vi "Laser Spectroscopy.vi"() -> ()   [LabVIEW 2014]
uses:
  Control 3.ctl
  Control 4.ctl
  Source Cluster.ctl
  MoCo Source Code LabView 2013/global_m.vi
  <instrlib>/Tektronix DPO 7104/Tektronix 7000 Series/Public/Configure/Configure Trigger (Edge).vi
  <instrlib>/Tektronix DPO 7104/Tektronix 7000 Series/Public/Data/Read (Single Waveform).vi
  <vilib>/NI/GXML/Generator.vi
  <vilib>/NI/GXML/Write XML to File.vi
  <vilib>/Utility/file.llb/Write To Spreadsheet File (DBL).vi
  <instrlib>/Tektronix 7000 Series/Tektronix 7000 Series.lvlib
  C8855-01api.dll
panel:
  out "Waveform Graph C8855":waveform(dbl)(graph)
  out "Refnum out":refnum<k7> caption="Mono RefNum out"
  out "XY Graph":cluster{"Wavelength":dbl[], "Int WF":dbl[]}(graph)
  in  "Reinitialise to default values":bool
  out "Waveform Graph":waveform(dbl)(graph)
  in  "Tab Control":T1(tab)
  out "state":dbl
  in  "Target Grating":u16(ring)=1 items=["1200", "600", "300"]
  in  "Clear data array":bool
  in  "Abort Scan":bool
  in  "Operator's Name":string="Operator"
  in  "File Format":enum16{"XML", "CSV"}(ring)
  in  "Log Data":bool
  in  "Path":path
  in  "Backward":bool
  in  "Forward":bool
  in  "Scan Mode":enum32{"Interrupted ", "Uninterrupted"}(radio)=enum."Uninterrupted"
  in  "Scan":bool
  in  "Target WL":bool
  in  "End Wavelength":dbl=572.0
  in  "Delay (s)":dbl
  in  "Interval Wavelength":dbl=0.1
  in  "Start Wavelength":dbl=882.0
  in  "Target WL":dbl=882.7202
  in  "Exit Mirror":u16(ring)=2 caption="Target Position Exit Mirror" items=["Front"=2, "Side"=3]
  in  "Entrance Mirror":u16(ring)=2 caption="Target Position\nEntrance Mirror" items=["Front"=2, "Side"=3]
  in  "Target  Exit":dbl
  in  "Target\nFront Entrance":dbl
  out "Current Grating":dbl=1200.0
  out "Grating Index":i32=1
  out "Current Description":string="1" caption="Description"
  in  "Mono ID":string(combo)="Mono4"
  out "Current UniqueID":string="Mono4"
  out "Current WL":dbl=897.9988
  out "Exit":dbl
  out "Unit":string="mm"
  out "Front Entrance":dbl
  out "Unit":string="mm"
  out "Exit Mirror\nPosition":i32(ring)=2 items=["EntranceMirror", "ExitMirror", "Front", "Side"]
  out "Entrance Mirror\nPosition":i32(ring)=2 items=["EntranceMirror", "ExitMirror", "Front", "Side"]
  in  "Force\nInitialization":bool
  out "Unit":string="nm"
  in  "Connect":bool
  out "iHR550 Error Bundle":errorcluster
  out "Emulating":bool
  out "Initialized":bool
  out "Status":string
  out "error out":errorcluster
  out "source out 2":string
  out "code out":i32 format="%0.0f"
  out "Gratings":dbl[](array[numeric])=[1200.0, 300.0]
  out "Current Blaze":string
  out "Medium Loop":T2
  out "DPO7104":T3=enum."Initial Settings"
  in  "stop":bool
  in  "Close Session":bool
  in  "Initialize":bool caption="Push at the start"
  in  "Auto Calibration:":bool
  in  "Save GL302 Settings":bool
  in  "Backlash Compensation":bool
  in  "Calibration":bool
  in  "Set speed":bool
  in  "stop 2":bool
  in  "fs":bool
  in  "bs":bool
  in  "FW":bool
  in  "BW":bool
  in  "Pause":dbl
  in  "Abort Scan GL302":bool
  in  "Step":dbl
  in  "Scan GL302":bool
  in  "End Wavelength":dbl min=-20.0 max=1100.0
  in  "Start Wavelength":dbl min=-20.0 max=1100.0
  in  "Target Wavelength":bool
  in  "Calibration, nm":dbl=587.2
  in  "Destination Wavelength":dbl min=-20.0 max=1100.0 format="%.3f"
  in  "Grating, gr/mm":u16(ring)=2 items=["2400", "1800", "1200", "600", "300", "150"]
  in  "delay before read (ms)":u32=100
  in  "Scan Mode":enum32{"Interrupted ", "Uninterrupted"}(radio)=enum."Uninterrupted"
  out "Present Wavelength":dbl=479.168125 format="%.3f"
  in  "Wavelength, nm":dbl format="%.3f"
  in  "Speed":dbl=5.0 format="%.3f"
  out "R number":i32
  in  "Backlash Compensation":dbl=0.01 format="%.3f"
  out "GL302 Initialization":errorcluster
  out "Communication Port":refnum<visa-resource-name>
  out "Status":string
  in  "shutdown":bool
  in  "stop curving":bool
  in  "Integrate":bool=TRUE
  out "CURV?":bool
  in  "Channel (0: Channel 1)":u16(ring)=1 format="%#_5f" items=["Channel 1", "Channel 2", "Channel 3", "Channel 4", "Math 1", "Math 2", "Math 3", "Math 4", "Reference 1", "Reference 2", "Reference 3", "Reference 4"]
  in  "AUTOSET":bool
  in  "Delay Time":dbl
  in  "Delay":bool
  in  "# of Averages":u32=16
  in  "Acquisition Mode":enum16{"Sample", "Average", "Hi Res"}(ring)=enum."Average"
  in  "Probe Attenuation (10.0)":dbl=1.0 step=0.5
  in  "Vertical Coupling (1: DC)":u16(ring)=1 items=["AC", "DC", "Ground"]
  in  "Trigger Level (0.0)":dbl=0.08
  in  "Input Impedance":u16(ring)=1 items=["1M", "50"]
  in  "Bandwidth (0: FULL)":u16(ring) items=["FULL", "500 MHz", "250 MHz", "150 MHz", "20 MHz"]
  in  "Delay Position":u32
  in  "Vertical Position":dbl step=0.5
  in  "Vertical Offset (0.0 V)":dbl
  in  "Position (0.0 s)":dbl=10.0
  in  "Coupling (0:DC)":u16(ring)=1 items=["DC", "AC", "Hf Reject", "Lf Reject", "Noise Rej", "Atrigger"]
  in  "Trigger Event (0:A Event)":u16(ring) items=["A Event", "B Event"]
  in  "Slope (0:Rise)":u16(ring) items=["Rise", "Fall", "Either"]
  in  "Source (0:Channel1)":u16(ring) items=["Channel1"=0, "Channel2"=1, "Channel3"=2, "Channel4"=3, "Aux"=12, "Line"=13, "Digital Channel0"=14, "Digital Channel1"=15, "Digital Channel2"=16, "Digital Channel3"=17, "Digital Channel4"=18, "Digital Chennel5"=19, "Digital Channel6"=20, "Digital Channel7"=21, "Digital Channel8"=22, "Digital Channel9"=23, "Digital Channel10"=24, "Digital Channel11"=25, "Digital Channel12"=26, "Digital Channel13"=27, "Digital Channel14"=28, "Digital Channel15"=29]
  in  "VISA resource name":refnum<visa-resource-name>="TEKSCOPE-A4EC42"
  out "Number of Acquisitions":u32
  out "Area":dbl
  out "Unit":string
  in  "file path":path
  in  "Save waveform":bool
  out "Saved":bool
  out "Main":errorcluster
  out "Cursors":errorcluster
  out "source out":string
  out "User-driven Event Struct":errorcluster
  out "code out":i32 format="%0.0f"
  in  "Horizontal Modes":enum16{"Constant", "Manual", "Auto"}(ring)=enum."Auto"
  in  "Record Length (10000)":u32=10000 caption="Record Length (10000s)"
  out "Acquisition Length":dbl
  out "Sample Rate":dbl
  out "Time/Div.":dbl
  out "Volt/Div.":dbl
  out "Acquisition Duration":dbl
  in  "Number of Averages":u32
  in  "Average":bool
  in  "Measure":bool
  in  "Monitor":bool
  in  "Close C8855":bool
  out "C8855 Initialised":bool
  in  "Measurement points":u32=30
  in  "C8855 gate time":i32(ring) caption="Gate time" items=["50 us", "100 us", "200 us", "500 us", "1 ms", "2 ms", "5 ms", "10 ms", "20 ms", "50 ms", "100 ms", "200 ms", "500 ms", "1 s", "2 s", "5 s", "10 s"]
  in  "Triggers":enum32{"Software", "External"}(radio)
  out "code out 2":i32 format="%0.0f"
  out "source out 3":string
  out "error out 2":errorcluster
  out "Counts":u32
  out "Measurement Time (sec)":dbl
  out "time step":dbl
  out "status":T3=enum."Initial Settings"
  out "Handle":i32
  out "Result Returned":u8
  out "iterations":i32
  out "Numeric":i32
  in  "wait between function nodes in averaging mode (ms)":u32=10
  in  "Horizontal Scale":u32(knob)=30 scale=0.0..44.0
  in  "Sampling Rate":u32(knob)=17 scale=0.0..29.0
  in  "Vertical Scale":u32(knob)=27 scale=0.0..36.0
  in  "Vertical Range (10.0 V)":dbl=10.0
  in  "L Cursor 2":dbl(slide)=3.9682539682539764e-05 min=-0.020000000000000004 max=0.18 step=0.001 scale=-0.020000000000000004..0.18
  in  "R Cursor 2":dbl(slide)=0.008058730158730161 min=-0.020000000000000004 max=0.18 step=0.001 scale=-0.020000000000000004..0.18
  out "delta t":dbl
  out "R Cursor":dbl
  out "L Cursor":dbl
  in  "T Cursor":dbl(slide) min=-5.0 max=5.0 step=0.2 scale=-5.0..5.0
  in  "B Cursor":dbl(slide) min=-5.0 max=5.0 step=0.2 scale=-5.0..5.0
  out "delta V":dbl
  out "B Cursor":dbl
  out "T Cursor":dbl
  in  "Cursor Type":enum16{"Vertical", "Horizontal", "Screen"}(ring)
  in  "Snap":bool
  in  "Cursor ON/OFF":bool
  in  "Vertical Cursor Style":i32=3 min=0 max=3 step=1
  in  "Horizontal Cursor Style":i32
  out "Cursors Error Status":bool
  # "Press until \"Saved\" light is on"
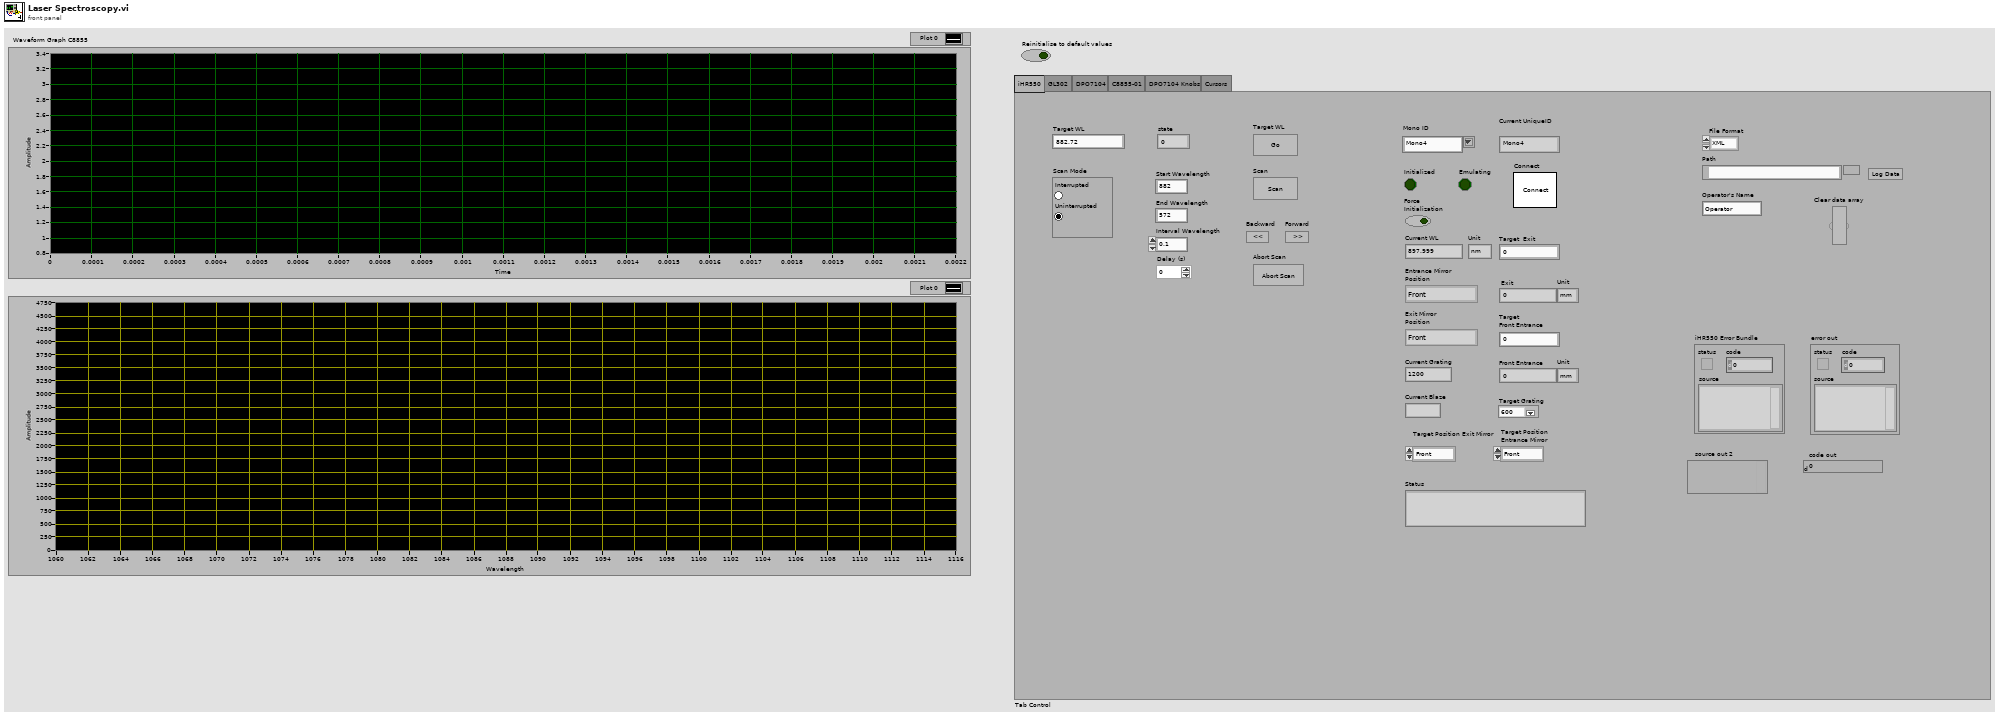
[diagram p1: front panel]
types:
  T1 = enum32{"iHR550", "GL302", "DPO7104", "C8855-01", "DPO7104 Knobs", "Cursors"}
  T2 = typedef "Control 3.ctl" = enum16{"Idle", "iHR550 Initial Settings", "iHR550 Front Entrance ", "iHR550 Front Exit", "iHR550 Gratings", "iHR550 Fixed Wavelength", "iHR550 Interval Movement", "GL302 Settings", "GL302 Goto WL", "GL302 Step Movement", "GL302 scan", "Log Data", "Error Handler", "Close Session"}
  T3 = typedef "Control 4.ctl" = enum16{"Stop ", "Waveform Queries", "Idle", "Initial Settings", "Ver/Hor Queries", "Trigger", "AUTOSET", "Delay", "Acquisition Mode", "Time Settings", "Channel Settings", "Error Handler", "C8855-Reset", "C8855-Measurement Setup", "C8855-Count Start", "C8855-Data Update", "C8855-Close", "C8855-Count Stop", "C8855-Monitor", "C8855-ECreO"}
  T4 = cluster{"Name":string, "Color":i32, "Style":i32, "Point Style":i32, "Name Visible":bool, "Allow Drag":bool, "Cursor Mode":i32, "Plot":i32, "Index":i32, "Position":cluster{"X":dbl, "Y":dbl}, "X Scale":i32, "Y Scale":i32, "Watch Plots":i32[], "Watch All Plots":bool, "Plot Area":i32, "Label Offset":cluster{"X":dbl, "Y":dbl}}
  T5 = cluster{"Operator's Name":string, "Start Wavelength":dbl, "End Wavelength":dbl, "Interval Wavelength":dbl, "Delay":dbl, "Date":string, "Time":string, "Data":cluster{"Wavelength":dbl[], "Int WF":dbl[]}}
  T6 = typedef "Source Cluster.ctl" = cluster{"VISA resource name":refnum<visa-resource-name>, "error in (no error)":errorcluster, "Spec Plot":cluster{"Wavelength":dbl[], "Int WF":dbl[]}, "C8855 Measurement Parameters":cluster{"Gate time":u8, "Number of Gates":u16, "Number of measurements":i32, "Number of blocks":i32, "For AVG":dbl[][]}, "Data Buffer":u32[]}
  T7 = cluster{"Name":string, "Color":i32, "Style":i32, "Point Style":i32, "Name Visible":bool, "Allow Drag":bool, "Cursor Mode":i32, "Plot":i32, "Index":i32, "Position":cluster{"X":dbl, "Y":dbl}, "X Scale":i32, "Y Scale":i32, "Watch Plots":i32[], "Watch All Plots":bool, "Plot Area":i32, "Label Offset":cluster{"X":dbl, "Y":dbl}}[]
  T8 = cluster{"Gate time":u8, "Number of Gates":u16, "Number of measurements":i32, "Number of blocks":i32, "For AVG":dbl[][]}
  T9 = cluster{"Gate time":u8, "Number of gates":u16, "Number of measurements":i32, "Number of blocks":i32, "Array":u32[][]}
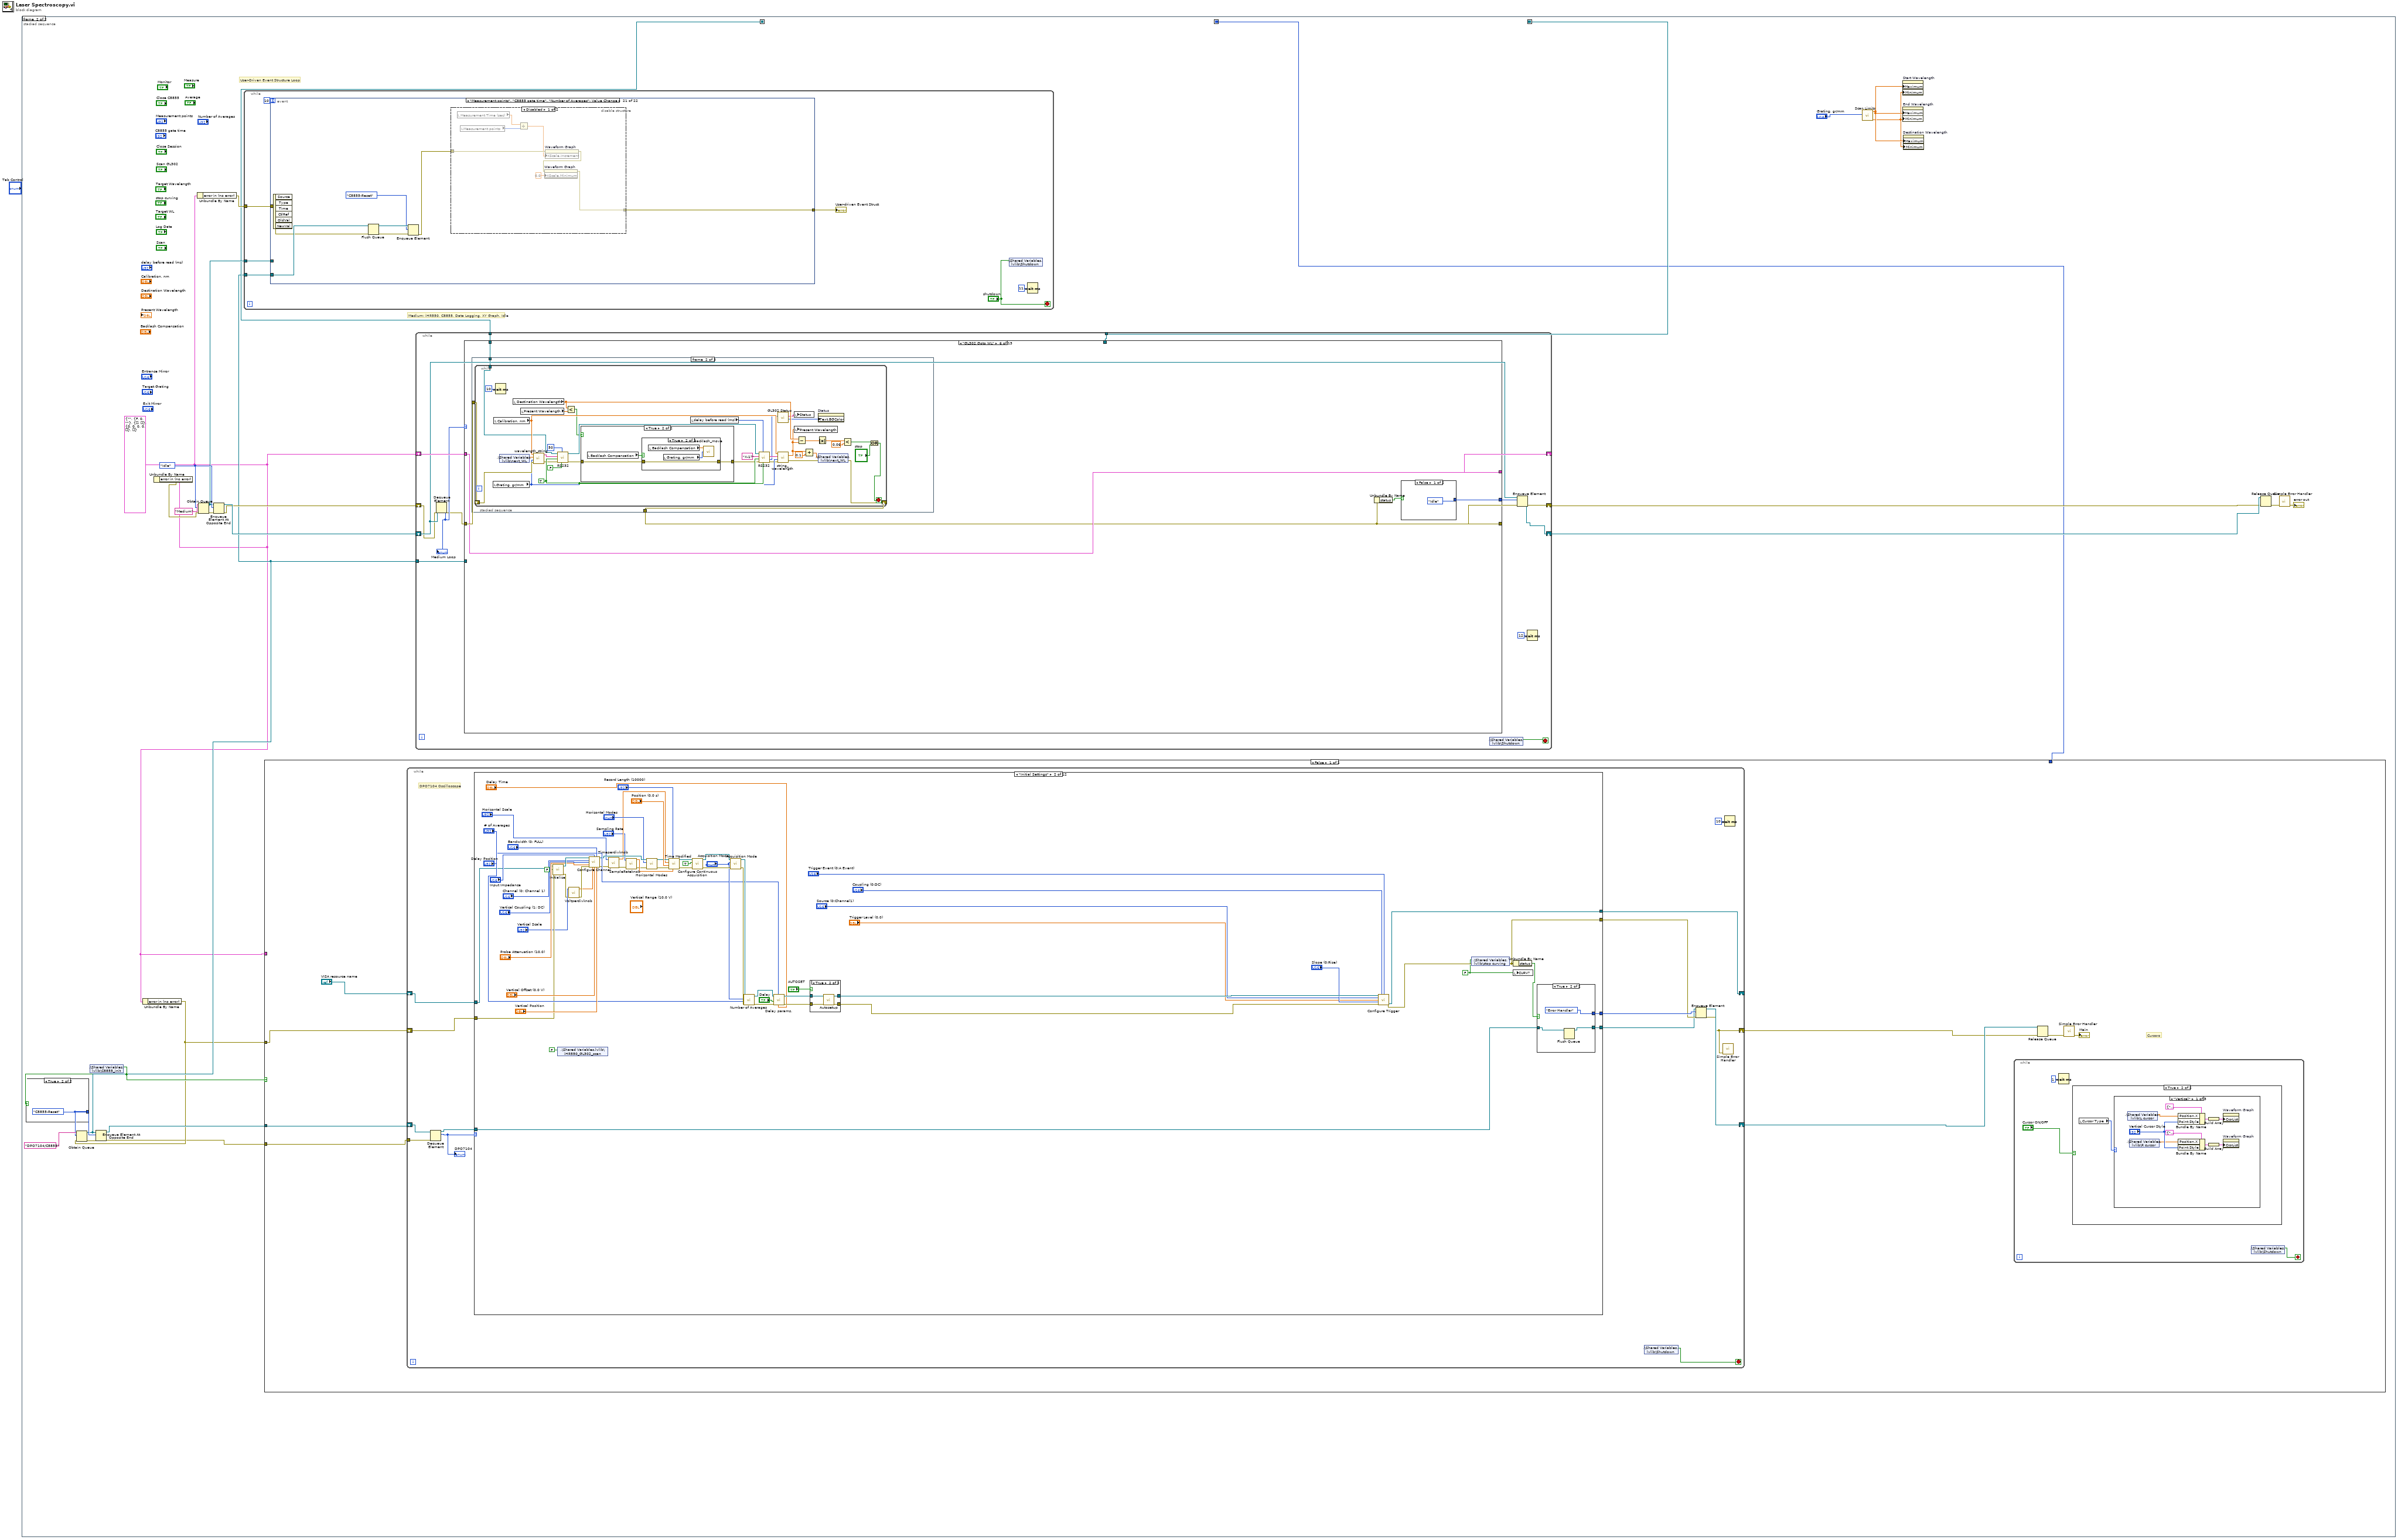
[diagram p0: block diagram]
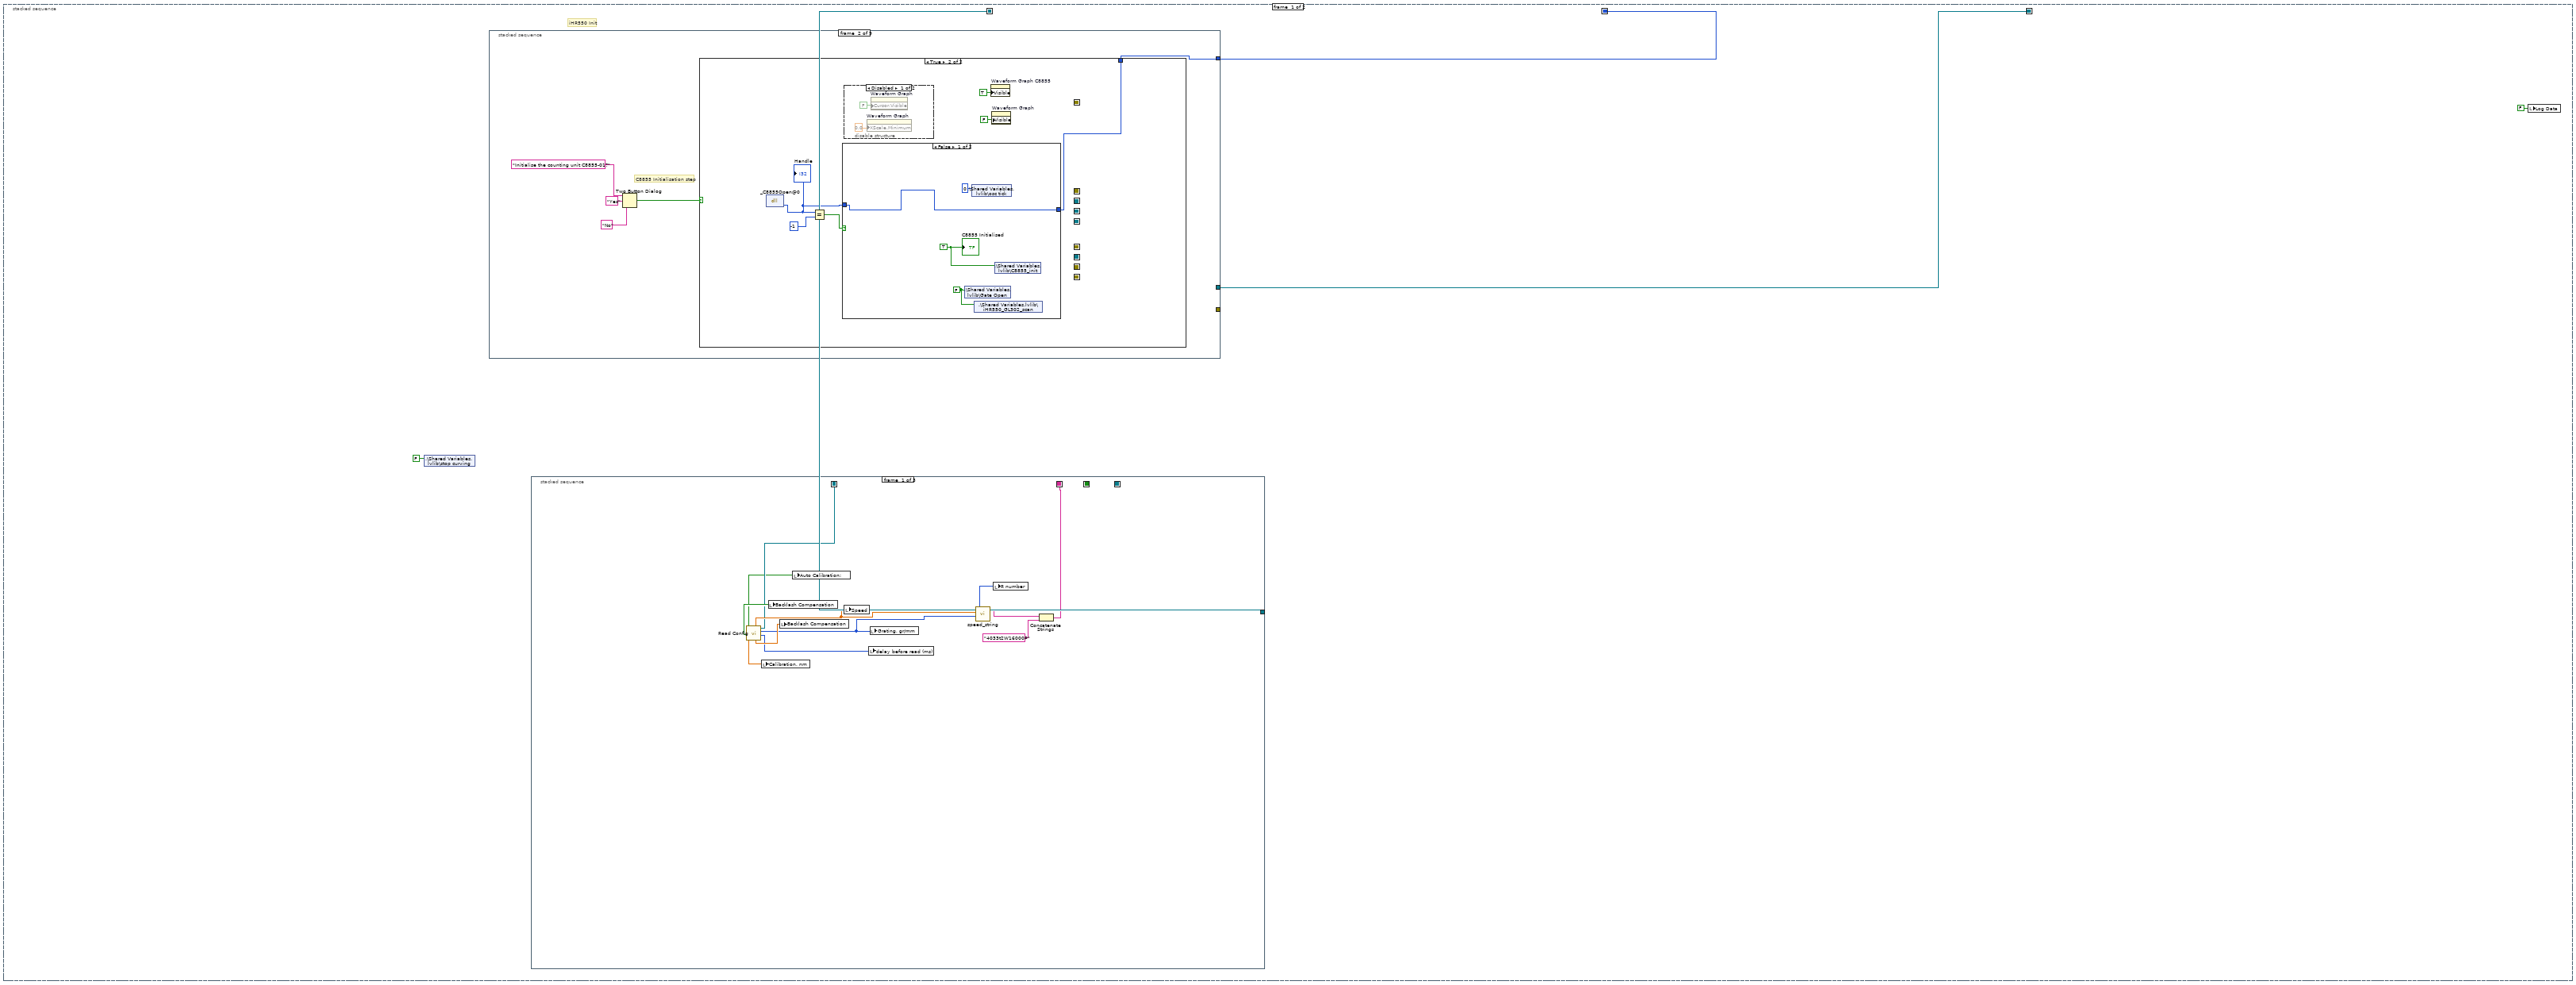
[diagram p2: hidden frame]
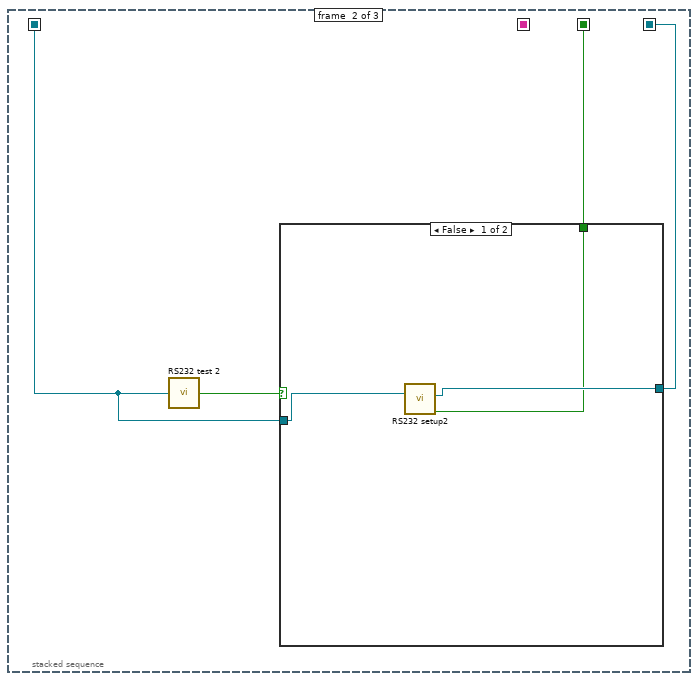
[diagram p3: hidden frame]
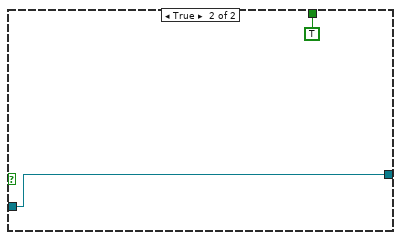
[diagram p4: hidden frame]
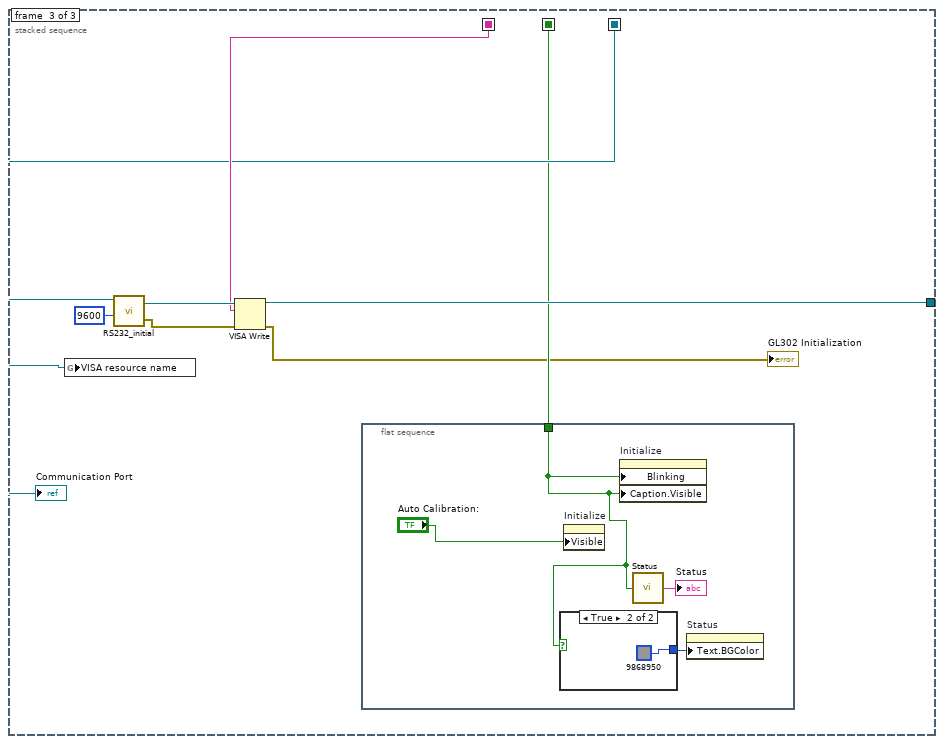
[diagram p5: hidden frame]
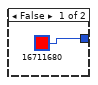
[diagram p6: hidden frame]
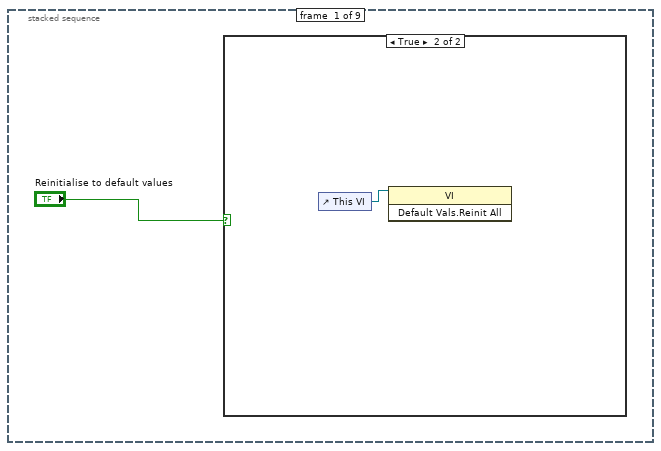
[diagram p7: hidden frame]
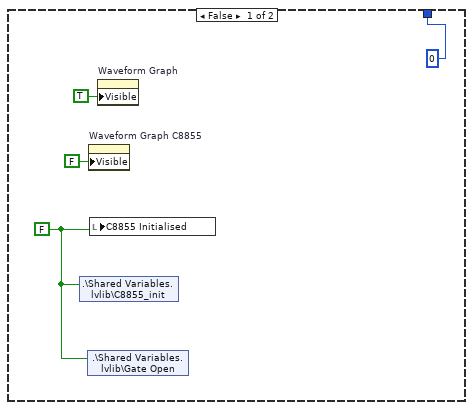
[diagram p9: hidden frame]
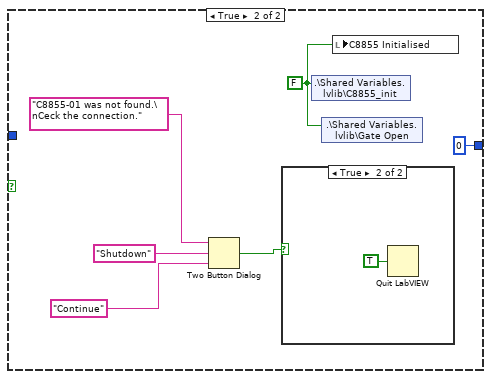
[diagram p11: hidden frame]
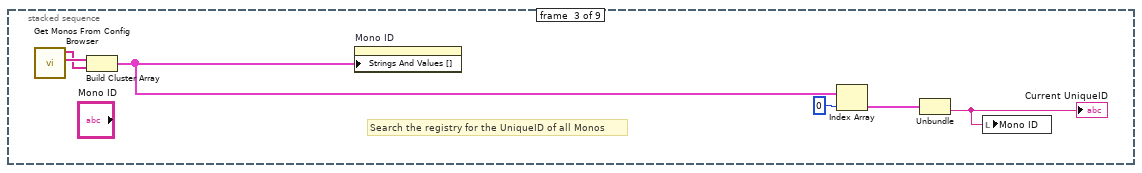
[diagram p13: hidden frame]
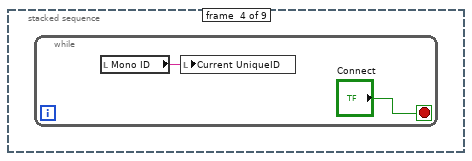
[diagram p14: hidden frame]
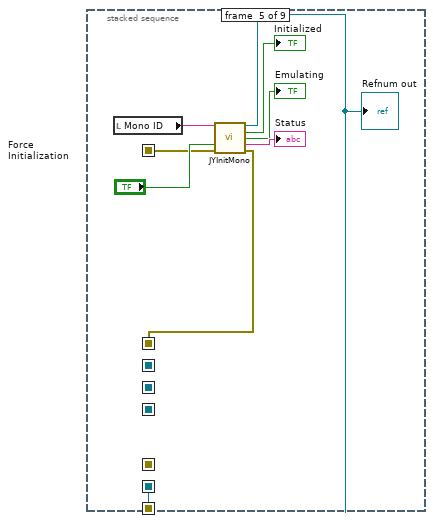
[diagram p15: hidden frame]
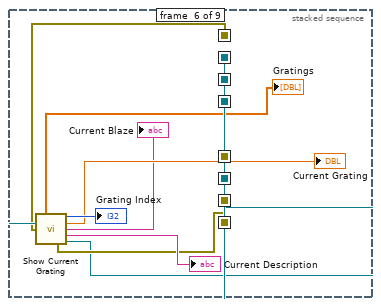
[diagram p16: hidden frame]
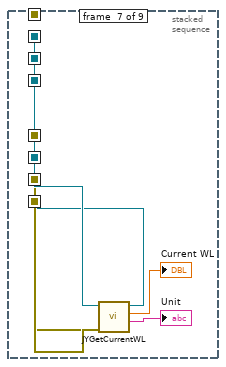
[diagram p17: hidden frame]
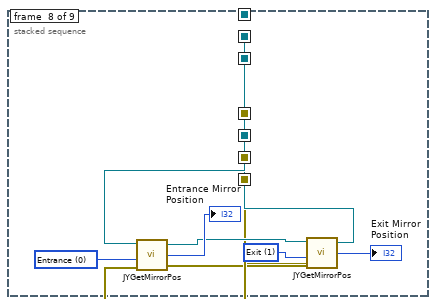
[diagram p18: hidden frame]
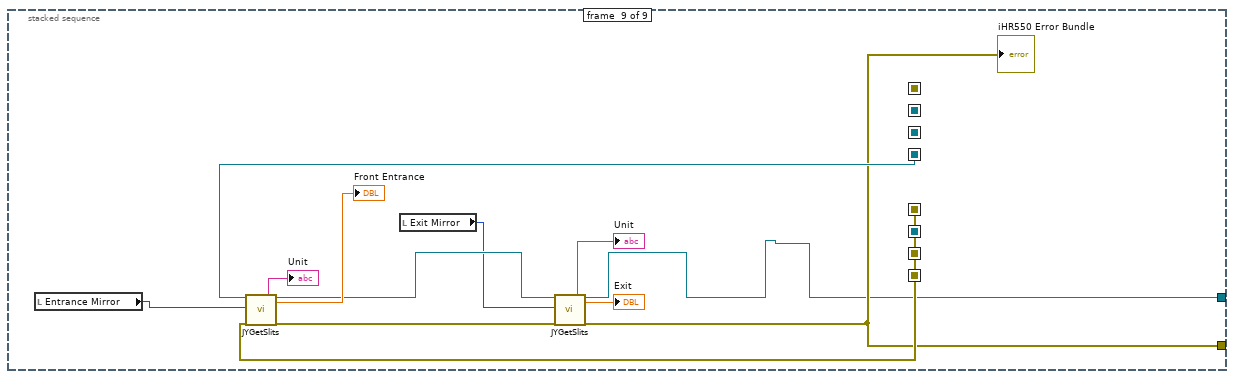
[diagram p19: hidden frame]
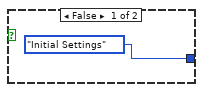
[diagram p20: hidden frame]
diagram:
  n1 = stacked-sequence {
    seq-local: [w4 _] -> [_ w143]
    seq-local: [w2 _] -> [_ w136]
    seq-local: [w1 _] -> [_ w124]
    frame #0 {
      # "iHR550 Init"
      n2 = shared-variable ".\\Shared Variables.lvlib\\stop curving"(FALSE ("Stop Curving")) -> ()  [unwired: 1 in, 1 out]
      n3 = stacked-sequence {
        seq-local: [_ _ _ _ w79 _ _ _ _] -> [_ _ _ _ _ _ _ _ _]
        seq-local: [_ _ _ _ w79 _ _ _ _] -> [_ _ _ _ _ w87 _ _ _]
        seq-local: [_ _ _ _ w82 _ _ _ _] -> [_ _ _ _ _ w92 _ _ _]
        seq-local: [_ _ _ _ _ w91 _ _ _] -> [_ _ _ _ _ _ w97 _ _]
        seq-local: [_ _ _ _ _ w90 _ _ _] -> [_ _ _ _ _ _ w98 _ _]
        seq-local: [_ _ _ _ _ _ w96 _ _] -> [_ _ _ _ _ _ _ w103 _]
        seq-local: [_ _ _ _ _ _ w95 _ _] -> [_ _ _ _ _ _ _ w106 _]
        seq-local: [_ _ _ _ _ _ _ w104 _] -> [_ _ _ _ _ _ _ _ w116]
        seq-local: [_ _ _ _ _ _ _ w101 _] -> [_ _ _ _ _ _ _ _ w115]
        tunnel: [_ _ _ _ _ _ _ _ w114] -> _
        tunnel: [_ _ _ _ _ _ _ _ w113] -> w4
        tunnel: [_ w43 _ _ _ _ _ _ _] -> w1
        frame #0 {
          n4 = case shown="True" "Reinitialise to default values" {
            frame False {
            }
            frame True {
              n5 = control-ref of="This VI"() -> (w42:refnum<vi>)
              n6 = invoke class="VI" method="Default Vals.Reinit All"(reference=w42) -> ()  [unwired: 2 in, 3 out]
            }
          }
        }
        frame #1 {
          # "C8855 Initialisation step"
          n7 = Two Button Dialog(message="Initialise the counting unit C8855-01?", 1:"No" ("F button name (\"Cancel\")"), 2:"Yes" ("T button name (\"OK\")")) -> (T button?=w47:bool)
          n8 = case shown="True" w47 {
            tunnel: [0 ("Handle") w57] -> w43
            frame False {
              w51 = FALSE ("C8855 Initialised")
              n9 = shared-variable ".\\Shared Variables.lvlib\\C8855_init"(w51) -> ()  [unwired: 1 in, 1 out]
              n10 = shared-variable ".\\Shared Variables.lvlib\\Gate Open"(w51) -> ()  [unwired: 1 in, 1 out]
              n11 = property on="Waveform Graph C8855" class="WFGraph (strict)"("Visible"=FALSE) -> ()  [unwired: 2 in, 2 out]
              n12 = local write "C8855 Initialised"(w51) -> ()
              n13 = property on="Waveform Graph" class="WFGraph (strict)"("Visible"=TRUE) -> ()  [unwired: 2 in, 2 out]
            }
            frame True {
              n14 = dll-call lib="C:/Users/physrin/Documents/LSLV/Labview Laser Spectroscopy/C8855-01api.dll" fn="_C8855Open@0"() -> ("Handle"=w56:i32)  [unwired: 3 in, 2 out]
              "Handle" <- w56
              n15 = Equal?(x=w56, y=-1) -> (x = y?=w55:bool)
              n16 = case shown="False" w55 {
                tunnel: w56 -> [w60 _]
                tunnel: [w60 0 ("Handle")] -> w57
                frame False {
                  w62 = FALSE ("Gate Open")
                  w63 = TRUE ("C8855 Initialised")
                  n17 = shared-variable ".\\Shared Variables.lvlib\\Gate Open"(w62) -> ()  [unwired: 1 in, 1 out]
                  n18 = shared-variable ".\\Shared Variables.lvlib\\osc tick"(u32 0 ("osc tick")) -> ()  [unwired: 1 in, 1 out]
                  n19 = shared-variable ".\\Shared Variables.lvlib\\iHR550_GL302_scan"(w62) -> ()  [unwired: 1 in, 1 out]
                  n20 = shared-variable ".\\Shared Variables.lvlib\\C8855_init"(w63) -> ()  [unwired: 1 in, 1 out]
                  "C8855 Initialised" <- w63
                }
                frame True {
                  w64 = FALSE ("C8855_init")
                  n21 = Two Button Dialog(message="C8855-01 was not found.\nCeck the connection.", 1:"Continue" ("F button name (\"Cancel\")"), 2:"Shutdown" ("T button name (\"OK\")")) -> (T button?=w66:bool)
                  n22 = case shown="True" w66 {
                    frame False {
                    }
                    frame True {
                      n23 = Quit LabVIEW(quit? (T)=TRUE) -> ()
                    }
                  }
                  n24 = shared-variable ".\\Shared Variables.lvlib\\C8855_init"(w64) -> ()  [unwired: 1 in, 1 out]
                  n25 = shared-variable ".\\Shared Variables.lvlib\\Gate Open"(w64) -> ()  [unwired: 1 in, 1 out]
                  n26 = local write "C8855 Initialised"(w64) -> ()
                }
              }
              n27 = disable-structure shown="Disabled" {
                frame Disabled {
                  n28 = property on="Waveform Graph" class="WFGraph (strict)"("XScale.Minimum"=0.0 ("X Scale.Range:Minimum")) -> ()  [unwired: 2 in, 2 out]
                  n29 = property on="Waveform Graph" class="WFGraph (strict)"("Cursor.Visible"=FALSE) -> ()  [unwired: 2 in, 2 out]
                }
                frame Enabled {
                }
              }
              n30 = property on="Waveform Graph C8855" class="WFGraph (strict)"("Visible"=TRUE) -> ()  [unwired: 2 in, 2 out]
              n31 = property on="Waveform Graph" class="WFGraph (strict)"("Visible"=FALSE) -> ()  [unwired: 2 in, 2 out]
            }
          }
        }
        frame #2 {
          # "Search the registry for the UniqueID of all Monos"
          n32 = call "Get Monos From Config Browser.vi"() -> ("UniqueIDs"=w71:string[], "Mono ID"=w72:string[])  [unwired: 3 in, 1 out]
          n33 = Build Cluster Array(w72, w71) -> (w76:cluster{"String":string, "String":string}[])
          n34 = property on="Mono ID" class="CmbBox"("Strings And Values []"=w76) -> ()  [unwired: 2 in, 2 out]
          n35 = Index Array(array=w76, index=0) -> (element=w74:cluster{"String":string, "String":string})
          n36 = Unbundle(w74) -> ("String"=w73:string)  [unwired: 1 out]
          "Current UniqueID" <- w73
          n37 = local write "Mono ID"(w73) -> ()
        }
        frame #3 {
          n38 = while {
            stop <- "Connect" stop-if-true
            n39 = local read "Mono ID"() -> (w78:string)
            n40 = local write "Current UniqueID"(w78) -> ()
          }
        }
        frame #4 {
          n41 = local read "Mono ID"() -> (w80:string)
          n42 = call "JYInitMono.vi"("Unique ID"=w80, "Force Init"="Force\nInitialization") -> ("Refnum out"=w82:refnum<k7>, "Initialized"=→"Initialized":bool, "Emulating"=→"Emulating":bool, "Status"=→"Status":string, "error out"=w79:errorcluster)  [unwired: 9 in]
          "Refnum out" <- w82
        }
        frame #5 {
          n43 = call "Show Current Grating.vi"("Refnum in"=w92, "error in (no error)"=w87) -> ("Gratings"=→"Gratings":dbl[], "Grating Index"=→"Grating Index":i32, "Current Grating"=→"Current Grating":dbl, "Current Blaze"=→"Current Blaze":string, "Current Description"=→"Current Description":string, "error out"=w91:errorcluster, "JYMONOLib.IJYMonoReqd"=w90:refnum<k7>)  [unwired: 5 in, 2 out]
        }
        frame #6 {
          n44 = call "JYGetCurrentWL.vi"("error in (no error)"=w97, "JYMONOLib.IJYMonoReqd"=w98) -> ("error out"=w96:errorcluster, "Units"=→"Unit":string, "Current WL"=→"Current WL":dbl, "JYMONOLib.IJYMonoReqd 2"=w95:refnum<k7>)  [unwired: 5 in, 1 out]
        }
        frame #7 {
          w107 = u16 1 items=["Entrance", "Exit"] ("Mirror")
          w108 = u16 0 items=["Entrance", "Exit"] ("Mirror")
          n45 = call "JYGetMirrorPos.vi"("error in (no error)"=w103, "Mirror"=w108, "Refnum In"=w106) -> ("error out"=w102:errorcluster, "Current Mirror Position"=→"Entrance Mirror\nPosition":i32, "Refnum Out"=w105:refnum<k7>)  [unwired: 1 in]
          n46 = call "JYGetMirrorPos.vi"("error in (no error)"=w102, "Mirror"=w107, "Refnum In"=w105) -> ("error out"=w101:errorcluster, "Current Mirror Position"=→"Exit Mirror\nPosition":i32, "Refnum Out"=w104:refnum<k7>)  [unwired: 1 in]
        }
        frame #8 {
          n47 = local read "Entrance Mirror"() -> (w112:u16)
          n48 = call "JYGetSlits.vi"("MonoRefNum IN"=w116, "Slit"=w112, "error in (no error)"=w115) -> ("Units"=→"Unit":string, "MonoRefNum Out"=w117:refnum<k7>, "Slit Width"=→"Front Entrance":dbl, "error out"=w118:errorcluster)  [unwired: 13 in]
          n49 = local read "Exit Mirror"() -> (w111:u16)
          n50 = call "JYGetSlits.vi"("MonoRefNum IN"=w117, "Slit"=w111, "error in (no error)"=w118) -> ("Units"=→"Unit":string, "MonoRefNum Out"=w113:refnum<k7>, "Slit Width"=→"Exit":dbl, "error out"=w114:errorcluster)  [unwired: 13 in]
          "iHR550 Error Bundle" <- w114
        }
      }
      n51 = stacked-sequence {
        seq-local: [w9 _ _] -> [_ w20 _]
        seq-local: [w7 _ _] -> [_ _ w32]
        seq-local: [_ w19 _] -> [_ _ w30]
        seq-local: [_ w18 _] -> [_ _ w28]
        tunnel: [_ _ w29] -> w2
        frame #0 {
          n52 = call "Read Config.vi"() -> ("Delay Before read (ms)"=w14:u32, "Grating, gr/mm"=w12:u16, "VISA resource name"=w9:refnum<visa-resource-name>, "Backlash compensation"=w16:dbl, "Speed"=w13:dbl, "Calibration, nm"=w15:dbl, "Backlash"=w17:bool, "Auto Calibration:"=w6:bool)  [unwired: 4 out]
          n53 = local write "Calibration, nm"(w15) -> ()
          n54 = local write "Backlash Compensation"(w17) -> ()
          n55 = local write "Backlash Compensation"(w16) -> ()
          n56 = local write "Auto Calibration:"(w6) -> ()
          n57 = local write "Speed"(w13) -> ()
          n58 = local write "delay before read (ms)"(w14) -> ()
          n59 = local write "Grating, gr/mm"(w12) -> ()
          n60 = call "speed_string.vi"("Grating, gr/mm"=w12, "Speed"=w13) -> ("nm_String"=w10:string, "R number"=w11:i32)  [unwired: 1 in, 1 out]
          n61 = local write "R number"(w11) -> ()
          n62 = Concatenate Strings(w10, "4033t2W16000P") -> (w7:string)
        }
        frame #1 {
          n63 = call "RS232 test 2.vi"("VISA resource name"=w20) -> ("RS Communication:"=w21:bool)  [unwired: 4 in]
          n64 = case shown="False" w21 {
            tunnel: w20 -> [w24 w26]
            tunnel: [w23 w26] -> w19
            tunnel: [w22 TRUE ("Status:")] -> w18
            frame False {
              n65 = call "RS232 setup2.vi"("PC Port"=w24) -> ("Status:"=w22:bool, "PC Port out"=w23:refnum<visa-resource-name>)  [unwired: 9 in]
            }
            frame True {
            }
          }
        }
        frame #2 {
          n66 = global write "global_m.vi" "VISA resource name"(w30) -> ()
          n67 = call "RS232_initial.vi"("baud rate"=u32 9600, "VISA resource name"=w30) -> ("error out"=w31:errorcluster, "VISA name out"=w33:refnum<visa-resource-name>)  [unwired: 2 in]
          n68 = VISA Write(VISA resource name=w33, write buffer=w32, error in (no error)=w31) -> (VISA resource name out=w29:refnum<visa-resource-name>, error out=→"GL302 Initialization":errorcluster)  [unwired: 1 out]
          n69 = flat-sequence {
            tunnel: w28 -> [w36]
            frame #0 {
              n70 = case shown="True" w36 {
                tunnel: [u32 16711680 u32 9868950] -> w35
                frame False {
                }
                frame True {
                }
              }
              n71 = property on="Initialize" class="Bool (strict)"("Visible"="Auto Calibration:") -> ()  [unwired: 2 in, 2 out]
              n72 = property on="Initialize" class="Bool (strict)"("Blinking"=w36, "Caption.Visible"=w36) -> ()  [unwired: 2 in, 2 out]
              n73 = call "Status.vi"("Status"=w36) -> ("String"=→"Status":string)
              n74 = property on="Status" class="Str"("Text.BGColor"=w35) -> ()  [unwired: 2 in, 2 out]
            }
          }
          "Communication Port" <- w30
        }
      }
      n75 = local write "Log Data"(FALSE ("Log Data")) -> ()
    }
    frame #1 {
      w147 = Control_3."Idle"
      w123 = T6 {"VISA resource name"="", "error in (no error)"={"status"=FALSE, "code"=0, "source"=""}, "Spec Plot"={"Wavelength"=[], "Int WF"=[]}, "C8855 Measurement Parameters"={"Gate time"=0, "Number of Gates"=0, "Number of measurements"=0, "Number of blocks"=0, "For AVG"=[]}, "Data Buffer"=[]}
      # "Medium: iHR550, C8855, Data Logging, XY Graph, Idle"
      # "User-Driven Event Structure Loop"
      n76 = shared-variable ".\\Shared Variables.lvlib\\C8855_init"() -> (w129:bool)  [unwired: 1 in, 1 out]
      n77 = case shown="True" w129 {
        tunnel: [Control_4."Initial Settings" ("Enum") Control_4."C8855-Reset" ("Enum")] -> w131
        frame False {
        }
        frame True {
        }
      }
      n78 = Unbundle By Name(w123) -> ("error in (no error)"=w126:errorcluster)
      n79 = Obtain Queue(name (unnamed)="DPO7104/C8855", element data type=w131, error in (no error)=w126) -> (queue out=w130:refnum<queue>, error out=w127:errorcluster)  [unwired: 2 in, 1 out]
      n80 = Enqueue Element At Opposite End(queue=w130, element=w131, error in (no error)=w127) -> (queue out=w128:refnum<queue>, error out=w125:errorcluster)  [unwired: 1 in, 1 out]
      n81 = Unbundle By Name(w123) -> ("error in (no error)"=w141:errorcluster)
      n82 = Unbundle By Name(w123) -> ("error in (no error)"=w137:errorcluster)
      n83 = Obtain Queue(name (unnamed)="Medium", element data type=w147, error in (no error)=w141) -> (queue out=w144:refnum<queue>, error out=w148:errorcluster)  [unwired: 2 in, 1 out]
      n84 = Enqueue Element At Opposite End(queue=w144, element=w147, error in (no error)=w148) -> (queue out=w146:refnum<queue>, error out=w138:errorcluster)  [unwired: 1 in, 1 out]
      n85 = while {
        tunnel: w130 -> [w2324]
        tunnel: w144 -> [w2323]
        tunnel: w137 -> [w2320]
        stop <- "shutdown" stop-if-true
        n86 = event shown="[20] \"Measurement points\", \"C8855 gate time\", \"Number of Averages\": Value Change" {
          selector: _ -> [_ _ _ _ _ _ _ _ _ _ _ _ _ _ _ _ _ _ _ _ _ _]
          dyn-events: _ -> [_ _ _ _ _ _ _ _ _ _ _ _ _ _ _ _ _ _ _ _ _ _]
          timeout: 10 -> [_ _ _ _ _ _ _ _ _ _ _ _ _ _ _ _ _ _ _ _ _ _]
          tunnel: w2324 -> [_ _ _ w2345 _ _ _ w2371 _ _ _ w2392 w2407 _ w2435 w2443 w2451 w2459 w2467 w2473 w2480 w2496]
          tunnel: w2323 -> [_ w2331 w2337 _ w2351 w2357 w2363 _ w2377 w2383 w2389 w2398 w2414 w2427 _ _ _ _ _ _ _ _]
          tunnel: [w2325 w2327 w2333 w2340 w2347 w2352 w2358 w2366 w2372 w2378 w2384 w2394 w2411 w2422 w2430 w2438 w2446 w2454 w2462 w2468 w2474 w2490] -> w2321
          tunnel: w2320 -> [w2325 w2329 w2335 w2343 w2349 w2354 w2360 w2368 w2374 w2380 w2386 w2391 w2409 w2424 w2433 w2441 w2449 w2457 w2465 w2472 w2477 w2495]
          event Timeout {
            n87 = event-data() -> ()  [unwired: 1 in, 3 out]
          }
          event "Target\nFront Entrance": Value Change {
            n88 = event-data() -> ()  [unwired: 1 in, 2 out]
            n89 = Flush Queue(queue=w2331, error in (no error)=w2329) -> (queue out=w2330:refnum<queue>, error out=w2328:errorcluster)  [unwired: 1 out]
            n90 = Enqueue Element(queue=w2330, element=Control_3."iHR550 Front Entrance ", error in (no error)=w2328) -> (error out=w2327:errorcluster)  [unwired: 1 in, 2 out]
          }
          event "Target  Exit": Value Change {
            n91 = event-data() -> ()  [unwired: 1 in, 6 out]
            n92 = Flush Queue(queue=w2337, error in (no error)=w2335) -> (queue out=w2336:refnum<queue>, error out=w2334:errorcluster)  [unwired: 1 out]
            n93 = Enqueue Element(queue=w2336, element=Control_3."iHR550 Front Exit", error in (no error)=w2334) -> (error out=w2333:errorcluster)  [unwired: 1 in, 2 out]
          }
          event "stop curving": Value Change {
            w2339 = TRUE ("Stop Curving")
            n94 = event-data() -> ()  [unwired: 1 in, 6 out]
            n95 = Flush Queue(queue=w2345, error in (no error)=w2343) -> (queue out=w2344:refnum<queue>, error out=w2342:errorcluster)  [unwired: 1 out]
            n96 = Enqueue Element(queue=w2344, element=Control_4."Stop " ("Enum"), error in (no error)=w2342) -> (error out=w2341:errorcluster)  [unwired: 1 in, 2 out]
            n97 = shared-variable ".\\Shared Variables.lvlib\\stop curving"(w2339, error in=w2341) -> (error out=w2340:errorcluster)
            "CURV?" <- w2339
          }
          event "Target Grating": Value Change {
            n98 = event-data() -> ()  [unwired: 1 in, 6 out]
            n99 = Flush Queue(queue=w2351, error in (no error)=w2349) -> (queue out=w2350:refnum<queue>, error out=w2348:errorcluster)  [unwired: 1 out]
            n100 = Enqueue Element(queue=w2350, element=Control_3."iHR550 Gratings", error in (no error)=w2348) -> (error out=w2347:errorcluster)  [unwired: 1 in, 2 out]
          }
          event "Set speed", "Calibration", "Save GL302 Settings", "Initialize": Value Change {
            n101 = event-data() -> ()  [unwired: 1 in, 6 out]
            n102 = Flush Queue(queue=w2357, error in (no error)=w2354) -> (queue out=w2356:refnum<queue>, error out=w2353:errorcluster)  [unwired: 1 out]
            n103 = Enqueue Element(queue=w2356, element=Control_3."GL302 Settings", error in (no error)=w2353) -> (error out=w2352:errorcluster)  [unwired: 1 in, 2 out]
          }
          event "Close Session": Value Change {
            n104 = event-data() -> ()  [unwired: 1 in, 6 out]
            n105 = Flush Queue(queue=w2363, error in (no error)=w2360) -> (queue out=w2362:refnum<queue>, error out=w2359:errorcluster)  [unwired: 1 out]
            n106 = Enqueue Element(queue=w2362, element=Control_3."Close Session", error in (no error)=w2359) -> (error out=w2358:errorcluster)  [unwired: 1 in, 2 out]
          }
          event "Vertical Coupling (1: DC)", "Probe Attenuation (10.0)", "Input Impedance", "Bandwidth (0: FULL)", "Vertical Position", "Vertical Offset (0.0 V)", "Channel (0: Channel 1)", "Vertical Scale": Value Change {
            w2365 = TRUE ("Stop Curving")
            n107 = event-data() -> ()  [unwired: 1 in, 1 out]
            n108 = Flush Queue(queue=w2371, error in (no error)=w2368) -> (queue out=w2370:refnum<queue>, error out=w2369:errorcluster)  [unwired: 1 out]
            n109 = Enqueue Element(queue=w2370, element=Control_4."Channel Settings" ("Enum"), error in (no error)=w2369) -> (error out=w2367:errorcluster)  [unwired: 1 in, 2 out]
            n110 = shared-variable ".\\Shared Variables.lvlib\\stop curving"(w2365, error in=w2367) -> (error out=w2366:errorcluster)
            n111 = local write "CURV?"(w2365) -> ()
          }
          event "Target WL": Value Change {
            n112 = event-data() -> ()  [unwired: 1 in, 6 out]
            n113 = Flush Queue(queue=w2377, error in (no error)=w2374) -> (queue out=w2376:refnum<queue>, error out=w2373:errorcluster)  [unwired: 1 out]
            n114 = Enqueue Element(queue=w2376, element=Control_3."iHR550 Fixed Wavelength", error in (no error)=w2373) -> (error out=w2372:errorcluster)  [unwired: 1 in, 2 out]
          }
          event "Target Wavelength": Value Change {
            n115 = event-data() -> ()  [unwired: 1 in, 6 out]
            n116 = Flush Queue(queue=w2383, error in (no error)=w2380) -> (queue out=w2382:refnum<queue>, error out=w2379:errorcluster)  [unwired: 1 out]
            n117 = Enqueue Element(queue=w2382, element=Control_3."GL302 Goto WL", error in (no error)=w2379) -> (error out=w2378:errorcluster)  [unwired: 1 in, 2 out]
          }
          event "bs", "stop 2", "fs": Value Change {
            n118 = event-data() -> ()  [unwired: 1 in, 6 out]
            n119 = Flush Queue(queue=w2389, error in (no error)=w2386) -> (queue out=w2388:refnum<queue>, error out=w2385:errorcluster)  [unwired: 1 out]
            n120 = Enqueue Element(queue=w2388, element=Control_3."GL302 Step Movement", error in (no error)=w2385) -> (error out=w2384:errorcluster)  [unwired: 1 in, 2 out]
          }
          event "Scan": Value Change {
            n121 = event-data() -> ()  [unwired: 1 in, 6 out]
            n122 = shared-variable ".\\Shared Variables.lvlib\\C8855_init"() -> (w2393:bool)  [unwired: 1 in, 1 out]
            n123 = case shown="True" w2393 {
              tunnel: w2392 -> [_ w2405]
              tunnel: w2391 -> [w2399 w2402]
              tunnel: [w2399 w2400] -> w2390
              frame False {
              }
              frame True {
                n124 = Flush Queue(queue=w2405, error in (no error)=w2402) -> (queue out=w2404:refnum<queue>, error out=w2401:errorcluster)  [unwired: 1 out]
                n125 = Enqueue Element(queue=w2404, element=Control_4."C8855-Count Start" ("Enum"), error in (no error)=w2401) -> (error out=w2400:errorcluster)  [unwired: 1 in, 2 out]
              }
            }
            n126 = Flush Queue(queue=w2398, error in (no error)=w2390) -> (queue out=w2397:refnum<queue>, error out=w2395:errorcluster)  [unwired: 1 out]
            n127 = Enqueue Element(queue=w2397, element=Control_3."iHR550 Interval Movement", error in (no error)=w2395) -> (error out=w2394:errorcluster)  [unwired: 1 in, 2 out]
          }
          event "Scan GL302": Value Change {
            n128 = event-data() -> ()  [unwired: 1 in, 6 out]
            n129 = shared-variable ".\\Shared Variables.lvlib\\C8855_init"() -> (w2406:bool)  [unwired: 1 in, 1 out]
            n130 = case shown="True" w2406 {
              tunnel: w2409 -> [w2415 w2421]
              tunnel: [w2415 w2419] -> w2408
              tunnel: w2407 -> [_ w2418]
              frame False {
              }
              frame True {
                n131 = Flush Queue(queue=w2418, error in (no error)=w2421) -> (queue out=w2417:refnum<queue>, error out=w2420:errorcluster)  [unwired: 1 out]
                n132 = Enqueue Element(queue=w2417, element=Control_4."C8855-Count Start" ("Enum"), error in (no error)=w2420) -> (error out=w2419:errorcluster)  [unwired: 1 in, 2 out]
              }
            }
            n133 = Flush Queue(queue=w2414, error in (no error)=w2408) -> (queue out=w2413:refnum<queue>, error out=w2412:errorcluster)  [unwired: 1 out]
            n134 = Enqueue Element(queue=w2413, element=Control_3."GL302 scan", error in (no error)=w2412) -> (error out=w2411:errorcluster)  [unwired: 1 in, 2 out]
          }
          event "Log Data": Value Change {
            n135 = event-data() -> ()  [unwired: 1 in, 6 out]
            n136 = Flush Queue(queue=w2427, error in (no error)=w2424) -> (queue out=w2426:refnum<queue>, error out=w2423:errorcluster)  [unwired: 1 out]
            n137 = Enqueue Element(queue=w2426, element=Control_3."Log Data", error in (no error)=w2423) -> (error out=w2422:errorcluster)  [unwired: 1 in, 2 out]
          }
          event "Delay Time", "Delay", "Delay Position": Value Change {
            w2429 = TRUE ("Stop Curving")
            n138 = event-data() -> ()  [unwired: 1 in, 6 out]
            n139 = Flush Queue(queue=w2435, error in (no error)=w2433) -> (queue out=w2434:refnum<queue>, error out=w2432:errorcluster)  [unwired: 1 out]
            n140 = Enqueue Element(queue=w2434, element=Control_4."Delay" ("Enum"), error in (no error)=w2432) -> (error out=w2431:errorcluster)  [unwired: 1 in, 2 out]
            n141 = shared-variable ".\\Shared Variables.lvlib\\stop curving"(w2429, error in=w2431) -> (error out=w2430:errorcluster)
            n142 = local write "CURV?"(w2429) -> ()
          }
          event "AUTOSET": Value Change {
            w2437 = TRUE ("Stop Curving")
            n143 = event-data() -> ()  [unwired: 1 in, 6 out]
            n144 = Flush Queue(queue=w2443, error in (no error)=w2441) -> (queue out=w2442:refnum<queue>, error out=w2440:errorcluster)  [unwired: 1 out]
            n145 = Enqueue Element(queue=w2442, element=Control_4."AUTOSET" ("Enum"), error in (no error)=w2440) -> (error out=w2439:errorcluster)  [unwired: 1 in, 2 out]
            n146 = shared-variable ".\\Shared Variables.lvlib\\stop curving"(w2437, error in=w2439) -> (error out=w2438:errorcluster)
            n147 = local write "CURV?"(w2437) -> ()
          }
          event "Trigger Level (0.0)", "Coupling (0:DC)", "Trigger Event (0:A Event)", "Slope (0:Rise)", "Source (0:Channel1)": Value Change {
            w2445 = TRUE ("Stop Curving")
            n148 = event-data() -> ()  [unwired: 1 in, 6 out]
            n149 = Flush Queue(queue=w2451, error in (no error)=w2449) -> (queue out=w2450:refnum<queue>, error out=w2448:errorcluster)  [unwired: 1 out]
            n150 = Enqueue Element(queue=w2450, element=Control_4."Trigger" ("Enum"), error in (no error)=w2448) -> (error out=w2447:errorcluster)  [unwired: 1 in, 2 out]
            n151 = shared-variable ".\\Shared Variables.lvlib\\stop curving"(w2445, error in=w2447) -> (error out=w2446:errorcluster)
            n152 = local write "CURV?"(w2445) -> ()
          }
          event "Horizontal Scale", "Position (0.0 s)", "Record Length (10000)", "Horizontal Modes", "Sampling Rate": Value Change {
            w2453 = TRUE ("Stop Curving")
            n153 = event-data() -> ()  [unwired: 1 in, 6 out]
            n154 = Flush Queue(queue=w2459, error in (no error)=w2457) -> (queue out=w2458:refnum<queue>, error out=w2456:errorcluster)  [unwired: 1 out]
            n155 = Enqueue Element(queue=w2458, element=Control_4."Time Settings" ("Enum"), error in (no error)=w2456) -> (error out=w2455:errorcluster)  [unwired: 1 in, 2 out]
            n156 = shared-variable ".\\Shared Variables.lvlib\\stop curving"(w2453, error in=w2455) -> (error out=w2454:errorcluster)
            n157 = local write "CURV?"(w2453) -> ()
          }
          event "Acquisition Mode", "# of Averages": Value Change {
            w2461 = TRUE ("Stop Curving")
            n158 = event-data() -> ()  [unwired: 1 in, 6 out]
            n159 = Flush Queue(queue=w2467, error in (no error)=w2465) -> (queue out=w2466:refnum<queue>, error out=w2464:errorcluster)  [unwired: 1 out]
            n160 = Enqueue Element(queue=w2466, element=Control_4."Acquisition Mode" ("Enum"), error in (no error)=w2464) -> (error out=w2463:errorcluster)  [unwired: 1 in, 2 out]
            n161 = shared-variable ".\\Shared Variables.lvlib\\stop curving"(w2461, error in=w2463) -> (error out=w2462:errorcluster)
            n162 = local write "CURV?"(w2461) -> ()
          }
          event "Close C8855": Value Change {
            n163 = event-data() -> ()  [unwired: 1 in, 6 out]
            n164 = Flush Queue(queue=w2473, error in (no error)=w2472) -> (queue out=w2470:refnum<queue>, error out=w2471:errorcluster)  [unwired: 1 out]
            n165 = Enqueue Element(queue=w2470, element=Control_4."C8855-Close" ("Enum"), error in (no error)=w2471) -> (error out=w2468:errorcluster)  [unwired: 1 in, 2 out]
          }
          event "Measurement points", "C8855 gate time", "Number of Averages": Value Change {
            n166 = event-data() -> ()  [unwired: 1 in, 6 out]
            n167 = Flush Queue(queue=w2480, error in (no error)=w2477) -> (queue out=w2479:refnum<queue>, error out=w2476:errorcluster)  [unwired: 1 out]
            n168 = Enqueue Element(queue=w2479, element=Control_4."C8855-Reset" ("Enum"), error in (no error)=w2476) -> (error out=w2475:errorcluster)  [unwired: 1 in, 2 out]
            n169 = disable-structure shown="Disabled" {
              disable-tunnel: w2475 -> [w2487 w2488]
              disable-tunnel: [w2485 w2488] -> w2474
              frame Disabled {
                n170 = local read "Measurement Time (sec)"() -> (w2484:dbl)
                n171 = local read "Measurement points"() -> (w2483:u32)
                n172 = Divide(x=w2484, y=w2483) -> (x/y=w2482:dbl)
                n173 = property on="Waveform Graph" class="WFGraph (strict)"(error in=w2487, "XScale.Increment"=w2482) -> (error out=w2486:errorcluster)  [unwired: 1 in, 1 out]
                n174 = property on="Waveform Graph" class="WFGraph (strict)"(error in=w2486, "XScale.Minimum"=0.0 ("X Scale.Range:Minimum")) -> (error out=w2485:errorcluster)  [unwired: 1 in, 1 out]
              }
              frame Enabled {
              }
            }
          }
          event "Monitor": Value Change {
            n175 = event-data() -> ()  [unwired: 1 in, 6 out]
            n176 = Flush Queue(queue=w2496, error in (no error)=w2495) -> (queue out=w2493:refnum<queue>, error out=w2494:errorcluster)  [unwired: 1 out]
            n177 = Enqueue Element(queue=w2493, element=Control_4."C8855-Monitor" ("Enum"), error in (no error)=w2494) -> (error out=w2491:errorcluster)  [unwired: 1 in, 2 out]
            n178 = local read "Monitor"() -> (w2489:bool)
            n179 = case shown="False" w2489 {
              tunnel: w2491 -> [w2499 w2502]
              tunnel: [w2498 w2501] -> w2490
              frame False {
                n180 = property on="Monitor" class="Bool (strict)"(error in=w2499, "BoolText.Text"="Monitor" ("Boolean Text.Text")) -> (error out=w2498:errorcluster)  [unwired: 1 in, 1 out]
              }
              frame True {
                n181 = property on="Monitor" class="Bool (strict)"(error in=w2502, "BoolText.Text"="Stop Monitoring" ("Boolean Text.Text")) -> (error out=w2501:errorcluster)  [unwired: 1 in, 1 out]
              }
            }
          }
        }
        "User-driven Event Struct" <- w2321
        n182 = shared-variable ".\\Shared Variables.lvlib\\Shutdown"("shutdown") -> ()  [unwired: 1 in, 1 out]
        n183 = Wait (ms)(milliseconds to wait=u32 11) -> ()  [unwired: 1 out]
      }
      n184 = case shown="False" w129 {
        tunnel: w128 -> [w154 w591]
        tunnel: w126 -> [w153 w588]
        tunnel: w125 -> [w152 w590]
        tunnel: w124 -> [_ _]
        tunnel: w123 -> [_ w589]
        frame False {
          # "Cursors"
          n185 = while {
            tunnel: w152 -> [w202]
            shift-right: [w211] -> w159
            shift-left: w154 -> [w212]
            shift-right: [w208] -> _
            shift-left: "VISA resource name" -> [w207]
            shift-right: [w203] -> w155
            shift-left: w153 -> [w213]
            stop <- w200 stop-if-true
            # "DPO7104 Oscilloscope"
            n186 = Dequeue Element(queue=w212, error in (no error)=w202) -> (queue out=w205:refnum<queue>, element=w201:T3)  [unwired: 1 in, 2 out]
            "DPO7104" <- w201
            n187 = case shown="\"Initial Settings\"" w201 {
              tunnel: w207 -> [w219 w253 w318 w332 w365 w372 w399 w425 w449 w461 w566 w582]
              tunnel: w213 -> [w218 w252 w302 w330 w364 w371 w395 w424 w448 w460 w568 w581]
              tunnel: [w219 w251 w317 w345 w362 w383 w398 w423 w446 w456 w566 w582] -> w208
              tunnel: [w218 w249 w316 w341 w357 w378 w394 w416 w437 w458 w562 w578] -> w209
              tunnel: [w216 w247 w306 w339 w355 w376 w392 w414 w435 w457 w565 Control_4."Idle" ("Enum")] -> w210
              tunnel: w205 -> [w215 w232 w303 w336 w352 w373 w389 w411 w432 w455 w563 w576]
              tunnel: [w214 w231 w304 w337 w353 w374 w390 w412 w433 w455 w564 w577] -> w204
              frame "Idle", Default {
                n188 = Unbundle By Name(w218) -> ("status"=w217:bool)
                n189 = case shown="False" w217 {
                  tunnel: [Control_4."Idle" ("Enum") Control_4."Error Handler" ("Enum")] -> w216
                  tunnel: w215 -> [w222 w225]
                  tunnel: [w221 w224] -> w214
                  frame False {
                    n190 = Flush Queue(queue=w222) -> (queue out=w221:refnum<queue>)  [unwired: 1 in, 2 out]
                  }
                  frame True {
                    n191 = Flush Queue(queue=w225) -> (queue out=w224:refnum<queue>)  [unwired: 1 in, 2 out]
                  }
                }
              }
              frame "Initial Settings" {
                w246 = FALSE ("stop curving")
                n192 = call <instrlib>:"Initialize.vi"("error in (no error)"=w252, "Reset? ( Yes)"=FALSE, "VISA resource name"=w253) -> ("error out"=w229:errorcluster, "VISA resource name out"=w283:refnum<visa-resource-name>)  [unwired: 7 in]
                n193 = shared-variable ".\\Shared Variables.lvlib\\iHR550_GL302_scan"(FALSE ("iHR550_GL302_scan")) -> ()  [unwired: 1 in, 1 out]
                n194 = call "Voltperdivknob.vi"("error in (no error)"=w229, "Dial"="Vertical Scale") -> ("error out"=w228:errorcluster, "Volt/Div."=w227:dbl)  [unwired: 8 in]
                n195 = call <instrlib>:"Configure Channel.vi"("VISA resource name"=w283, "Input Impedance (0: 1M ohm)"="Input Impedance", "Bandwidth (0: FULL)"="Bandwidth (0: FULL)", "Channel (0: Channel 1)"="Channel (0: Channel 1)", "Vertical Coupling (1: DC)"="Vertical Coupling (1: DC)", "Probe Attenuation (1.0)"="Probe Attenuation (10.0)", "error in (no error)"=w228, "Vertical Range (10.0 V)"=w227, "Vertical Offset (0.0 V)"="Vertical Offset (0.0 V)", "Vertical Position"="Vertical Position") -> ("VISA resource name out"=w244:refnum<visa-resource-name>, "error out"=w238:errorcluster)  [unwired: 4 in]
                n196 = call "Timeperdivknob.vi"("Dial"="Horizontal Scale", "error in (no error)"=w238) -> ("Time/Div."=w239:dbl, "error out"=w235:errorcluster)  [unwired: 5 in]
                n197 = call "SampleRateknob.vi"("Dial"="Sampling Rate", "error in (no error)"=w235) -> ("Sampling Rate"=w236:dbl, "error out"=w234:errorcluster)  [unwired: 5 in]
                n198 = call "Horizontal Modes.vi"("error in (no error)"=w234, "Hor modes"="Horizontal Modes", "VISA Refnum in"=w244) -> ("error out"=w242:errorcluster, "VISA Refnum out"=w243:refnum<visa-resource-name>)  [unwired: 7 in]
                n199 = call <instrlib>:"Time Modified.vi"("Sampling Rate"=w236, "Record Length (10000)"="Record Length (10000)", "error in (no error)"=w242, "Position (0.0 s)"="Position (0.0 s)", "Horizontal Scale"=w239, "VISA resource name"=w243) -> ("error out"=w245:errorcluster, "VISA resource name out"=w282:refnum<visa-resource-name>)  [unwired: 4 in]
                n200 = call <instrlib>:"Configure Continuous Acquisition.vi"("error in (no error)"=w245, "Enable Continuous Acquisition Mode (True)"=TRUE, "VISA resource name"=w282) -> ("error out"=w286:errorcluster, "VISA resource name out"=w281:refnum<visa-resource-name>)  [unwired: 7 in]
                n201 = call <instrlib>:"Acquisition Mode.vi"("error in (no error)"=w286, "Acq Mode"="Acquisition Mode", "VISA resource name"=w281) -> ("error out"=w266:errorcluster, "VISA resource name out"=w268:refnum<visa-resource-name>)  [unwired: 7 in]
                n202 = call <instrlib>:"Number of Averages.vi"("error in (no error)"=w266, "# of Averages"="# of Averages", "Acq Mode"="Acquisition Mode", "VISA resource name"=w268) -> ("error out"=w265:errorcluster, "VISA resource name out"=w267:refnum<visa-resource-name>)  [unwired: 6 in]
                n203 = call <instrlib>:"Delay params..vi"("Delay Time"="Delay Time", "Delay Position"="Delay Position", "error in (no error)"=w265, "selector"="Delay", "VISA resource name"=w267) -> ("error out"=w285:errorcluster, "VISA resource name out"=w280:refnum<visa-resource-name>)  [unwired: 5 in]
                n204 = case shown="True" "AUTOSET" {
                  tunnel: w285 -> [w294 w298]
                  tunnel: [w294 w297] -> w284
                  tunnel: w280 -> [w293 w296]
                  tunnel: [w293 w295] -> w279
                  frame False {
                  }
                  frame True {
                    n205 = call <instrlib>:"Autosetup.vi"("error in (no error)"=w298, "VISA resource name"=w296) -> ("error out"=w297:errorcluster, "VISA resource name out"=w295:refnum<visa-resource-name>)  [unwired: 8 in]
                  }
                }
                n206 = call-poly <instrlib>:"Configure Trigger.vi"("VISA resource name"=w279, "Coupling (0:DC)"="Coupling (0:DC)", "Trigger Event (0:A Event)"="Trigger Event (0:A Event)", "Source (0:Channel1)"="Source (0:Channel1)", "Trigger Level (0.0V)"="Trigger Level (0.0)", "Slope (0:Rise)"="Slope (0:Rise)", "error in (no error)"=w284) -> ("VISA resource name out"=w251:refnum<visa-resource-name>, "error out"=w250:errorcluster)  [unwired: 7 in]
                n207 = shared-variable ".\\Shared Variables.lvlib\\stop curving"(w246, error in=w250) -> (error out=w249:errorcluster)
                n208 = Unbundle By Name(w249) -> ("status"=w248:bool)
                n209 = local write "CURV?"(w246) -> ()
                n210 = case shown="True" w248 {
                  tunnel: [Control_4."Ver/Hor Queries" ("Enum") Control_4."Error Handler" ("Enum")] -> w247
                  tunnel: w232 -> [w289 w292]
                  tunnel: [w288 w291] -> w231
                  frame False {
                    n211 = Flush Queue(queue=w289) -> (queue out=w288:refnum<queue>)  [unwired: 1 in, 2 out]
                  }
                  frame True {
                    n212 = Flush Queue(queue=w292) -> (queue out=w291:refnum<queue>)  [unwired: 1 in, 2 out]
                  }
                }
              }
              frame "Channel Settings" {
                w305 = FALSE ("stop curving")
                n213 = local read "Probe Attenuation (10.0)"() -> (w311:dbl)
                n214 = local read "Channel (0: Channel 1)"() -> (w312:u16)
                n215 = local read "Vertical Coupling (1: DC)"() -> (w313:u16)
                n216 = local read "Vertical Offset (0.0 V)"() -> (w310:dbl)
                n217 = local read "Input Impedance"() -> (w314:u16)
                n218 = local read "Vertical Position"() -> (w309:dbl)
                n219 = local read "Bandwidth (0: FULL)"() -> (w315:u16)
                n220 = local read "Vertical Scale"() -> (w300:u32)
                n221 = call "Voltperdivknob.vi"("error in (no error)"=w302, "Dial"=w300) -> ("error out"=w301:errorcluster, "Volt/Div."=w299:dbl)  [unwired: 8 in]
                n222 = call <instrlib>:"Configure Channel.vi"("VISA resource name"=w318, "Input Impedance (0: 1M ohm)"=w314, "Bandwidth (0: FULL)"=w315, "Channel (0: Channel 1)"=w312, "Vertical Coupling (1: DC)"=w313, "Probe Attenuation (1.0)"=w311, "error in (no error)"=w301, "Vertical Range (10.0 V)"=w299, "Vertical Offset (0.0 V)"=w310, "Vertical Position"=w309) -> ("VISA resource name out"=w317:refnum<visa-resource-name>, "error out"=w308:errorcluster)  [unwired: 4 in]
                n223 = Unbundle By Name(w308) -> ("status"=w307:bool)
                n224 = local write "CURV?"(w305) -> ()
                n225 = shared-variable ".\\Shared Variables.lvlib\\stop curving"(w305, error in=w308) -> (error out=w316:errorcluster)
                n226 = case shown="True" w307 {
                  tunnel: [Control_4."Ver/Hor Queries" ("Enum") Control_4."Error Handler" ("Enum")] -> w306
                  tunnel: [w320 w324] -> w304
                  tunnel: w303 -> [w321 w323]
                  frame False {
                    n227 = Flush Queue(queue=w321) -> (queue out=w320:refnum<queue>)  [unwired: 1 in, 2 out]
                  }
                  frame True {
                    n228 = Flush Queue(queue=w323) -> (queue out=w324:refnum<queue>)  [unwired: 1 in, 2 out]
                  }
                }
              }
              frame "Time Settings" {
                w338 = FALSE ("stop curving")
                n229 = local read "Horizontal Modes"() -> (w333:enum16{"Constant", "Manual", "Auto"})
                n230 = local read "Horizontal Scale"() -> (w335:u32)
                n231 = local read "Sampling Rate"() -> (w328:u32)
                n232 = local read "Record Length (10000)"() -> (w343:u32)
                n233 = call "Horizontal Modes.vi"("error in (no error)"=w330, "Hor modes"=w333, "VISA Refnum in"=w332) -> ("error out"=w329:errorcluster, "VISA Refnum out"=w331:refnum<visa-resource-name>)  [unwired: 7 in]
                n234 = local read "Position (0.0 s)"() -> (w342:dbl)
                n235 = call "Timeperdivknob.vi"("Dial"=w335, "error in (no error)"=w329) -> ("Time/Div."=w334:dbl, "error out"=w326:errorcluster)  [unwired: 5 in]
                n236 = call "SampleRateknob.vi"("Dial"=w328, "error in (no error)"=w326) -> ("Sampling Rate"=w327:dbl, "error out"=w325:errorcluster)  [unwired: 5 in]
                n237 = call <instrlib>:"Time Modified.vi"("Sampling Rate"=w327, "Record Length (10000)"=w343, "error in (no error)"=w325, "Position (0.0 s)"=w342, "Horizontal Scale"=w334, "VISA resource name"=w331) -> ("error out"=w344:errorcluster, "VISA resource name out"=w345:refnum<visa-resource-name>)  [unwired: 4 in]
                n238 = shared-variable ".\\Shared Variables.lvlib\\stop curving"(w338, error in=w344) -> (error out=w341:errorcluster)
                n239 = local write "CURV?"(w338) -> ()
                n240 = Unbundle By Name(w341) -> ("status"=w340:bool)
                n241 = case shown="True" w340 {
                  tunnel: [Control_4."Ver/Hor Queries" ("Enum") Control_4."Error Handler" ("Enum")] -> w339
                  tunnel: [w348 w351] -> w337
                  tunnel: w336 -> [w347 w350]
                  frame False {
                    n242 = Flush Queue(queue=w347) -> (queue out=w348:refnum<queue>)  [unwired: 1 in, 2 out]
                  }
                  frame True {
                    n243 = Flush Queue(queue=w350) -> (queue out=w351:refnum<queue>)  [unwired: 1 in, 2 out]
                  }
                }
              }
              frame "Acquisition Mode" {
                w354 = FALSE ("stop curving")
                n244 = local read "# of Averages"() -> (w358:u32)
                n245 = local read "Acquisition Mode"() -> (w359:enum16{"Sample", "Average", "Hi Res"})
                n246 = call <instrlib>:"Number of Averages.vi"("error in (no error)"=w364, "# of Averages"=w358, "Acq Mode"=w359, "VISA resource name"=w365) -> ("error out"=w361:errorcluster, "VISA resource name out"=w363:refnum<visa-resource-name>)  [unwired: 6 in]
                n247 = call <instrlib>:"Acquisition Mode.vi"("error in (no error)"=w361, "Acq Mode"=w359, "VISA resource name"=w363) -> ("error out"=w360:errorcluster, "VISA resource name out"=w362:refnum<visa-resource-name>)  [unwired: 7 in]
                n248 = shared-variable ".\\Shared Variables.lvlib\\stop curving"(w354, error in=w360) -> (error out=w357:errorcluster)
                n249 = local write "CURV?"(w354) -> ()
                n250 = Unbundle By Name(w357) -> ("status"=w356:bool)
                n251 = case shown="True" w356 {
                  tunnel: [Control_4."Waveform Queries" ("Enum") Control_4."Error Handler" ("Enum")] -> w355
                  tunnel: [w367 w370] -> w353
                  tunnel: w352 -> [w367 w369]
                  frame False {
                  }
                  frame True {
                    n252 = Flush Queue(queue=w369) -> (queue out=w370:refnum<queue>)  [unwired: 1 in, 2 out]
                  }
                }
              }
              frame "Delay" {
                w375 = FALSE ("stop curving")
                n253 = local read "Delay"() -> (w380:bool)
                n254 = local read "Delay Position"() -> (w381:u32)
                n255 = local read "Delay Time"() -> (w379:dbl)
                n256 = call <instrlib>:"Delay params..vi"("Delay Time"=w379, "Delay Position"=w381, "error in (no error)"=w371, "selector"=w380, "VISA resource name"=w372) -> ("error out"=w382:errorcluster, "VISA resource name out"=w383:refnum<visa-resource-name>)  [unwired: 5 in]
                n257 = shared-variable ".\\Shared Variables.lvlib\\stop curving"(w375, error in=w382) -> (error out=w378:errorcluster)
                n258 = local write "CURV?"(w375) -> ()
                n259 = Unbundle By Name(w378) -> ("status"=w377:bool)
                n260 = case shown="False" w377 {
                  tunnel: [Control_4."Waveform Queries" ("Enum") Control_4."Error Handler" ("Enum")] -> w376
                  tunnel: [w385 w388] -> w374
                  tunnel: w373 -> [w385 w387]
                  frame False {
                  }
                  frame True {
                    n261 = Flush Queue(queue=w387) -> (queue out=w388:refnum<queue>)  [unwired: 1 in, 2 out]
                  }
                }
              }
              frame "AUTOSET" {
                w391 = FALSE ("stop curving")
                n262 = local read "AUTOSET"() -> (w396:bool)
                n263 = case shown="True" w396 {
                  tunnel: w395 -> [w406 w410]
                  tunnel: w399 -> [w405 w409]
                  tunnel: [w405 w408] -> w398
                  tunnel: [w406 w407] -> w397
                  frame False {
                  }
                  frame True {
                    n264 = call <instrlib>:"Autosetup.vi"("error in (no error)"=w410, "VISA resource name"=w409) -> ("error out"=w407:errorcluster, "VISA resource name out"=w408:refnum<visa-resource-name>)  [unwired: 8 in]
                  }
                }
                n265 = shared-variable ".\\Shared Variables.lvlib\\stop curving"(w391, error in=w397) -> (error out=w394:errorcluster)
                n266 = local write "CURV?"(w391) -> ()
                n267 = Unbundle By Name(w394) -> ("status"=w393:bool)
                n268 = case shown="True" w393 {
                  tunnel: [Control_4."Waveform Queries" ("Enum") Control_4."Error Handler" ("Enum")] -> w392
                  tunnel: [w401 w404] -> w390
                  tunnel: w389 -> [w401 w403]
                  frame False {
                  }
                  frame True {
                    n269 = Flush Queue(queue=w403) -> (queue out=w404:refnum<queue>)  [unwired: 1 in, 2 out]
                  }
                }
              }
              frame "Trigger" {
                w413 = FALSE ("stop curving")
                n270 = local read "Source (0:Channel1)"() -> (w419:u16)
                n271 = local read "Trigger Event (0:A Event)"() -> (w421:u16)
                n272 = local read "Trigger Level (0.0)"() -> (w418:dbl)
                n273 = local read "Coupling (0:DC)"() -> (w420:u16)
                n274 = local read "Slope (0:Rise)"() -> (w417:u16)
                n275 = call-poly <instrlib>:"Configure Trigger.vi"("VISA resource name"=w425, "Coupling (0:DC)"=w420, "Trigger Event (0:A Event)"=w421, "Source (0:Channel1)"=w419, "Trigger Level (0.0V)"=w418, "Slope (0:Rise)"=w417, "error in (no error)"=w424) -> ("VISA resource name out"=w423:refnum<visa-resource-name>, "error out"=w422:errorcluster)  [unwired: 7 in]
                n276 = shared-variable ".\\Shared Variables.lvlib\\stop curving"(w413, error in=w422) -> (error out=w416:errorcluster)
                n277 = local write "CURV?"(w413) -> ()
                n278 = Unbundle By Name(w416) -> ("status"=w415:bool)
                n279 = case shown="False" w415 {
                  tunnel: [Control_4."Waveform Queries" ("Enum") Control_4."Error Handler" ("Enum")] -> w414
                  tunnel: [w427 w430] -> w412
                  tunnel: w411 -> [w427 w429]
                  frame False {
                  }
                  frame True {
                    n280 = Flush Queue(queue=w429) -> (queue out=w430:refnum<queue>)  [unwired: 1 in, 2 out]
                  }
                }
              }
              frame "Ver/Hor Queries" {
                w434 = FALSE ("stop curving")
                n281 = local read "Channel (0: Channel 1)"() -> (w438:u16)
                n282 = call <instrlib>:"Horizontal Queries.vi"("error in (no error)"=w448, "VISA resource name"=w449) -> ("error out"=w445:errorcluster, "Time/Div."=→"Time/Div.":dbl, "Acquisition Length"=→"Acquisition Length":dbl, "VISA resource name out"=w447:refnum<visa-resource-name>, "Sample Rate"=→"Sample Rate":dbl, "Acquisition Duration"=→"Acquisition Duration":dbl)  [unwired: 4 in]
                n283 = call <instrlib>:"Vertical Queries.vi"("error in (no error)"=w445, "Channel (0:Channel1)"=w438, "VISA resource name"=w447) -> ("error out"=w439:errorcluster, "VISA resource name out"=w446:refnum<visa-resource-name>, "Volt/Div."=→"Volt/Div.":dbl)  [unwired: 4 in, 2 out]
                n284 = shared-variable ".\\Shared Variables.lvlib\\stop curving"(w434, error in=w439) -> (error out=w437:errorcluster)
                n285 = local write "CURV?"(w434) -> ()
                n286 = Unbundle By Name(w437) -> ("status"=w436:bool)
                n287 = case shown="False" w436 {
                  tunnel: [Control_4."Waveform Queries" ("Enum") Control_4."Error Handler" ("Enum")] -> w435
                  tunnel: [w451 w454] -> w433
                  tunnel: w432 -> [w451 w453]
                  frame False {
                  }
                  frame True {
                    n288 = Flush Queue(queue=w453) -> (queue out=w454:refnum<queue>)  [unwired: 1 in, 2 out]
                  }
                }
                n289 = Wait (ms)(milliseconds to wait=u32 100) -> ()  [unwired: 1 out]
              }
              frame "Waveform Queries" {
                n290 = stacked-sequence {
                  tunnel: w461 -> [w497 _]
                  tunnel: w460 -> [w466 _]
                  tunnel: [w496 _] -> w456
                  tunnel: [w495 _] -> w458
                  frame #0 {
                    # "There should be a save case when in\n\"Uninterrupted\" mode."
                    n291 = while {
                      tunnel: w497 -> [w546]
                      tunnel: [w543] -> w496
                      tunnel: [w513] -> w464
                      shift-right: [w514] -> w465
                      shift-left: w466 -> [w545]
                      stop <- w535 stop-if-true
                      n292 = local read "Channel (0: Channel 1)"() -> (w515:u16)
                      n293 = call-poly <instrlib>:"Read.vi"("error in (no error)"=w545, "Maximum Time (10000 ms)"=u32 10000, "Channel (0: Channel 1)"=w515, "VISA resource name"=w546) -> ("error out"=w542:errorcluster, "Waveform Data"=w513:waveform(dbl), "VISA resource name out"=w544:refnum<visa-resource-name>)  [unwired: 5 in]
                      "Waveform Graph" <- w513
                      n294 = call <instrlib>:"Number of Acquisitions.vi"("error in (no error)"=w542, "VISA resource name"=w544) -> ("error out"=w539:errorcluster, "Number of Acquisitions"=→"Number of Acquisitions":u32, "VISA resource name out"=w541:refnum<visa-resource-name>)  [unwired: 7 in]
                      n295 = case shown="True" "Integrate" {
                        tunnel: w541 -> [w549 w559]
                        tunnel: [w549 w558] -> w540
                        tunnel: w539 -> [w548 w557]
                        tunnel: [w548 w553] -> w537
                        tunnel: w515 -> [_ w550]
                        frame False {
                        }
                        frame True {
                          n296 = call <instrlib>:"Gated Integration.vi"("error in (no error)"=w557, "Measurement Source"=w550, "VISA resource name"=w559) -> ("error out"=w554:errorcluster, "Unit"=→"Unit":string, "Area"=w555:dbl, "VISA resource name out"=w558:refnum<visa-resource-name>)  [unwired: 5 in]
                          "Area" <- w555
                          n297 = shared-variable ".\\Shared Variables.lvlib\\Area"(w555, error in=w554) -> (error out=w552:errorcluster)
                          n298 = Tick Count (ms)() -> (millisecond timer value=w551:u32)
                          n299 = shared-variable ".\\Shared Variables.lvlib\\osc tick"(w551, error in=w552) -> (error out=w553:errorcluster)
                        }
                      }
                      n300 = local read "Cursor ON/OFF"() -> (w520:bool)
                      n301 = local read "Record Length (10000)"() -> (w521:u32)
                      n302 = Wait (ms)(milliseconds to wait=u32 100) -> ()  [unwired: 1 out]
                      n303 = shared-variable ".\\Shared Variables.lvlib\\stop curving"() -> (w518:bool)  [unwired: 1 in, 1 out]
                      n304 = call <instrlib>:"Cursors.vi"("VISA resource name"=w540, "Snap"="Snap", "T Cursor"="T Cursor", "B Cursor"="B Cursor", "DATA:STOP"=w521, "error in (no error)"=w537, "L Cursor"="L Cursor 2", "R Cursor"="R Cursor 2", "Cursor Type"="Cursor Type", "ON/OFF"=w520) -> ("delta t"=→"delta t":dbl, "VISA resource name out"=w543:refnum<visa-resource-name>, "L Cursor"=w525:dbl, "T Cursor"=w524:dbl, "B Cursor"=w523:dbl, "delta V"=→"delta V":dbl, "R Cursor"=w522:dbl, "error out"=w514:errorcluster)  [unwired: 10 in]
                      "R Cursor" <- w522
                      "L Cursor" <- w525
                      "B Cursor" <- w523
                      "T Cursor" <- w524
                      n305 = shared-variable ".\\Shared Variables.lvlib\\L cursor"(w525) -> ()  [unwired: 1 in, 1 out]
                      n306 = shared-variable ".\\Shared Variables.lvlib\\T cursor"(w524) -> ()  [unwired: 1 in, 1 out]
                      n307 = shared-variable ".\\Shared Variables.lvlib\\B cursor"(w523) -> ()  [unwired: 1 in, 1 out]
                      n308 = local write "CURV?"("Save waveform") -> ()
                      n309 = Unbundle By Name(w514) -> ("status"=w536:bool)
                      n310 = Or(x="Save waveform", y=w518) -> (x .or. y?=w517:bool)
                      n311 = shared-variable ".\\Shared Variables.lvlib\\R cursor"(w522) -> ()  [unwired: 1 in, 1 out]
                      n312 = Or(x=w536, y=w517) -> (x .or. y?=w535:bool)
                    }
                    n313 = local read "Vertical Offset (0.0 V)"() -> (w480:dbl)
                    n314 = local read "Vertical Position"() -> (w481:dbl)
                    n315 = local read "Volt/Div."() -> (w479:dbl)
                    n316 = call <instrlib>:"Y Scale.vi"("Volt/Div."=w479, "Offset"=w480, "Position"=w481) -> ("Y Minor Inc"=w485:dbl, "Y Min"=w483:dbl, "Y Inc"=w484:dbl, "Y Max"=w482:dbl)  [unwired: 5 in]
                    n317 = property on="T Cursor" class="Slide (strict)"(error in=w466, "Increment"=w484, "Maximum"=w482, "Minimum"=w483) -> (error out=w478:errorcluster)  [unwired: 1 in, 1 out]
                    n318 = property on="B Cursor" class="Slide (strict)"(error in=w478, "Increment"=w484, "Maximum"=w482, "Minimum"=w483) -> (error out=w477:errorcluster)  [unwired: 1 in, 1 out]
                    n319 = property on="Waveform Graph" class="WFGraph (strict)"(error in=w477, "YScale.Increment"=w484, "YScale.Maximum"=w482, "YScale.Minimum"=w483, "YScale.MinorInc"=w485, "YScale.Visible"=TRUE ("Y Scale.Visible")) -> (error out=w476:errorcluster)  [unwired: 1 in, 1 out]
                    n320 = property on="T Cursor" class="Slide (strict)"(error in=w476, "Scale.Maximum"=w482, "Scale.Minimum"=w483, "Scale.MinorInc"=w485) -> (error out=w475:errorcluster)  [unwired: 1 in, 1 out]
                    n321 = property on="B Cursor" class="Slide (strict)"(error in=w475, "Scale.Maximum"=w482, "Scale.Minimum"=w483, "Scale.MinorInc"=w485) -> (error out=w467:errorcluster)  [unwired: 1 in, 1 out]
                    n322 = local read "Delay"() -> (w490:bool)
                    n323 = case shown="True" w490 {
                      tunnel: [w498 w499] -> w487
                      frame False {
                        n324 = local read "Position (0.0 s)"() -> (w498:dbl)
                      }
                      frame True {
                        n325 = local read "Delay Position"() -> (w500:u32)
                        n326 = To Double Precision Float(number=w500) -> (double precision float=w499:dbl)
                      }
                    }
                    n327 = local read "Save waveform"() -> (w494:bool)
                    n328 = local read "Time/Div."() -> (w488:dbl)
                    n329 = case shown="True" w494 {
                      tunnel: w464 -> [_ w504]
                      tunnel: w465 -> [w501 w503]
                      tunnel: [w501 w502] -> w495
                      frame False {
                      }
                      frame True {
                        n330 = stacked-sequence {
                          tunnel: w504 -> [w510 _]
                          tunnel: w503 -> [w508 _]
                          tunnel: [w507 _] -> w502
                          frame #0 {
                            n331 = shared-variable ".\\Shared Variables.lvlib\\stop curving"(FALSE ("stop curving")) -> ()  [unwired: 1 in, 1 out]
                            n332 = call <instrlib>:"TDMS.vi"("error in (no error)"=w508, "Waveform Data"=w510, "file path"="file path") -> ("error out"=w507:errorcluster, "Status"=→"Saved":bool)  [unwired: 7 in]
                          }
                          frame #1 {
                            n333 = flat-sequence {
                              frame #0 {
                                n334 = Wait (ms)(milliseconds to wait=u32 100) -> ()  [unwired: 1 out]
                              }
                              frame #1 {
                                n335 = local write "Saved"(FALSE ("Saved")) -> ()
                              }
                            }
                          }
                        }
                      }
                    }
                    n336 = call <instrlib>:"WF Graph Scale Calculator.vi"("Delay Position"=w487, "Time/Div."=w488) -> ("X Inc"=w492:dbl, "X Max"=w491:dbl, "X Min"=w493:dbl, "X Minor Inc"=w468:dbl)  [unwired: 6 in]
                    n337 = property on="R Cursor 2" class="Slide (strict)"(error in=w467, "Scale.Maximum"=w491, "Scale.Minimum"=w493, "Scale.MinorInc"=w468) -> (error out=w474:errorcluster)  [unwired: 1 in, 1 out]
                    n338 = property on="Waveform Graph" class="WFGraph (strict)"(error in=w474, "XScale.Increment"=w492, "XScale.Maximum"=w491, "XScale.Minimum"=w493, "XScale.MinorInc"=w468, "XScale.Visible"=TRUE ("X Scale.Visible"), "XScale.Offset"=w493) -> (error out=w473:errorcluster)  [unwired: 1 in, 1 out]
                    n339 = property on="L Cursor 2" class="Slide (strict)"(error in=w473, "Increment"=w468, "Maximum"=w491, "Minimum"=w493) -> (error out=w472:errorcluster)  [unwired: 1 in, 1 out]
                    n340 = property on="L Cursor 2" class="Slide (strict)"(error in=w472, "Scale.Maximum"=w491, "Scale.Minimum"=w493, "Scale.MinorInc"=w468) -> (error out=w471:errorcluster)  [unwired: 1 in, 1 out]
                    n341 = property on="R Cursor 2" class="Slide (strict)"(error in=w471, "Increment"=w468, "Maximum"=w491, "Minimum"=w493) -> (error out=w470:errorcluster)  [unwired: 1 in, 1 out]
                    "Cursors" <- w470
                    n342 = Unbundle By Name(w470) -> ("status"=→"Cursors Error Status":bool)
                  }
                  frame #1 {
                    w560 = FALSE ("Stop Curving")
                    n343 = shared-variable ".\\Shared Variables.lvlib\\stop curving"(w560) -> ()  [unwired: 1 in, 1 out]
                    n344 = local write "CURV?"(w560) -> ()
                  }
                }
                n345 = Unbundle By Name(w458) -> ("status"=w459:bool)
                n346 = case shown="False" w459 {
                  tunnel: [Control_4."Waveform Queries" ("Enum") Control_4."Error Handler" ("Enum")] -> w457
                  frame False {
                  }
                  frame True {
                  }
                }
              }
              frame "Stop " {
                n347 = call <instrlib>:"Close.vi"("error in (no error)"=w568, "VISA resource name"=w566) -> ("error out"=w567:errorcluster)  [unwired: 9 in]
                n348 = call <vilib>:"Simple Error Handler.vi"("error in (no error)"=w567) -> ("error out"=w562:errorcluster)  [unwired: 4 in, 4 out]
                n349 = Unbundle By Name(w562) -> ("status"=w561:bool)
                n350 = case shown="True" w561 {
                  tunnel: [Control_4."Idle" ("Enum") Control_4."Error Handler" ("Enum")] -> w565
                  tunnel: [w571 w574] -> w564
                  tunnel: w563 -> [w570 w573]
                  frame False {
                    n351 = Flush Queue(queue=w570) -> (queue out=w571:refnum<queue>)  [unwired: 1 in, 2 out]
                  }
                  frame True {
                    n352 = Flush Queue(queue=w573) -> (queue out=w574:refnum<queue>)  [unwired: 1 in, 2 out]
                  }
                }
              }
              frame "Error Handler" {
                n353 = call <vilib>:"Simple Error Handler.vi"("error in (no error)"=w581) -> ("code out"=→"code out":i32, "source out"=→"source out":string, "error out"=w578:errorcluster)  [unwired: 4 in, 2 out]
                n354 = Flush Queue(queue=w576) -> (queue out=w577:refnum<queue>)  [unwired: 1 in, 2 out]
              }
            }
            n355 = shared-variable ".\\Shared Variables.lvlib\\Shutdown"() -> (w200:bool)  [unwired: 1 in, 1 out]
            n356 = Enqueue Element(queue=w204, element=w210, error in (no error)=w209) -> (queue out=w211:refnum<queue>, error out=w203:errorcluster)  [unwired: 1 in, 1 out]
            n357 = call <vilib>:"Simple Error Handler.vi"("error in (no error)"=w203) -> ()  [unwired: 4 in, 5 out]
            n358 = Wait (ms)(milliseconds to wait=u32 10) -> ()  [unwired: 1 out]
          }
          n359 = while {
            stop <- w160 stop-if-true
            n360 = Wait (ms)(milliseconds to wait=u32 1) -> ()  [unwired: 1 out]
            n361 = case shown="True" "Cursor ON/OFF" {
              frame False {
              }
              frame True {
                n362 = local read "Cursor Type"() -> (w163:enum16{"Vertical", "Horizontal", "Screen"})
                n363 = case shown="\"Vertical\"" w163 {
                  frame "Vertical" {
                    n364 = shared-variable ".\\Shared Variables.lvlib\\L cursor"() -> (w164:dbl)  [unwired: 1 in, 1 out]
                    n365 = shared-variable ".\\Shared Variables.lvlib\\R cursor"() -> (w165:dbl)  [unwired: 1 in, 1 out]
                    n366 = Bundle By Name(cluster=T4 {"Name"="Cursor 0", "Color"=16776960, "Style"=2, "Point Style"=0, "Name Visible"=FALSE, "Allow Drag"=TRUE, "Cursor Mode"=0, "Plot"=0, "Index"=0, "Position"={"X"=0.0, "Y"=-inf}, "X Scale"=0, "Y Scale"=0, "Watch Plots"=[], "Watch All Plots"=FALSE, "Plot Area"=0, "Label Offset"={"X"=0.0, "Y"=0.0}} ("Cluster"), "Position.X"=w164, "Point Style"="Vertical Cursor Style") -> (w170:T4)
                    n367 = Bundle By Name(cluster=T4 {"Name"="Cursor 0", "Color"=16776960, "Style"=2, "Point Style"=0, "Name Visible"=FALSE, "Allow Drag"=TRUE, "Cursor Mode"=0, "Plot"=0, "Index"=0, "Position"={"X"=0.0, "Y"=-inf}, "X Scale"=0, "Y Scale"=0, "Watch Plots"=[], "Watch All Plots"=FALSE, "Plot Area"=0, "Label Offset"={"X"=0.0, "Y"=0.0}} ("Cluster"), "Position.X"=w165, "Point Style"="Vertical Cursor Style") -> (w168:T4)
                    n368 = Build Array(w170) -> (w169:T7)
                    n369 = Build Array(w168) -> (w167:T7)
                    n370 = property on="Waveform Graph" class="WFGraph (strict)"("CrsrList"=w169) -> ()  [unwired: 2 in, 2 out]
                    n371 = property on="Waveform Graph" class="WFGraph (strict)"("CrsrList"=w167) -> ()  [unwired: 2 in, 2 out]
                  }
                  frame "Horizontal" {
                    n372 = shared-variable ".\\Shared Variables.lvlib\\T cursor"() -> (w174:dbl)  [unwired: 1 in, 1 out]
                    n373 = shared-variable ".\\Shared Variables.lvlib\\B cursor"() -> (w173:dbl)  [unwired: 1 in, 1 out]
                    n374 = Bundle By Name(cluster=T4 {"Name"="Cursor 0", "Color"=16776960, "Style"=2, "Point Style"=0, "Name Visible"=FALSE, "Allow Drag"=TRUE, "Cursor Mode"=0, "Plot"=0, "Index"=0, "Position"={"X"=0.0, "Y"=-inf}, "X Scale"=0, "Y Scale"=0, "Watch Plots"=[], "Watch All Plots"=FALSE, "Plot Area"=0, "Label Offset"={"X"=0.0, "Y"=0.0}} ("Cluster"), "Position.Y"=w174, "Style"="Horizontal Cursor Style") -> (w178:T4)
                    n375 = Bundle By Name(cluster=T4 {"Name"="Cursor 0", "Color"=16776960, "Style"=2, "Point Style"=0, "Name Visible"=FALSE, "Allow Drag"=TRUE, "Cursor Mode"=0, "Plot"=0, "Index"=0, "Position"={"X"=0.0, "Y"=-inf}, "X Scale"=0, "Y Scale"=0, "Watch Plots"=[], "Watch All Plots"=FALSE, "Plot Area"=0, "Label Offset"={"X"=0.0, "Y"=0.0}} ("Cluster"), "Position.Y"=w173, "Style"="Horizontal Cursor Style") -> (w180:T4)
                    n376 = Build Array(w178) -> (w177:T7)
                    n377 = Build Array(w180) -> (w179:T7)
                    n378 = property on="Waveform Graph" class="WFGraph (strict)"("CrsrList"=w177) -> ()  [unwired: 2 in, 2 out]
                    n379 = property on="Waveform Graph" class="WFGraph (strict)"("CrsrList"=w179) -> ()  [unwired: 2 in, 2 out]
                  }
                  frame "Screen" {
                    n380 = local read "Horizontal Cursor Style"() -> (w195:i32)
                    n381 = local read "Vertical Cursor Style"() -> (w194:i32)
                    n382 = shared-variable ".\\Shared Variables.lvlib\\B cursor"() -> (w182:dbl)  [unwired: 1 in, 1 out]
                    n383 = shared-variable ".\\Shared Variables.lvlib\\T cursor"() -> (w183:dbl)  [unwired: 1 in, 1 out]
                    n384 = shared-variable ".\\Shared Variables.lvlib\\L cursor"() -> (w185:dbl)  [unwired: 1 in, 1 out]
                    n385 = shared-variable ".\\Shared Variables.lvlib\\R cursor"() -> (w184:dbl)  [unwired: 1 in, 1 out]
                    n386 = Bundle By Name(cluster=T4 {"Name"="Cursor 0", "Color"=16776960, "Style"=2, "Point Style"=0, "Name Visible"=FALSE, "Allow Drag"=TRUE, "Cursor Mode"=0, "Plot"=0, "Index"=0, "Position"={"X"=0.0, "Y"=-inf}, "X Scale"=0, "Y Scale"=0, "Watch Plots"=[], "Watch All Plots"=FALSE, "Plot Area"=0, "Label Offset"={"X"=0.0, "Y"=0.0}} ("Cluster"), "Position.Y"=w183, "Style"=w195) -> (w189:T4)
                    n387 = Bundle By Name(cluster=T4 {"Name"="Cursor 0", "Color"=16776960, "Style"=2, "Point Style"=0, "Name Visible"=FALSE, "Allow Drag"=TRUE, "Cursor Mode"=0, "Plot"=0, "Index"=0, "Position"={"X"=0.0, "Y"=-inf}, "X Scale"=0, "Y Scale"=0, "Watch Plots"=[], "Watch All Plots"=FALSE, "Plot Area"=0, "Label Offset"={"X"=0.0, "Y"=0.0}} ("Cluster"), "Position.Y"=w182, "Style"=w195) -> (w187:T4)
                    n388 = Bundle By Name(cluster=T4 {"Name"="Cursor 0", "Color"=16776960, "Style"=2, "Point Style"=0, "Name Visible"=FALSE, "Allow Drag"=TRUE, "Cursor Mode"=0, "Plot"=0, "Index"=0, "Position"={"X"=0.0, "Y"=-inf}, "X Scale"=0, "Y Scale"=0, "Watch Plots"=[], "Watch All Plots"=FALSE, "Plot Area"=0, "Label Offset"={"X"=0.0, "Y"=0.0}} ("Cluster"), "Position.X"=w185, "Point Style"=w194) -> (w193:T4)
                    n389 = Bundle By Name(cluster=T4 {"Name"="Cursor 0", "Color"=16776960, "Style"=2, "Point Style"=0, "Name Visible"=FALSE, "Allow Drag"=TRUE, "Cursor Mode"=0, "Plot"=0, "Index"=0, "Position"={"X"=0.0, "Y"=-inf}, "X Scale"=0, "Y Scale"=0, "Watch Plots"=[], "Watch All Plots"=FALSE, "Plot Area"=0, "Label Offset"={"X"=0.0, "Y"=0.0}} ("Cluster"), "Position.X"=w184, "Point Style"=w194) -> (w191:T4)
                    n390 = Build Array(w189) -> (w188:T7)
                    n391 = Build Array(w187) -> (w186:T7)
                    n392 = Build Array(w193) -> (w192:T7)
                    n393 = Build Array(w191) -> (w190:T7)
                    n394 = property on="Waveform Graph" class="WFGraph (strict)"("CrsrList"=w188) -> ()  [unwired: 2 in, 2 out]
                    n395 = property on="Waveform Graph" class="WFGraph (strict)"("CrsrList"=w186) -> ()  [unwired: 2 in, 2 out]
                    n396 = property on="Waveform Graph" class="WFGraph (strict)"("CrsrList"=w192) -> ()  [unwired: 2 in, 2 out]
                    n397 = property on="Waveform Graph" class="WFGraph (strict)"("CrsrList"=w190) -> ()  [unwired: 2 in, 2 out]
                  }
                }
              }
            }
            n398 = shared-variable ".\\Shared Variables.lvlib\\Shutdown"() -> (w160:bool)  [unwired: 1 in, 1 out]
          }
          n399 = Release Queue(queue=w159, error in (no error)=w155) -> (error out=w158:errorcluster)  [unwired: 1 in, 2 out]
          n400 = call <vilib>:"Simple Error Handler.vi"("error in (no error)"=w158) -> ("error out"=→"Main":errorcluster)  [unwired: 4 in, 4 out]
        }
        frame True {
          n401 = local read "Handle"() -> (w583:i32)
          n402 = while {
            tunnel: w590 -> [w605]
            shift-right: [w600] -> _
            shift-left: w589 -> [w601]
            shift-right: [w599] -> w587
            shift-left: w591 -> [w603]
            shift-right: [w596] -> w586
            shift-left: w588 -> [w598]
            shift-right: [w594] -> _
            shift-left: w583 -> [w593]
            stop <- w595 stop-if-true
            n403 = Dequeue Element(queue=w603, error in (no error)=w605) -> (element=w604:T3)  [unwired: 1 in, 3 out]
            "status" <- w604
            n404 = case shown="\"Error Handler\"" w604 {
              tunnel: [w606 Control_4."Idle" ("Enum") w633 w682 w733 w771 w847 w1047 w1065] -> w602
              tunnel: w598 -> [w608 w632 w642 w695 w730 w772 w850 w1052 w1069]
              tunnel: w601 -> [w610 w627 w641 w692 w718 w752 w851 w1048 w1063]
              tunnel: [w610 w627 w641 w691 w717 w753 w835 w1048 w1063] -> w600
              tunnel: [w608 w629 w637 w654 w734 w756 w845 w1044 w1064] -> w597
              tunnel: [w609 w626 w640 w657 w731 w754 w836 _ w1061] -> w594
              tunnel: w593 -> [w609 w626 w639 w658 w732 w758 w837 w1046 w1062]
              frame "Idle", Default {
                n405 = shared-variable ".\\Shared Variables.lvlib\\Gate Open"() -> (w607:bool)  [unwired: 1 in, 1 out]
                n406 = case shown="False" w607 {
                  tunnel: [w611 Control_4."C8855-Count Start" ("Enum")] -> w606
                  frame False {
                    n407 = shared-variable ".\\Shared Variables.lvlib\\iHR550_GL302_scan"() -> (w612:bool)  [unwired: 1 in, 1 out]
                    n408 = case shown="True" w612 {
                      tunnel: [w615 w620] -> w611
                      frame False {
                        n409 = local write "iterations"(0 ("iterations")) -> ()
                        n410 = local read "Measure"() -> (w614:bool)
                        n411 = case shown="True" w614 {
                          tunnel: [Control_4."Idle" ("Enum") Control_4."C8855-Count Start" ("Enum")] -> w615
                          frame False {
                          }
                          frame True {
                          }
                        }
                      }
                      frame True {
                        n412 = shared-variable ".\\Shared Variables.lvlib\\C8855-Avg"() -> (w619:bool)  [unwired: 1 in, 1 out]
                        n413 = local write "iterations"(0 ("iterations")) -> ()
                        n414 = case shown="False" w619 {
                          tunnel: [Control_4."Idle" ("Enum") Control_4."C8855-Count Start" ("Enum")] -> w620
                          frame False {
                            w621 = FALSE ("iHR550_scan")
                            n415 = Tick Count (ms)() -> (millisecond timer value=w623:u32)
                            n416 = shared-variable ".\\Shared Variables.lvlib\\osc tick"(w623) -> ()  [unwired: 1 in, 1 out]
                            n417 = shared-variable ".\\Shared Variables.lvlib\\iHR550_GL302_scan"(w621) -> ()  [unwired: 1 in, 1 out]
                            n418 = local write "Measure"(w621) -> ()
                          }
                          frame True {
                          }
                        }
                      }
                    }
                  }
                  frame True {
                  }
                }
              }
              frame "Error Handler" {
                n419 = call <vilib>:"Simple Error Handler.vi"("error in (no error)"=w632) -> ("code out"=→"code out 2":i32, "source out"=→"source out 3":string, "error out"=w629:errorcluster)  [unwired: 4 in, 2 out]
              }
              frame "C8855-Reset" {
                n420 = dll-call lib="C:/Users/physrin/Documents/LSLV/Labview Laser Spectroscopy/C8855-01api.dll" fn="_C8855Reset@4"(error in=w642, "Handle"=w639) -> (error out=w638:errorcluster, "Error"=w643:i32, "Handle"=w640:i32)  [unwired: 2 in, 1 out]
                n421 = call <vilib>:"Simple Error Handler.vi"("error in (no error)"=w638) -> ("code out"=w635:i32, "source out"=w636:string, "error out"=w637:errorcluster)  [unwired: 4 in, 2 out]
                n422 = Equal?(x=w643, y=-1) -> (x = y?=w634:bool)
                n423 = local write "source out 3"(w636) -> ()
                n424 = local write "code out 2"(w635) -> ()
                n425 = case shown="True" w634 {
                  tunnel: [Control_4."C8855-Measurement Setup" ("Enum") w646] -> w633
                  frame False {
                  }
                  frame True {
                    n426 = Two Button Dialog(message="C8855Reset()\nCheck C8855.", 1:"Continue" ("F button name (\"Cancel\")"), 2:"Shutdown" ("T button name (\"OK\")")) -> (T button?=w647:bool)
                    n427 = case shown="False" w647 {
                      tunnel: [Control_4."C8855-Reset" ("Enum") Control_4."C8855-Close" ("Enum")] -> w646
                      frame False {
                      }
                      frame True {
                        n428 = Quit LabVIEW(quit? (T)=TRUE) -> ()
                      }
                    }
                  }
                }
              }
              frame "C8855-Measurement Setup" {
                # "C8855 gate time array"
                n429 = Build Array(5e-05, 0.0001, 0.0002, 0.0005, 0.001, 0.002, 0.005, 0.01, 0.02, 0.05, 0.1, 0.2, 0.5, 1.0, 2.0, 5.0, 10.0) -> (w664:dbl[])
                n430 = Unbundle By Name(w692) -> ("C8855 Measurement Parameters"=w694:T8)
                n431 = local read "Measurement points"() -> (w662:u32)
                n432 = local read "C8855 gate time"() -> (w663:i32)
                n433 = Index Array(array=w664, index=w663) -> (element=w655:dbl)
                "time step" <- w655
                n434 = call "c8855_calc_measurement_params_sub.vi"("measurement params"=w694, "Gate time"=w663, "Measurement points"=w662) -> ("measurement params out"=w693:T9)  [unwired: 2 in]
                n435 = To Double Precision Float(number=w662) -> (double precision float=w661:dbl)
                n436 = Multiply(x=w655, y=w661) -> (x*y=→"Measurement Time (sec)":dbl)
                n437 = Unbundle By Name(w693) -> ("Gate time"=w659:u8, "Number of gates"=w689:u16)
                n438 = dll-call lib="C:/Users/physrin/Documents/LSLV/Labview Laser Spectroscopy/C8855-01api.dll" fn="_C8855Setup@16"(error in=w695, "Handle"=w658, "Gatetime"=w659, "Transmode"=u8 2 ("TransferMode"), "Number of gate"=w689) -> (error out=w656:errorcluster, "Error"=w685:i32, "Handle"=w657:i32)  [unwired: 5 in, 1 out]
                n439 = To Long Integer(number=w689) -> (32bit integer=w688:i32)
                n440 = Initialize Array(u32 0 ("element"), w688) -> (w686:u32[])
                n441 = Bundle By Name(cluster=w692, "C8855 Measurement Parameters"=w693, "Data Buffer"=w686) -> (w691:T6)
                n442 = Equal?(x=w685, y=-1) -> (x = y?=w683:bool)
                n443 = case shown="False" w683 {
                  tunnel: [Control_4."Idle" ("Enum") w709] -> w682
                  tunnel: w656 -> [w697 w708]
                  tunnel: [w696 w708] -> w654
                  frame False {
                    n444 = local read "Scan GL302"() -> (w698:bool)
                    n445 = local read "Scan"() -> (w699:bool)
                    n446 = Exclusive Or(1:w698, 2:w699) -> (0:w700:bool)
                    n447 = case shown="True" w700 {
                      tunnel: w697 -> [w703 w706]
                      tunnel: [w702 w705] -> w696
                      frame False {
                        n448 = shared-variable ".\\Shared Variables.lvlib\\iHR550_GL302_scan"(FALSE ("iHR550_GL302_scan"), error in=w703) -> (error out=w702:errorcluster)
                      }
                      frame True {
                        n449 = shared-variable ".\\Shared Variables.lvlib\\iHR550_GL302_scan"(TRUE ("iHR550_GL302_scan"), error in=w706) -> (error out=w705:errorcluster)
                      }
                    }
                  }
                  frame True {
                    n450 = Two Button Dialog(message="C8855Setup()\nCheck C8855.", 1:"Continue" ("F button name (\"Cancel\")"), 2:"Shutdown" ("T button name (\"OK\")")) -> (T button?=w710:bool)
                    n451 = case shown="False" w710 {
                      tunnel: [Control_4."C8855-Reset" ("Enum") Control_4."C8855-Close" ("Enum")] -> w709
                      frame False {
                      }
                      frame True {
                        n452 = Quit LabVIEW(quit? (T)=TRUE) -> ()
                      }
                    }
                  }
                }
              }
              frame "C8855-Count Start" {
                n453 = Unbundle By Name(w718) -> ("C8855 Measurement Parameters.Number of Gates"=w721:u16)
                n454 = To Long Integer(number=w721) -> (32bit integer=w720:i32)
                n455 = Initialize Array(u32 0 ("element"), w720) -> (w719:u32[])
                n456 = Bundle By Name(cluster=w718, "Data Buffer"=w719) -> (w717:T6)
                n457 = case shown="\"External\", Default" "Triggers" {
                  tunnel: [u8 0 u8 1] -> w728
                  frame "Software" {
                  }
                  frame "External", Default {
                  }
                }
                n458 = dll-call lib="C:/Users/physrin/Documents/LSLV/Labview Laser Spectroscopy/C8855-01api.dll" fn="_C8855CountStart@8"(error in=w730, "Handle"=w732, "TriggerMode"=w728) -> (error out=w723:errorcluster, "Error"=w727:i32, "Handle"=w731:i32)  [unwired: 3 in, 1 out]
                n459 = Equal?(x=w727, y=0) -> (x = y?=w725:bool)
                n460 = case shown="False" w725 {
                  tunnel: [Control_4."C8855-Data Update" ("Enum") w736] -> w733
                  frame False {
                  }
                  frame True {
                    n461 = Two Button Dialog(message="C8855CountStart()\nCheck C8855.", 1:"Continue" ("F button name (\"Cancel\")"), 2:"Shutdown" ("T button name (\"OK\")")) -> (T button?=w737:bool)
                    n462 = case shown="False" w737 {
                      tunnel: [Control_4."C8855-Reset" ("Enum") Control_4."C8855-Close" ("Enum")] -> w736
                      frame False {
                      }
                      frame True {
                        n463 = Quit LabVIEW(quit? (T)=TRUE) -> ()
                      }
                    }
                  }
                }
                n464 = shared-variable ".\\Shared Variables.lvlib\\Gate Open"(FALSE ("Gate Open"), error in=w723) -> (error out=w734:errorcluster)
              }
              frame "C8855-Monitor" {
                n465 = dll-call lib="C:/Users/physrin/Documents/LSLV/Labview Laser Spectroscopy/C8855-01api.dll" fn="_C8855Reset@4"(error in=w772, "Handle"=w758) -> (error out=w750:errorcluster, "Error"=w770:i32, "Handle"=w749:i32)  [unwired: 2 in, 1 out]
                n466 = dll-call lib="C:/Users/physrin/Documents/LSLV/Labview Laser Spectroscopy/C8855-01api.dll" fn="_C8855Setup@16"(error in=w750, "Handle"=w749, "Gatetime"=u8 12, "Transmode"=u8 2 ("TransferMode"), "Number of gate"=u16 10 ("NumberOfGate")) -> (error out=w763:errorcluster, "Error"=w769:i32, "Handle"=w762:i32)  [unwired: 5 in, 1 out]
                n467 = dll-call lib="C:/Users/physrin/Documents/LSLV/Labview Laser Spectroscopy/C8855-01api.dll" fn="_C8855CountStart@8"(error in=w763, "Handle"=w762, "TriggerMode"=u8 0) -> (error out=w757:errorcluster, "Error"=w760:i32, "Handle"=w755:i32)  [unwired: 3 in, 1 out]
                n468 = Equal?(x=w760, y=0) -> (x = y?=w759:bool)
                n469 = Equal?(x=w769, y=-1) -> (x = y?=w765:bool)
                n470 = Equal?(x=w770, y=-1) -> (x = y?=w766:bool)
                n471 = Compound Arithmetic op=OR(w759, w765, w766) -> (w764:bool)
                n472 = case shown="False" w764 {
                  tunnel: [w773 w821] -> w771
                  tunnel: w757 -> [w779 w820]
                  tunnel: [w775 w820] -> w756
                  tunnel: w755 -> [w778 w819]
                  tunnel: [w777 w819] -> w754
                  tunnel: w752 -> [w776 w818]
                  tunnel: [w774 w818] -> w753
                  frame False {
                    n473 = stacked-sequence {
                      seq-local: [_ w787 _] -> [_ _ _]
                      seq-local: [w782 _ _] -> [_ w785 _]
                      tunnel: w779 -> [_ w789 w806]
                      tunnel: w778 -> [_ w788 w808]
                      tunnel: [_ _ w807] -> w777
                      tunnel: w776 -> [w781 _ _]
                      tunnel: [_ _ w805] -> w775
                      tunnel: [_ w786 _] -> w774
                      tunnel: [_ _ w801] -> w773
                      frame #0 {
                        n474 = Initialize Array(u32 0 ("element"), 10 ("dimension size")) -> (w784:u32[])
                        n475 = Bundle By Name(cluster=w781, "Data Buffer"=w784) -> (w782:T6)
                      }
                      frame #1 {
                        n476 = while {
                          tunnel: w789 -> [w800]
                          tunnel: w785 -> [w799]
                          tunnel: w788 -> [w798]
                          tunnel: [w797] -> w787
                          tunnel: [w792] -> w786
                          stop <- w793 continue-if-true
                          n477 = call "C8855_read_data.vi"("error in (no error)"=w800, "Cluster in"=w799, "Handle"=w798) -> ("error out"=w797:errorcluster, "Data update error 1"=w796:bool, "Cluster out"=w792:T6)  [unwired: 2 in, 2 out]
                          n478 = local read "Monitor"() -> (w794:bool)
                          n479 = Not(x=w796) -> (.not. x?=w795:bool)
                          n480 = Unbundle By Name(w792) -> ("Data Buffer"=w791:u32[])
                          n481 = And(x=w795, y=w794) -> (x .and. y?=w793:bool)
                          n482 = Add Array Elements(numeric array=w791) -> (sum=w790:u32)
                          n483 = local write "Counts"(w790) -> ()
                        }
                      }
                      frame #2 {
                        n484 = dll-call lib="C:/Users/physrin/Documents/LSLV/Labview Laser Spectroscopy/C8855-01api.dll" fn="_C8855CountStop@4"(error in=w806, "Handle"=w808) -> (error out=w805:errorcluster, "Error"=w804:i32, "Handle"=w807:i32)  [unwired: 2 in, 1 out]
                        n485 = Equal?(x=w804, y=0) -> (x = y?=w802:bool)
                        n486 = case shown="False" w802 {
                          tunnel: [Control_4."C8855-Reset" ("Enum") w810] -> w801
                          frame False {
                          }
                          frame True {
                            n487 = Two Button Dialog(message="C8855CountStart()\nCheck C8855.", 1:"Continue" ("F button name (\"Cancel\")"), 2:"Shutdown" ("T button name (\"OK\")")) -> (T button?=w811:bool)
                            n488 = case shown="False" w811 {
                              tunnel: [Control_4."C8855-Reset" ("Enum") Control_4."C8855-Close" ("Enum")] -> w810
                              frame False {
                              }
                              frame True {
                                n489 = Quit LabVIEW(quit? (T)=TRUE) -> ()
                              }
                            }
                          }
                        }
                      }
                    }
                  }
                  frame True {
                    n490 = Two Button Dialog(message="C8855CountStart()\nCheck C8855.", 1:"Continue" ("F button name (\"Cancel\")"), 2:"Shutdown" ("T button name (\"OK\")")) -> (T button?=w822:bool)
                    n491 = case shown="False" w822 {
                      tunnel: [Control_4."C8855-Reset" ("Enum") Control_4."C8855-Close" ("Enum")] -> w821
                      frame False {
                      }
                      frame True {
                        n492 = Quit LabVIEW(quit? (T)=TRUE) -> ()
                      }
                    }
                  }
                }
              }
              frame "C8855-Data Update" {
                n493 = Unbundle By Name(w851) -> ("C8855 Measurement Parameters.For AVG"=w839:dbl[][], "C8855 Measurement Parameters.Number of measurements"=w855:i32, "C8855 Measurement Parameters.Number of blocks"=w854:i32)
                n494 = Equal?(x=w854, y=1) -> (x = y?=w852:bool)
                n495 = local read "Average"() -> (w840:bool)
                n496 = case shown="True" w840 {
                  tunnel: [1 w860] -> w841
                  frame False {
                    n497 = shared-variable ".\\Shared Variables.lvlib\\C8855-Avg"(FALSE ("C8855-Avg")) -> ()  [unwired: 1 in, 1 out]
                  }
                  frame True {
                    n498 = local read "Number of Averages"() -> (w861:u32)
                    n499 = shared-variable ".\\Shared Variables.lvlib\\C8855-Avg"(FALSE ("C8855-Avg")) -> ()  [unwired: 1 in, 1 out]
                    n500 = To Long Integer(number=w861) -> (32bit integer=w860:i32)
                  }
                }
                n501 = case shown="False" w852 {
                  tunnel: w837 -> [w865 w918]
                  tunnel: w850 -> [w872 w917]
                  tunnel: [w873 w916] -> w848
                  tunnel: [w874 w912] -> w846
                  tunnel: w851 -> [w871 w915]
                  tunnel: [w870 w914] -> w835
                  tunnel: w855 -> [w869 w913]
                  tunnel: [w866 w910] -> w838
                  tunnel: w854 -> [w868 _]
                  tunnel: w841 -> [_ w911]
                  tunnel: w839 -> [_ w908]
                  tunnel: [w865 w909] -> w836
                  frame False {
                    n502 = for {
                      N: w869 -> [_]
                      tunnel: [w886] -> w874
                      shift-right: [w885] -> w873
                      shift-left: w872 -> [w884]
                      shift-right: [w882] -> w870
                      shift-left: w871 -> [w883]
                      tunnel: w865 -> [w881]
                      tunnel: w868 -> [w879]
                      shift-right: [w875] -> w866
                      shift-left: u32[] [] -> [w877]
                      n503 = for {
                        N: w879 -> [_]
                        shift-right: [w897] -> w886
                        shift-left: FALSE -> [w893]
                        shift-right: [w896] -> w885
                        shift-left: w884 -> [w895]
                        shift-right: [w891] -> w882
                        shift-left: w883 -> [w894]
                        tunnel: w881 -> [w892]
                        shift-right: [w888] -> w878
                        shift-left: u32[] [] -> [w890]
                        n504 = case shown="False" w893 {
                          selector: w893 -> [_ w907]
                          tunnel: [w898 w907] -> w897
                          tunnel: [w904 w905] -> w896
                          tunnel: w895 -> [w903 w905]
                          tunnel: w894 -> [w902 w906]
                          tunnel: [w901 w906] -> w891
                          tunnel: w892 -> [w900 _]
                          frame False {
                            n505 = call "C8855_read_data.vi"("error in (no error)"=w903, "Cluster in"=w902, "Handle"=w900) -> ("error out"=w904:errorcluster, "Data update error 1"=w898:bool, "Result Returned"=→"Result Returned":u8, "Cluster out"=w901:T6)  [unwired: 2 in, 1 out]
                          }
                          frame True {
                          }
                        }
                        n506 = Unbundle By Name(w891) -> ("Data Buffer"=w889:u32[])
                        n507 = Build Array (concatenate)(w890, w889) -> (w888:u32[])
                      }
                      n508 = Add Array Elements(numeric array=w878) -> (sum=w876:u32)
                      n509 = Build Array (concatenate)(w877, w876) -> (w875:u32[])
                    }
                  }
                  frame True {
                    n510 = for {
                      N: w911 -> [_]
                      tunnel: w918 -> [w931]
                      tunnel: w913 -> [w927]
                      tunnel: [w926] -> w912
                      shift-right: [w929] -> w916
                      shift-left: w917 -> [w930]
                      shift-right: [w921] -> w914
                      shift-left: w915 -> [w928]
                      tunnel: w911 -> [w925]
                      tunnel: [w923] -> w910
                      tunnel: [w922] -> w909
                      shift-right: [w920] -> _
                      shift-left: w908 -> [w924]
                      i -> [w919]
                      n511 = stacked-sequence {
                        seq-local: [w934 _] -> [_ w972]
                        seq-local: [w933 _] -> [_ w967]
                        seq-local: [w932 _] -> [_ w964]
                        tunnel: w931 -> [w941 w962]
                        tunnel: w930 -> [w940 _]
                        tunnel: [_ w965] -> w929
                        tunnel: w928 -> [w939 _]
                        tunnel: w927 -> [w938 _]
                        tunnel: [w937 _] -> w926
                        tunnel: w925 -> [_ w973]
                        tunnel: w924 -> [_ w971]
                        tunnel: [_ w970] -> w920
                        tunnel: [_ w969] -> w923
                        tunnel: [_ w966] -> w922
                        tunnel: [_ w963] -> w921
                        frame #0 {
                          n512 = for {
                            N: w938 -> [_]
                            tunnel: w941 -> [w951]
                            shift-right: [w949] -> w933
                            shift-left: w940 -> [w950]
                            shift-right: [w942] -> w932
                            shift-left: w939 -> [w948]
                            shift-right: [w943] -> w934
                            shift-left: u32[] [] -> [w946]
                            shift-right: [w945] -> w937
                            shift-left: FALSE -> [w944]
                            n513 = case shown="False" w944 {
                              selector: w944 -> [_ w961]
                              tunnel: w951 -> [w958 _]
                              tunnel: w950 -> [w957 w959]
                              tunnel: [w956 w959] -> w949
                              tunnel: w948 -> [w955 w960]
                              tunnel: [w954 w960] -> w942
                              tunnel: [w953 w961] -> w945
                              frame False {
                                n514 = call "C8855_read_data.vi"("error in (no error)"=w957, "Cluster in"=w955, "Handle"=w958) -> ("error out"=w956:errorcluster, "Data update error 1"=w953:bool, "Result Returned"=w952:u8, "Cluster out"=w954:T6)  [unwired: 2 in, 1 out]
                                n515 = local write "Result Returned"(w952) -> ()
                              }
                              frame True {
                              }
                            }
                            n516 = Unbundle By Name(w942) -> ("Data Buffer"=w947:u32[])
                            n517 = Build Array (concatenate)(w946, w947) -> (w943:u32[])
                          }
                        }
                        frame #1 {
                          n518 = local read "Average"() -> (w968:bool)
                          n519 = case shown="True" w968 {
                            selector: w968 -> [_ w985]
                            tunnel: w973 -> [_ w990]
                            tunnel: w972 -> [w978 w989]
                            tunnel: w971 -> [w977 w988]
                            tunnel: [w977 w987] -> w970
                            tunnel: [w978 w986] -> w969
                            tunnel: w962 -> [w975 w984]
                            tunnel: w967 -> [w976 w983]
                            tunnel: [w976 w981] -> w965
                            tunnel: [w975 w982] -> w966
                            tunnel: w964 -> [w974 w980]
                            tunnel: [w974 w979] -> w963
                            frame False {
                            }
                            frame True {
                              n520 = stacked-sequence {
                                seq-local: [w993 _] -> [_ w1032]
                                tunnel: w990 -> [w1001 _]
                                tunnel: w989 -> [w1000 _]
                                tunnel: w988 -> [w999 _]
                                tunnel: [w996 _] -> w987
                                tunnel: [w995 _] -> w986
                                tunnel: w985 -> [w994 _]
                                tunnel: w984 -> [_ w1033]
                                tunnel: w983 -> [w993 _]
                                tunnel: [_ w1028] -> w982
                                tunnel: [_ w1025] -> w981
                                tunnel: w980 -> [_ w1019]
                                tunnel: [_ w1018] -> w979
                                frame #0 {
                                n521 = local read "iterations"() -> (w992:i32)
                                n522 = To Unsigned Long Integer(number=w1001) -> (unsigned 32bit integer=w998:u32)
                                n523 = call "C8855_WFAVG.vi"("iteration # in"=w992, "2D populated array in"=w999, "Input Array"=w1000, "Number of Averages"=w998, "Average ON/OFF"=w994) -> ("iteration # out"=→"iterations":i32, "2D populated array out"=w996:dbl[][], "Averaged Array"=w995:dbl[], "Average ON/OFF"=w997:bool)  [unwired: 3 in]
                                n524 = shared-variable ".\\Shared Variables.lvlib\\C8855-Avg"(w997) -> ()  [unwired: 1 in, 1 out]
                                }
                                frame #1 {
                                n525 = Unbundle By Name(w1019) -> ("C8855 Measurement Parameters"=w1020:T8)
                                n526 = local read "Triggers"() -> (w1024:enum32{"Software", "External"})
                                n527 = local read "Measurement points"() -> (w1022:u32)
                                n528 = local read "C8855 gate time"() -> (w1021:i32)
                                n529 = flat-sequence {
                                tunnel: w1011 -> [w1041]
                                tunnel: [w1041] -> w1010
                                tunnel: ["wait between function nodes in averaging mode (ms)"] -> w1003
                                frame #0 {
                                n530 = Wait (ms)(milliseconds to wait="wait between function nodes in averaging mode (ms)") -> ()  [unwired: 1 out]
                                }
                                }
                                n531 = dll-call lib="C:/Users/physrin/Documents/LSLV/Labview Laser Spectroscopy/C8855-01api.dll" fn="_C8855CountStop@4"(error in=w1032, "Handle"=w1033) -> (error out=w1011:errorcluster, "Handle"=w1031:i32)  [unwired: 2 in, 2 out]
                                n532 = call "c8855_calc_measurement_params_sub.vi"("measurement params"=w1020, "Gate time"=w1021, "Measurement points"=w1022) -> ("measurement params out"=w1014:T9)  [unwired: 2 in]
                                n533 = case shown="\"External\", Default" w1024 {
                                tunnel: [u8 0 u8 1] -> w1027
                                frame "Software" {
                                }
                                frame "External", Default {
                                }
                                }
                                n534 = Unbundle By Name(w1014) -> ("Gate time"=w1013:u8, "Number of gates"=w1012:u16)
                                n535 = flat-sequence {
                                tunnel: w1009 -> [w1039]
                                tunnel: [w1039] -> w1008
                                tunnel: w1003 -> [w1038]
                                tunnel: [w1038] -> w1002
                                frame #0 {
                                n536 = Wait (ms)(milliseconds to wait=w1038) -> ()  [unwired: 1 out]
                                }
                                }
                                n537 = dll-call lib="C:/Users/physrin/Documents/LSLV/Labview Laser Spectroscopy/C8855-01api.dll" fn="_C8855Reset@4"(error in=w1010, "Handle"=w1031) -> (error out=w1009:errorcluster, "Handle"=w1030:i32)  [unwired: 3 in, 1 out]
                                n538 = flat-sequence {
                                tunnel: w1007 -> [w1037]
                                tunnel: [w1037] -> w1006
                                tunnel: w1002 -> [w1036]
                                frame #0 {
                                n539 = Wait (ms)(milliseconds to wait=w1036) -> ()  [unwired: 1 out]
                                }
                                }
                                n540 = dll-call lib="C:/Users/physrin/Documents/LSLV/Labview Laser Spectroscopy/C8855-01api.dll" fn="_C8855Setup@16"(error in=w1008, "Handle"=w1030, "Gatetime"=w1013, "Transmode"=u8 2, "Number of gate"=w1012) -> (error out=w1007:errorcluster, "Handle"=w1029:i32)  [unwired: 5 in, 2 out]
                                n541 = To Long Integer(number=w1012) -> (32bit integer=w1016:i32)
                                n542 = dll-call lib="C:/Users/physrin/Documents/LSLV/Labview Laser Spectroscopy/C8855-01api.dll" fn="_C8855CountStart@8"(error in=w1006, "Handle"=w1029, "TriggerMode"=w1027) -> (error out=w1005:errorcluster, "Handle"=w1028:i32)  [unwired: 3 in, 2 out]
                                n543 = Initialize Array(u32 0 ("element"), w1016) -> (w1015:u32[])
                                n544 = flat-sequence {
                                tunnel: w1005 -> [w1035]
                                tunnel: [w1035] -> w1004
                                tunnel: w1002 -> [w1034]
                                frame #0 {
                                n545 = Wait (ms)(milliseconds to wait=w1034) -> ()  [unwired: 1 out]
                                }
                                }
                                n546 = Bundle By Name(cluster=w1019, "C8855 Measurement Parameters"=w1014, "Data Buffer"=w1015) -> (w1018:T6)
                                n547 = shared-variable ".\\Shared Variables.lvlib\\Gate Open"(FALSE ("Gate Open"), error in=w1004) -> (error out=w1025:errorcluster)
                                }
                              }
                            }
                          }
                        }
                      }
                      "Numeric" <- w919
                    }
                  }
                }
                n548 = local read "Measurement Time (sec)"() -> (w832:dbl)
                n549 = local read "Measurement points"() -> (w831:u32)
                n550 = Divide(x=w832, y=w831) -> (x/y=w830:dbl)
                n551 = case shown="False" w846 {
                  tunnel: [Control_4."C8855-Count Stop" ("Enum") Control_4."C8855-Reset" ("Enum")] -> w847
                  frame False {
                  }
                  frame True {
                    n552 = One Button Dialog(message="C8855ReadData()\nChange to a longer gate time.") -> ()  [unwired: 1 in, 1 out]
                  }
                }
                n553 = Add Array Elements(numeric array=w838) -> (sum=w833:dbl)
                n554 = To Unsigned Long Integer(number=w833) -> (unsigned 32bit integer=→"Counts":u32)
                n555 = To Time Stamp(1:0.0) -> (0:w843:timestamp)
                n556 = To Double Precision Float(number=w833) -> (double precision float=w849:dbl)
                n557 = Bundle By Name("t0"=w843, "dt"=w830, "Y"=w838) -> (w842:waveform(dbl))  [unwired: 1 in]
                n558 = To Double Precision Float(number=w842) -> (double precision float=→"Waveform Graph C8855":waveform(dbl))
                n559 = shared-variable ".\\Shared Variables.lvlib\\Area"(w849, error in=w848) -> (error out=w845:errorcluster)
                n560 = disable-structure shown="Disabled" {
                  frame Disabled {
                    n561 = property on="Waveform Graph" class="WFGraph (strict)"("XScale.Minimum"=0.0 ("X Scale.Range:Minimum")) -> ()  [unwired: 2 in, 2 out]
                  }
                  frame Enabled {
                  }
                }
              }
              frame "C8855-Close" {
                n562 = dll-call lib="C:/Users/physrin/Documents/LSLV/Labview Laser Spectroscopy/C8855-01api.dll" fn="_C8855Close@4"(error in=w1052, "Handle"=w1046) -> (error out=w1045:errorcluster, "Handle"=w1051:i32)  [unwired: 2 in, 2 out]
                n563 = Equal?(x=w1051, y=-1) -> (x = y?=w1049:bool)
                n564 = case shown="False" w1049 {
                  tunnel: [Control_4."Idle" ("Enum") Control_4."Idle" ("Enum")] -> w1047
                  tunnel: w1045 -> [w1054 w1057]
                  tunnel: [w1053 w1057] -> w1044
                  frame False {
                    w1055 = FALSE ("C8855_init")
                    n565 = shared-variable ".\\Shared Variables.lvlib\\C8855_init"(w1055, error in=w1054) -> (error out=w1053:errorcluster)
                    n566 = local write "C8855 Initialised"(w1055) -> ()
                  }
                  frame True {
                    n567 = One Button Dialog(message="C8855Close()\nCheck C8855.", button name ("OK")="OK" ("F button name (\"Cancel\")")) -> ()  [unwired: 1 out]
                  }
                }
              }
              frame "C8855-Count Stop" {
                n568 = dll-call lib="C:/Users/physrin/Documents/LSLV/Labview Laser Spectroscopy/C8855-01api.dll" fn="_C8855CountStop@4"(error in=w1069, "Handle"=w1062) -> (error out=w1064:errorcluster, "Error"=w1068:i32, "Handle"=w1061:i32)  [unwired: 2 in, 1 out]
                n569 = Equal?(x=w1068, y=0) -> (x = y?=w1066:bool)
                n570 = case shown="False" w1066 {
                  tunnel: [Control_4."C8855-Reset" ("Enum") w1071] -> w1065
                  frame False {
                  }
                  frame True {
                    n571 = Two Button Dialog(message="C8855CountStop( )\nCheck C8855.", 1:"Continue" ("F button name (\"Cancel\")"), 2:"Shutdown" ("T button name (\"OK\")")) -> (T button?=w1072:bool)
                    n572 = case shown="False" w1072 {
                      tunnel: [Control_4."C8855-Reset" ("Enum") Control_4."C8855-Close" ("Enum")] -> w1071
                      frame False {
                      }
                      frame True {
                        n573 = Quit LabVIEW(quit? (T)=TRUE) -> ()
                      }
                    }
                  }
                }
              }
            }
            n574 = shared-variable ".\\Shared Variables.lvlib\\Shutdown"() -> (w595:bool)  [unwired: 1 in, 1 out]
            n575 = Enqueue Element(queue=w603, element=w602, error in (no error)=w597) -> (queue out=w599:refnum<queue>, error out=w596:errorcluster)  [unwired: 1 in, 1 out]
            n576 = Wait (ms)(milliseconds to wait=u32 100) -> ()  [unwired: 1 out]
          }
          n577 = Release Queue(queue=w587, error in (no error)=w586) -> (error out=w585:errorcluster)  [unwired: 1 in, 2 out]
          n578 = call <vilib>:"Simple Error Handler.vi"("error in (no error)"=w585) -> ("error out"=→"error out 2":errorcluster)  [unwired: 4 in, 4 out]
        }
      }
      n579 = while {
        tunnel: w143 -> [w1092]
        tunnel: w130 -> [w1090]
        shift-right: [w1089] -> _
        shift-left: w123 -> [w1093]
        shift-right: [w1086] -> w145
        shift-left: w146 -> [w1088]
        shift-right: [w1083] -> w140
        shift-left: w138 -> [w1082]
        tunnel: w136 -> [w1080]
        stop <- w1079 stop-if-true
        n580 = Dequeue Element(queue=w1088, error in (no error)=w1082) -> (element=w1091:T2, error out=w1085:errorcluster)  [unwired: 1 in, 2 out]
        "Medium Loop" <- w1091
        n581 = case shown="\"GL302 Goto WL\"" w1091 {
          tunnel: w1093 -> [w1097 w1104 w1116 w1489 w1537 w1544 w1605 w2092 w2189 w2266 w2283 w2297 w2307]
          tunnel: w1092 -> [_ w1105 w1123 _ _ _ _ _ _ _ w2279 w2293 w2309]
          tunnel: w1090 -> [_ _ w1122 _ _ _ w1603 _ _ _ _ _ _]
          tunnel: [w1097 w1104 w1121 w1488 w1537 w1544 w1600 w2092 w2189 w2266 w2283 w2297 w2307] -> w1089
          tunnel: [w1096 w1102 w1120 w1486 w1532 w1541 w1602 w2093 w2190 w2267 w2281 w2295 w2304] -> w1087
          tunnel: w1085 -> [w1095 w1103 w1119 w1487 w1533 w1545 w1604 w2096 w2193 w2270 w2284 w2298 w2308]
          tunnel: [w1095 w1101 w1118 w1485 w1531 w1543 w1601 w2095 w2192 w2269 w2274 w2288 w2306] -> w1084
          tunnel: w1080 -> [_ _ _ _ _ w1540 w1599 w2085 w2187 w2265 _ _ _]
          frame "Idle" {
            n582 = Unbundle By Name(w1095) -> ("status"=w1094:bool)
            n583 = case shown="False" w1094 {
              tunnel: [Control_3."Idle" Control_3."Error Handler"] -> w1096
              frame False {
              }
              frame True {
              }
            }
          }
          frame "iHR550 Fixed Wavelength", Default {
            n584 = stacked-sequence {
              tunnel: w1105 -> [w1110 _]
              tunnel: w1103 -> [w1109 _]
              tunnel: [w1108 _] -> w1101
              frame #0 {
                n585 = call "JYMoveToWavelength.vi"("error in (no error)"=w1109, "Target WL"="Target WL", "RefNum In"=w1110) -> ("error out"=w1112:errorcluster, "Refnum Out"=w1113:refnum<k7>)  [unwired: 1 in, 1 out]
                n586 = call "JYGetCurrentWL.vi"("error in (no error)"=w1112, "JYMONOLib.IJYMonoReqd"=w1113) -> ("error out"=w1108:errorcluster, "Current WL"=w1111:dbl)  [unwired: 5 in, 3 out]
                n587 = local write "Current WL"(w1111) -> ()
              }
              frame #1 {
                n588 = local write "Target WL"(FALSE ("Target WL")) -> ()
              }
            }
            n589 = Unbundle By Name(w1101) -> ("status"=w1100:bool)
            n590 = case shown="False" w1100 {
              tunnel: [Control_3."Idle" Control_3."Error Handler"] -> w1102
              frame False {
              }
              frame True {
              }
            }
          }
          frame "iHR550 Interval Movement" {
            n591 = stacked-sequence {
              seq-local: [w1130 _ _] -> [_ w1132 _]
              tunnel: w1116 -> [w1129 _ _]
              tunnel: w1123 -> [_ w1137 _]
              tunnel: w1122 -> [_ w1136 _]
              tunnel: [_ w1135 _] -> w1121
              tunnel: w1119 -> [_ w1134 _]
              tunnel: [_ w1133 _] -> w1118
              frame #0 {
                n592 = Bundle By Name(cluster=w1129, "Spec Plot"=cluster{"Wavelength":dbl[], "Int WF":dbl[]} {"Wavelength"=[], "Int WF"=[]}) -> (w1130:T6)
              }
              frame #1 {
                n593 = case shown="\"Uninterrupted\"" "Scan Mode" {
                  tunnel: w1132 -> [w1147 w1289]
                  tunnel: w1137 -> [w1146 w1288]
                  tunnel: w1136 -> [w1145 w1287]
                  tunnel: [w1144 w1286] -> w1135
                  tunnel: w1134 -> [w1143 w1285]
                  tunnel: [w1142 w1284] -> w1133
                  frame "Interrupted " {
                    n594 = stacked-sequence {
                      seq-local: [w1156 _] -> [_ w1165]
                      seq-local: [w1150 _] -> [_ w1167]
                      tunnel: w1147 -> [_ w1166]
                      tunnel: [_ w1164] -> w1142
                      tunnel: w1146 -> [w1155 _]
                      tunnel: [_ w1162] -> w1144
                      tunnel: w1145 -> [_ w1163]
                      tunnel: w1143 -> [w1152 _]
                      frame #0 {
                        n595 = local write "state"(0.0 ("state")) -> ()
                        n596 = local read "Start Wavelength"() -> (w1159:dbl)
                        n597 = call "JYMoveToWavelength.vi"("error in (no error)"=w1152, "Target WL"=w1159, "RefNum In"=w1155) -> ("error out"=w1157:errorcluster, "Refnum Out"=w1158:refnum<k7>)  [unwired: 1 in, 1 out]
                        n598 = call "JYGetCurrentWL.vi"("error in (no error)"=w1157, "JYMONOLib.IJYMonoReqd"=w1158) -> ("error out"=w1154:errorcluster, "Current WL"=w1160:dbl, "JYMONOLib.IJYMonoReqd 2"=w1156:refnum<k7>)  [unwired: 5 in, 2 out]
                        n599 = local write "Current WL"(w1160) -> ()
                        n600 = shared-variable ".\\Shared Variables.lvlib\\mono tick"(u32 1 ("mono tick"), error in=w1154) -> (error out=w1151:errorcluster)
                        n601 = shared-variable ".\\Shared Variables.lvlib\\osc tick"(u32 0 ("osc tick"), error in=w1151) -> (error out=w1150:errorcluster)
                      }
                      frame #1 {
                        n602 = while {
                          tunnel: w1167 -> [w1192]
                          tunnel: w1165 -> [w1188]
                          shift-right: [w1187] -> w1162
                          shift-left: w1166 -> [w1191]
                          tunnel: [w1185] -> w1164
                          tunnel: w1163 -> [w1186]
                          stop <- w1189 continue-if-true
                          n603 = local write "state"(2.0 ("state")) -> ()
                          n604 = Build Array("Forward", "Backward") -> (w1173:bool[])
                          n605 = shared-variable ".\\Shared Variables.lvlib\\C8855_init"() -> (w1169:bool)  [unwired: 1 in, 1 out]
                          n606 = local read "Start Wavelength"() -> (w1184:dbl)
                          n607 = local read "Current WL"() -> (w1183:dbl)
                          n608 = Search 1D Array(1D array=w1173, element=TRUE) -> (index of element=w1171:i32)  [unwired: 1 in]
                          n609 = Increment(x=w1171) -> (x+1=w1170:i32)
                          n610 = local read "End Wavelength"() -> (w1190:dbl)
                          n611 = case shown="2" w1170 {
                            tunnel: w1192 -> [w1194 w1203 w1253]
                            tunnel: w1191 -> [w1195 w1202 w1257]
                            tunnel: w1188 -> [_ w1201 w1254]
                            tunnel: w1183 -> [_ w1200 w1255]
                            tunnel: [w1195 w1199 w1256] -> w1187
                            tunnel: [w1194 w1198 w1252] -> w1185
                            tunnel: w1186 -> [_ w1197 _]
                            tunnel: w1169 -> [_ w1196 _]
                            frame 0, Default {
                              n612 = local write "state"(3.0 ("state")) -> ()
                            }
                            frame 1 {
                              n613 = stacked-sequence {
                                tunnel: w1203 -> [w1206 _]
                                tunnel: w1202 -> [w1216 _]
                                tunnel: w1201 -> [w1217 _]
                                tunnel: w1200 -> [w1215 _]
                                tunnel: [w1214 _] -> w1199
                                tunnel: [w1213 _] -> w1198
                                tunnel: w1197 -> [w1212 _]
                                tunnel: w1196 -> [w1204 _]
                                frame #0 {
                                n614 = shared-variable ".\\Shared Variables.lvlib\\mono tick"(error in=w1206) -> (w1210:u32, error out=w1207:errorcluster)
                                n615 = shared-variable ".\\Shared Variables.lvlib\\osc tick"(error in=w1207) -> (w1209:u32, error out=w1205:errorcluster)
                                n616 = case shown="True" w1204 {
                                tunnel: w1212 -> [w1221 _]
                                tunnel: [w1220 w1222] -> w1211
                                tunnel: w1205 -> [w1218 w1222]
                                frame False {
                                n617 = Enqueue Element(queue=w1221, element=Control_4."Waveform Queries" ("Enum"), error in (no error)=w1218) -> (error out=w1220:errorcluster)  [unwired: 1 in, 2 out]
                                }
                                frame True {
                                }
                                }
                                n618 = Less?(x=w1210, y=w1209) -> (x < y?=w1208:bool)
                                n619 = case shown="True" w1208 {
                                tunnel: w1217 -> [_ w1244]
                                tunnel: w1211 -> [w1224 w1240]
                                tunnel: w1216 -> [w1225 w1236]
                                tunnel: w1215 -> [_ w1233]
                                tunnel: [w1225 w1231] -> w1214
                                tunnel: [w1224 w1229] -> w1213
                                frame False {
                                n620 = local write "state"(6.0 ("state")) -> ()
                                }
                                frame True {
                                n621 = Unbundle By Name(w1236) -> ("Spec Plot.Wavelength"=w1238:dbl[], "Spec Plot.Int WF"=w1239:dbl[])
                                n622 = local read "Interval Wavelength"() -> (w1234:dbl)
                                n623 = shared-variable ".\\Shared Variables.lvlib\\Area"(error in=w1240) -> (w1237:dbl, error out=w1242:errorcluster)
                                n624 = Add(x=w1233, y=w1234) -> (x+y=w1232:dbl)
                                n625 = Build Array (concatenate)(w1238, w1233) -> (w1228:dbl[])
                                n626 = Build Array (concatenate)(w1239, w1237) -> (w1227:dbl[])
                                n627 = Bundle By Name(cluster=w1236, "Spec Plot.Wavelength"=w1228, "Spec Plot.Int WF"=w1227) -> (w1231:T6)
                                n628 = call "JYMoveToWavelength.vi"("error in (no error)"=w1242, "Target WL"=w1232, "RefNum In"=w1244) -> ("error out"=w1241:errorcluster, "Refnum Out"=w1243:refnum<k7>)  [unwired: 1 in, 1 out]
                                n629 = call "JYGetCurrentWL.vi"("error in (no error)"=w1241, "JYMONOLib.IJYMonoReqd"=w1243) -> ("error out"=w1230:errorcluster, "Current WL"=w1235:dbl)  [unwired: 5 in, 3 out]
                                n630 = local write "Current WL"(w1235) -> ()
                                n631 = Bundle(w1228, w1227) -> (w1226:cluster{dbl[], dbl[]})  [unwired: 1 in]
                                n632 = flat-sequence {
                                tunnel: w1230 -> [w1249]
                                tunnel: [w1246] -> w1229
                                frame #0 {
                                n633 = Tick Count (ms)() -> (millisecond timer value=w1248:u32)
                                n634 = shared-variable ".\\Shared Variables.lvlib\\mono tick"(w1248, error in=w1249) -> (error out=w1247:errorcluster)
                                n635 = shared-variable ".\\Shared Variables.lvlib\\Gate Open"(TRUE ("Gate Open"), error in=w1247) -> (error out=w1246:errorcluster)
                                }
                                }
                                n636 = local write "XY Graph"(w1226) -> ()
                                }
                                }
                                }
                                frame #1 {
                                n637 = local write "state"(4.0 ("state")) -> ()
                                }
                              }
                            }
                            frame 2 {
                              n638 = stacked-sequence {
                                tunnel: w1257 -> [w1279 _]
                                tunnel: [w1278 _] -> w1256
                                tunnel: w1255 -> [w1277 _]
                                tunnel: w1254 -> [w1276 _]
                                tunnel: w1253 -> [w1274 _]
                                tunnel: [w1275 _] -> w1252
                                frame #0 {
                                n639 = local read "Interval Wavelength"() -> (w1273:dbl)
                                n640 = Unbundle By Name(w1279) -> ("Spec Plot.Wavelength"=w1261:dbl[], "Spec Plot.Int WF"=w1265:dbl[])
                                n641 = Subtract(x=w1277, y=w1273) -> (x-y=w1272:dbl)
                                n642 = Array Size(array=w1261) -> (size(s)=w1264:i32)
                                n643 = Array Size(array=w1265) -> (size(s)=w1268:i32)
                                n644 = call "JYMoveToWavelength.vi"("error in (no error)"=w1274, "Target WL"=w1272, "RefNum In"=w1276) -> ("error out"=w1269:errorcluster, "Refnum Out"=w1271:refnum<k7>)  [unwired: 1 in, 1 out]
                                n645 = Subtract(x=w1268, y=1) -> (x-y=w1266:i32)
                                n646 = Subtract(x=w1264, y=1) -> (x-y=w1262:i32)
                                n647 = Delete From Array(array=w1265, index=w1266) -> (array with subset deleted=w1259:dbl[])  [unwired: 1 in, 1 out]
                                n648 = Delete From Array(array=w1261, index=w1262) -> (array with subset deleted=w1260:dbl[])  [unwired: 1 in, 1 out]
                                n649 = call "JYGetCurrentWL.vi"("error in (no error)"=w1269, "JYMONOLib.IJYMonoReqd"=w1271) -> ("error out"=w1275:errorcluster, "Current WL"=w1270:dbl)  [unwired: 5 in, 3 out]
                                n650 = local write "Current WL"(w1270) -> ()
                                n651 = Bundle By Name(cluster=w1279, "Spec Plot.Wavelength"=w1260, "Spec Plot.Int WF"=w1259) -> (w1278:T6)
                                n652 = Bundle("Wavelength"=w1260, "Int WF"=w1259) -> (w1258:cluster{"Wavelength":dbl[], "Int WF":dbl[]})  [unwired: 1 in]
                                n653 = local write "XY Graph"(w1258) -> ()
                                }
                                frame #1 {
                                n654 = local write "Backward"(FALSE ("Backward")) -> ()
                                }
                              }
                              n655 = local write "state"(5.0 ("state")) -> ()
                            }
                          }
                          n656 = Less Or Equal?(x=w1184, y=w1183) -> (x <= y?=w1180:bool)
                          n657 = Greater Or Equal?(x=w1190, y=w1183) -> (x >= y?=w1181:bool)
                          n658 = And(x=w1181, y=w1180) -> (x .and. y?=w1182:bool)
                          n659 = local read "Abort Scan"() -> (w1177:bool)
                          n660 = Unbundle By Name(w1185) -> ("status"=w1179:bool)
                          n661 = Not(x=w1177) -> (.not. x?=w1176:bool)
                          n662 = Not(x=w1179) -> (.not. x?=w1178:bool)
                          n663 = Compound Arithmetic op=AND(w1178, w1182, w1176) -> (w1189:bool)
                        }
                        "state" <- 1.0 ("state")
                      }
                    }
                    n664 = Unbundle By Name(w1144) -> ("Spec Plot.Wavelength"=w1141:dbl[], "Spec Plot.Int WF"=w1140:dbl[])
                    n665 = Bundle("Wavelength"=w1141, "Int WF"=w1140) -> (→"XY Graph":cluster{"Wavelength":dbl[], "Int WF":dbl[]})  [unwired: 1 in]
                  }
                  frame "Uninterrupted" {
                    n666 = Less?(x="Start Wavelength", y="End Wavelength") -> (x < y?=w1292:bool)
                    n667 = case shown="False" w1292 {
                      tunnel: w1289 -> [w1298 w1391]
                      tunnel: w1288 -> [w1297 w1390]
                      tunnel: [w1296 w1386] -> w1286
                      tunnel: w1287 -> [w1295 w1389]
                      tunnel: w1285 -> [w1294 w1387]
                      tunnel: [w1293 w1388] -> w1284
                      frame False {
                        n668 = stacked-sequence {
                          seq-local: [w1306 _] -> [_ w1315]
                          seq-local: [w1300 _] -> [_ w1314]
                          tunnel: w1298 -> [_ w1316]
                          tunnel: [_ w1313] -> w1293
                          tunnel: w1297 -> [w1305 _]
                          tunnel: [_ w1312] -> w1296
                          tunnel: w1295 -> [_ w1311]
                          tunnel: w1294 -> [w1302 _]
                          frame #0 {
                            n669 = local read "Start Wavelength"() -> (w1309:dbl)
                            n670 = call "JYMoveToWavelength.vi"("error in (no error)"=w1302, "Target WL"=w1309, "RefNum In"=w1305) -> ("error out"=w1310:errorcluster, "Refnum Out"=w1307:refnum<k7>)  [unwired: 1 in, 1 out]
                            n671 = call "JYGetCurrentWL.vi"("error in (no error)"=w1310, "JYMONOLib.IJYMonoReqd"=w1307) -> ("error out"=w1303:errorcluster, "Current WL"=w1308:dbl, "JYMONOLib.IJYMonoReqd 2"=w1306:refnum<k7>)  [unwired: 5 in, 2 out]
                            n672 = local write "Current WL"(w1308) -> ()
                            n673 = shared-variable ".\\Shared Variables.lvlib\\mono tick"(u32 1 ("mono tick"), error in=w1303) -> (error out=w1301:errorcluster)
                            n674 = shared-variable ".\\Shared Variables.lvlib\\osc tick"(u32 0 ("osc tick"), error in=w1301) -> (error out=w1300:errorcluster)
                          }
                          frame #1 {
                            n675 = while {
                              shift-right: [w1321] -> w1312
                              shift-left: w1316 -> [w1328]
                              tunnel: w1315 -> [w1329]
                              tunnel: w1314 -> [w1331]
                              tunnel: [w1326] -> w1313
                              tunnel: w1311 -> [w1327]
                              stop <- w1322 continue-if-true
                              n676 = shared-variable ".\\Shared Variables.lvlib\\C8855_init"() -> (w1317:bool)  [unwired: 1 in, 1 out]
                              n677 = local read "Current WL"() -> (w1330:dbl)
                              n678 = stacked-sequence {
                                tunnel: w1331 -> [w1336 _]
                                tunnel: w1330 -> [w1346 _]
                                tunnel: w1329 -> [w1345 _]
                                tunnel: [w1344 _] -> w1326
                                tunnel: [w1343 _] -> w1321
                                tunnel: w1328 -> [w1342 _]
                                tunnel: w1327 -> [w1335 _]
                                tunnel: w1317 -> [w1337 w1377]
                                frame #0 {
                                n679 = case shown="False" w1337 {
                                tunnel: w1336 -> [w1349 w1351]
                                tunnel: w1335 -> [w1348 _]
                                tunnel: [w1347 w1351] -> w1334
                                frame False {
                                n680 = Enqueue Element(queue=w1348, element=Control_4."Waveform Queries" ("Enum"), error in (no error)=w1349) -> (error out=w1347:errorcluster)  [unwired: 1 in, 2 out]
                                }
                                frame True {
                                }
                                }
                                n681 = shared-variable ".\\Shared Variables.lvlib\\mono tick"() -> (w1340:u32, error out=w1338:errorcluster)  [unwired: 1 in]
                                n682 = shared-variable ".\\Shared Variables.lvlib\\osc tick"(error in=w1338) -> (w1341:u32)  [unwired: 1 out]
                                n683 = Less?(x=w1340, y=w1341) -> (x < y?=w1339:bool)
                                n684 = case shown="True" w1339 {
                                tunnel: [w1352 w1371] -> w1343
                                tunnel: w1334 -> [w1353 w1368]
                                tunnel: [w1353 w1354] -> w1344
                                tunnel: w1342 -> [w1352 w1356]
                                tunnel: w1346 -> [_ w1358]
                                tunnel: w1345 -> [_ w1364]
                                frame False {
                                }
                                frame True {
                                n685 = Unbundle By Name(w1356) -> ("Spec Plot.Wavelength"=w1366:dbl[], "Spec Plot.Int WF"=w1365:dbl[])
                                n686 = shared-variable ".\\Shared Variables.lvlib\\Area"(error in=w1368) -> (w1369:dbl, error out=w1361:errorcluster)
                                n687 = Build Array (concatenate)(w1366, w1358) -> (w1367:dbl[])
                                n688 = Build Array (concatenate)(w1365, w1369) -> (w1370:dbl[])
                                n689 = Bundle By Name(cluster=w1356, "Spec Plot.Wavelength"=w1367, "Spec Plot.Int WF"=w1370) -> (w1371:T6)
                                n690 = local read "Interval Wavelength"() -> (w1359:dbl)
                                n691 = Subtract(x=w1358, y=w1359) -> (x-y=w1357:dbl)
                                n692 = call "JYMoveToWavelength.vi"("error in (no error)"=w1361, "Target WL"=w1357, "RefNum In"=w1364) -> ("error out"=w1360:errorcluster, "Refnum Out"=w1363:refnum<k7>)  [unwired: 1 in, 1 out]
                                n693 = flat-sequence {
                                tunnel: w1355 -> [w1376]
                                tunnel: [w1373] -> w1354
                                frame #0 {
                                n694 = Tick Count (ms)() -> (millisecond timer value=w1375:u32)
                                n695 = shared-variable ".\\Shared Variables.lvlib\\mono tick"(w1375, error in=w1376) -> (error out=w1374:errorcluster)
                                n696 = shared-variable ".\\Shared Variables.lvlib\\Gate Open"(TRUE ("Gate Open"), error in=w1374) -> (error out=w1373:errorcluster)
                                }
                                }
                                n697 = call "JYGetCurrentWL.vi"("error in (no error)"=w1360, "JYMONOLib.IJYMonoReqd"=w1363) -> ("error out"=w1355:errorcluster, "Current WL"=w1362:dbl)  [unwired: 5 in, 3 out]
                                n698 = local write "Current WL"(w1362) -> ()
                                }
                                }
                                }
                                frame #1 {
                                n699 = case shown="False" w1377 {
                                frame False {
                                n700 = local read "Delay (s)"() -> (w1380:dbl)
                                n701 = Multiply(x=w1380, y=1000.0) -> (x*y=w1378:dbl)
                                n702 = To Unsigned Long Integer(number=w1378) -> (unsigned 32bit integer=w1381:u32)
                                n703 = Wait (ms)(milliseconds to wait=w1381) -> ()  [unwired: 1 out]
                                }
                                frame True {
                                n704 = local read "Delay (s)"() -> (w1385:dbl)
                                n705 = Multiply(x=w1385, y=1000.0) -> (x*y=w1383:dbl)
                                n706 = To Unsigned Long Integer(number=w1383) -> (unsigned 32bit integer=w1382:u32)
                                n707 = Wait (ms)(milliseconds to wait=w1382) -> ()  [unwired: 1 out]
                                }
                                }
                                }
                              }
                              n708 = local read "End Wavelength"() -> (w1333:dbl)
                              n709 = local read "Abort Scan"() -> (w1324:bool)
                              n710 = Unbundle By Name(w1321) -> ("Spec Plot.Wavelength"=w1320:dbl[], "Spec Plot.Int WF"=w1319:dbl[])
                              n711 = Unbundle By Name(w1326) -> ("status"=w1325:bool)
                              n712 = Less Or Equal?(x=w1333, y=w1330) -> (x <= y?=w1332:bool)
                              n713 = Not(x=w1324) -> (.not. x?=w1323:bool)
                              n714 = Compound Arithmetic op=AND(w1325, w1332, w1323) -> (w1322:bool)
                              n715 = Bundle("Wavelength"=w1320, "Int WF"=w1319) -> (w1318:cluster{"Wavelength":dbl[], "Int WF":dbl[]})  [unwired: 1 in]
                              n716 = local write "XY Graph"(w1318) -> ()
                            }
                          }
                        }
                      }
                      frame True {
                        n717 = stacked-sequence {
                          seq-local: [w1399 _] -> [_ w1408]
                          seq-local: [w1392 _] -> [_ w1409]
                          tunnel: w1391 -> [_ w1405]
                          tunnel: [_ w1407] -> w1388
                          tunnel: w1390 -> [w1398 _]
                          tunnel: w1389 -> [_ w1406]
                          tunnel: w1387 -> [w1395 _]
                          tunnel: [_ w1404] -> w1386
                          frame #0 {
                            n718 = local read "Start Wavelength"() -> (w1401:dbl)
                            n719 = call "JYMoveToWavelength.vi"("error in (no error)"=w1395, "Target WL"=w1401, "RefNum In"=w1398) -> ("error out"=w1403:errorcluster, "Refnum Out"=w1402:refnum<k7>)  [unwired: 1 in, 1 out]
                            n720 = call "JYGetCurrentWL.vi"("error in (no error)"=w1403, "JYMONOLib.IJYMonoReqd"=w1402) -> ("error out"=w1397:errorcluster, "Current WL"=w1400:dbl, "JYMONOLib.IJYMonoReqd 2"=w1399:refnum<k7>)  [unwired: 5 in, 2 out]
                            n721 = local write "Current WL"(w1400) -> ()
                            n722 = shared-variable ".\\Shared Variables.lvlib\\mono tick"(u32 1 ("mono tick"), error in=w1397) -> (error out=w1393:errorcluster)
                            n723 = shared-variable ".\\Shared Variables.lvlib\\osc tick"(u32 0 ("osc tick"), error in=w1393) -> (error out=w1392:errorcluster)
                          }
                          frame #1 {
                            n724 = while {
                              shift-right: [w1411] -> w1404
                              shift-left: w1405 -> [w1412]
                              tunnel: w1409 -> [w1424]
                              tunnel: w1408 -> [w1423]
                              tunnel: [w1419] -> w1407
                              tunnel: w1406 -> [w1420]
                              stop <- w1414 continue-if-true
                              n725 = shared-variable ".\\Shared Variables.lvlib\\C8855_init"() -> (w1410:bool)  [unwired: 1 in, 1 out]
                              n726 = local read "End Wavelength"() -> (w1421:dbl)
                              n727 = local read "Current WL"() -> (w1422:dbl)
                              n728 = stacked-sequence {
                                seq-local: [w1429 _ _] -> [_ w1468 _]
                                seq-local: [_ w1467 _] -> [_ _ w1472]
                                tunnel: w1412 -> [w1436 _ _]
                                tunnel: w1424 -> [w1425 _ _]
                                tunnel: w1422 -> [w1435 _ _]
                                tunnel: w1423 -> [w1434 _ _]
                                tunnel: [w1433 _ _] -> w1419
                                tunnel: w1420 -> [w1427 _ _]
                                tunnel: [_ _ w1472] -> w1413
                                tunnel: w1410 -> [w1428 _ w1471]
                                frame #0 {
                                n729 = case shown="True" w1428 {
                                tunnel: w1427 -> [w1439 _]
                                tunnel: [w1438 w1441] -> w1426
                                tunnel: w1425 -> [w1437 w1441]
                                frame False {
                                n730 = Enqueue Element(queue=w1439, element=Control_4."Waveform Queries" ("Enum"), error in (no error)=w1437) -> (error out=w1438:errorcluster)  [unwired: 1 in, 2 out]
                                }
                                frame True {
                                }
                                }
                                n731 = shared-variable ".\\Shared Variables.lvlib\\mono tick"() -> (w1432:u32)  [unwired: 1 in, 1 out]
                                n732 = shared-variable ".\\Shared Variables.lvlib\\osc tick"() -> (w1430:u32)  [unwired: 1 in, 1 out]
                                n733 = Less?(x=w1432, y=w1430) -> (x < y?=w1431:bool)
                                n734 = case shown="True" w1431 {
                                tunnel: w1426 -> [w1442 w1446]
                                tunnel: w1436 -> [w1443 w1455]
                                tunnel: w1435 -> [_ w1450]
                                tunnel: w1434 -> [_ w1459]
                                tunnel: [w1443 w1454] -> w1429
                                tunnel: [w1442 w1447] -> w1433
                                frame False {
                                }
                                frame True {
                                n735 = local read "Interval Wavelength"() -> (w1449:dbl)
                                n736 = Unbundle By Name(w1455) -> ("Spec Plot.Wavelength"=w1461:dbl[], "Spec Plot.Int WF"=w1460:dbl[])
                                n737 = Add(x=w1450, y=w1449) -> (x+y=w1451:dbl)
                                n738 = shared-variable ".\\Shared Variables.lvlib\\Area"(error in=w1446) -> (w1444:dbl, error out=w1445:errorcluster)
                                n739 = Build Array (concatenate)(w1461, w1450) -> (w1457:dbl[])
                                n740 = Build Array (concatenate)(w1460, w1444) -> (w1456:dbl[])
                                n741 = call "JYMoveToWavelength.vi"("error in (no error)"=w1445, "Target WL"=w1451, "RefNum In"=w1459) -> ("error out"=w1453:errorcluster, "Refnum Out"=w1458:refnum<k7>)  [unwired: 1 in, 1 out]
                                n742 = Bundle By Name(cluster=w1455, "Spec Plot.Wavelength"=w1457, "Spec Plot.Int WF"=w1456) -> (w1454:T6)
                                n743 = call "JYGetCurrentWL.vi"("error in (no error)"=w1453, "JYMONOLib.IJYMonoReqd"=w1458) -> ("error out"=w1448:errorcluster, "Current WL"=w1452:dbl)  [unwired: 5 in, 3 out]
                                n744 = local write "Current WL"(w1452) -> ()
                                n745 = flat-sequence {
                                tunnel: w1448 -> [w1466]
                                tunnel: [w1463] -> w1447
                                frame #0 {
                                n746 = Tick Count (ms)() -> (millisecond timer value=w1465:u32)
                                n747 = shared-variable ".\\Shared Variables.lvlib\\mono tick"(w1465, error in=w1466) -> (error out=w1464:errorcluster)
                                n748 = shared-variable ".\\Shared Variables.lvlib\\Gate Open"(TRUE ("Gate Open"), error in=w1464) -> (error out=w1463:errorcluster)
                                }
                                }
                                }
                                }
                                }
                                frame #1 {
                                n749 = Unbundle By Name(w1468) -> ("Spec Plot.Wavelength"=w1469:dbl[], "Spec Plot.Int WF"=w1470:dbl[])
                                n750 = Bundle("Wavelength"=w1469, "Int WF"=w1470) -> (w1467:cluster{"Wavelength":dbl[], "Int WF":dbl[]})  [unwired: 1 in]
                                n751 = local write "XY Graph"(w1467) -> ()
                                }
                                frame #2 {
                                n752 = case shown="True" w1471 {
                                frame False {
                                n753 = local read "Delay (s)"() -> (w1475:dbl)
                                n754 = Multiply(x=w1475, y=1000.0) -> (x*y=w1473:dbl)
                                n755 = To Unsigned Long Integer(number=w1473) -> (unsigned 32bit integer=w1476:u32)
                                n756 = Wait (ms)(milliseconds to wait=w1476) -> ()  [unwired: 1 out]
                                }
                                frame True {
                                n757 = local read "Delay (s)"() -> (w1480:dbl)
                                n758 = Multiply(x=w1480, y=1000.0) -> (x*y=w1478:dbl)
                                n759 = To Unsigned Long Integer(number=w1478) -> (unsigned 32bit integer=w1477:u32)
                                n760 = Wait (ms)(milliseconds to wait=w1477) -> ()  [unwired: 1 out]
                                }
                                }
                                }
                              }
                              n761 = Less Or Equal?(x=w1422, y=w1421) -> (x <= y?=w1417:bool)
                              n762 = Bundle By Name(cluster=w1412, "Spec Plot"=w1413) -> (w1411:T6)
                              n763 = Not(x="Abort Scan") -> (.not. x?=w1416:bool)
                              n764 = Unbundle By Name(w1419) -> ("status"=w1415:bool)
                              n765 = Compound Arithmetic op=AND(invert w1415, w1416, w1417) -> (w1414:bool)
                            }
                          }
                        }
                      }
                    }
                    n766 = Unbundle By Name(w1286) -> ("Spec Plot.Wavelength"=w1283:dbl[], "Spec Plot.Int WF"=w1282:dbl[])
                    n767 = Bundle("Wavelength"=w1283, "Int WF"=w1282) -> (w1281:cluster{"Wavelength":dbl[], "Int WF":dbl[]})  [unwired: 1 in]
                    n768 = local write "XY Graph"(w1281) -> ()
                  }
                }
              }
              frame #2 {
                n769 = while {
                  stop <- w1481 continue-if-true
                  n770 = shared-variable ".\\Shared Variables.lvlib\\iHR550_GL302_scan"() -> (w1481:bool)  [unwired: 1 in, 1 out]
                  n771 = case shown="False" w1481 {
                    frame False {
                      n772 = local write "Scan"(FALSE ("Scan")) -> ()
                    }
                    frame True {
                      n773 = local write "Scan"(TRUE ("Scan")) -> ()
                    }
                  }
                }
              }
            }
            n774 = Unbundle By Name(w1118) -> ("status"=w1117:bool)
            n775 = case shown="False" w1117 {
              tunnel: [w1124 Control_3."Error Handler"] -> w1120
              frame False {
                n776 = local read "Log Data"() -> (w1125:bool)
                n777 = case shown="False" w1125 {
                  tunnel: [Control_3."Idle" Control_3."Log Data"] -> w1124
                  frame False {
                  }
                  frame True {
                  }
                }
              }
              frame True {
              }
            }
          }
          frame "Log Data" {
            n778 = stacked-sequence {
              seq-local: [w1494 _] -> [_ w1525]
              tunnel: w1489 -> [w1494 _]
              tunnel: [_ w1524] -> w1488
              tunnel: w1487 -> [w1493 _]
              tunnel: [w1492 _] -> w1485
              frame #0 {
                n779 = case shown="\"CSV\"" "File Format" {
                  tunnel: w1494 -> [w1499 w1519]
                  tunnel: w1493 -> [w1497 w1516]
                  tunnel: [w1496 w1516] -> w1492
                  frame "XML" {
                    n780 = Unbundle By Name(w1499) -> ("Spec Plot"=w1498:cluster{"Wavelength":dbl[], "Int WF":dbl[]})
                    n781 = local read "Interval Wavelength"() -> (w1506:dbl)
                    n782 = local read "Start Wavelength"() -> (w1508:dbl)
                    n783 = local read "End Wavelength"() -> (w1507:dbl)
                    n784 = Get Date/Time In Seconds() -> (seconds since 1Jan1904=w1513:timestamp)
                    n785 = local read "Delay (s)"() -> (w1505:dbl)
                    n786 = Get Date/Time String(seconds (now)=w1513) -> (date string=w1511:string, time string=w1510:string)  [unwired: 2 in]
                    n787 = Bundle By Name(cluster=T5 {"Operator's Name"="", "Start Wavelength"=0.0, "End Wavelength"=0.0, "Interval Wavelength"=0.0, "Delay"=0.0, "Date"="", "Time"="", "Data"={"Wavelength"=[], "Int WF"=[]}}, "Time"=w1510, "Date"=w1511, "Operator's Name"="Operator's Name", "Start Wavelength"=w1508, "End Wavelength"=w1507, "Interval Wavelength"=w1506, "Delay"=w1505, "Data"=w1498) -> (w1504:T5)
                    n788 = local read "Path"() -> (w1500:path)
                    n789 = To Variant(anything=w1504) -> (Variant=w1503:variant)
                    n790 = call <vilib>:"gxml_Generator.vi"("error in"=w1497, "Variant"=w1503) -> ("error out"=w1502:errorcluster, "XML String Out"=w1501:string)  [unwired: 8 in]
                    n791 = call <vilib>:"gxml_WriteXMLtoFile.vi"("error in"=w1502, "XML Input"=w1501, "XML File Path"=w1500) -> ("error out"=w1496:errorcluster)  [unwired: 7 in, 1 out]
                  }
                  frame "CSV" {
                    n792 = Unbundle By Name(w1519) -> ("Spec Plot.Wavelength"=w1518:dbl[], "Spec Plot.Int WF"=w1517:dbl[])
                    n793 = Build Array(w1518, w1517) -> (w1520:dbl[][])
                    n794 = call-poly <vilib>:"Write To Spreadsheet File.vi"("delimiter (\\t)"="," ("delimiter (\\t)"), "transpose? (no:F)"=TRUE, "format (%.3f)"="%.13f", "2D data"=w1520, "file path (dialog if empty)"="Path") -> ()  [unwired: 3 in, 1 out]
                  }
                }
              }
              frame #1 {
                n795 = case shown="True" "Clear data array" {
                  tunnel: w1525 -> [w1526 w1528]
                  tunnel: [w1526 w1527] -> w1524
                  frame False {
                  }
                  frame True {
                    n796 = Bundle By Name(cluster=w1528, "Spec Plot"=cluster{"Wavelength":dbl[], "Int WF":dbl[]} {"Wavelength"=[], "Int WF"=[]}) -> (w1527:T6)
                  }
                }
              }
            }
            n797 = Unbundle By Name(w1485) -> ("status"=w1484:bool)
            n798 = case shown="False" w1484 {
              tunnel: [Control_3."Idle" Control_3."Error Handler"] -> w1486
              frame False {
              }
              frame True {
              }
            }
          }
          frame "Error Handler" {
            n799 = call <vilib>:"Simple Error Handler.vi"("error in (no error)"=w1533) -> ("code out"=w1535:i32, "source out"=→"source out 2":string, "error out"=w1536:errorcluster)  [unwired: 4 in, 2 out]
            "code out" <- w1535
            n800 = call <vilib>:"Clear Errors.vi"("error in (no error)"=w1536, "specific error code to clear (0: all)"=w1535) -> ("error out"=w1531:errorcluster)  [unwired: 4 in, 1 out]
            n801 = Unbundle By Name(w1531) -> ("status"=w1530:bool)
            n802 = case shown="True" w1530 {
              tunnel: [Control_3."Idle" Control_3."Error Handler"] -> w1532
              frame False {
              }
              frame True {
              }
            }
          }
          frame "GL302 Goto WL" {
            n803 = stacked-sequence {
              tunnel: w1545 -> [_ w1551 _]
              tunnel: [_ w1549 _] -> w1543
              tunnel: w1540 -> [_ w1550 _]
              frame #0 {
                n804 = local read "Present Wavelength"() -> (w1548:dbl)
                n805 = Add(x=0.1, y=w1548) -> (x+y=w1546:dbl)
                n806 = shared-variable ".\\Shared Variables.lvlib\\next_WL"(w1546) -> ()  [unwired: 1 in, 1 out]
              }
              frame #1 {
                n807 = while {
                  tunnel: w1550 -> [w1575]
                  shift-right: [w1552] -> w1549
                  shift-left: w1551 -> [w1584]
                  stop <- w1558 stop-if-true
                  w1585 = TRUE
                  n808 = local read "Grating, gr/mm"() -> (w1580:u16)
                  n809 = local read "Calibration, nm"() -> (w1581:dbl)
                  n810 = Wait (ms)(milliseconds to wait=u32 10) -> ()  [unwired: 1 out]
                  n811 = shared-variable ".\\Shared Variables.lvlib\\next_WL"() -> (w1557:dbl)  [unwired: 1 in, 1 out]
                  n812 = local read "Destination Wavelength"() -> (w1572:dbl)
                  n813 = local read "Present Wavelength"() -> (w1579:dbl)
                  n814 = call "wavelength_string.vi"("error in (no error)"=w1584, "Grating, gr/mm"=w1580, "Destination Wavelength"=w1557, "Calibration, nm"=w1581) -> ("error out"=w1583:errorcluster, "Wavelength_String"=w1586:string)  [unwired: 1 in]
                  n815 = call "RS232.vi"("read"=FALSE, "milliseconds to wait"=u32 50, "error in"=w1583, "write"=w1585, "string to write"=w1586, "VISA  name in"=w1575) -> ("error out"=w1577:errorcluster, "VISA out"=w1582:refnum<visa-resource-name>)  [unwired: 2 out]
                  n816 = Less?(x=w1572, y=w1579) -> (x < y?=w1578:bool)
                  n817 = case shown="True" w1578 {
                    tunnel: w1577 -> [w1587 w1589]
                    tunnel: [w1587 w1588] -> w1576
                    frame False {
                    }
                    frame True {
                      n818 = local read "Backlash Compensation"() -> (w1590:bool)
                      n819 = case shown="True" w1590 {
                        tunnel: w1589 -> [w1591 w1592]
                        tunnel: [w1591 w1592] -> w1588
                        frame False {
                        }
                        frame True {
                          n820 = local read "Backlash Compensation"() -> (w1594:dbl)
                          n821 = local read "Grating, gr/mm"() -> (w1593:u16)
                          n822 = call "backlash_move.vi"("Grating, gr/mm"=w1593, "Wavelength, nm"=w1594) -> ()  [unwired: 3 in]
                        }
                      }
                    }
                  }
                  n823 = local read "delay before read (ms)"() -> (w1568:u32)
                  n824 = call "RS232.vi"("read"=w1585, "milliseconds to wait"=w1568, "error in"=w1576, "write"=w1585, "string to write"="X-1?", "VISA  name in"=w1582) -> ("error out"=w1571:errorcluster, "bytes to read"=w1567:u32, "read string"=w1569:string)  [unwired: 1 out]
                  n825 = call "GL302 Status.vi"("bytes to read"=w1567) -> ("Numeric"=w1565:u32, "String"=w1566:string)  [unwired: 9 in]
                  n826 = call "string_wavelength.vi"("Calibration, nm"=w1581, "Position String"=w1569, "Grating, gr/mm"=w1580, "error in (no error)"=w1571) -> ("Present Wavelength"=w1556:dbl, "error out"=w1553:errorcluster)  [unwired: 1 in]
                  n827 = local write "Status"(w1566) -> ()
                  n828 = local write "Present Wavelength"(w1556) -> ()
                  n829 = Subtract(x=w1572, y=w1556) -> (x-y=w1562:dbl)
                  n830 = Add(x=w1556, y=0.1) -> (x+y=w1555:dbl)
                  n831 = Absolute Value(x=w1562) -> (abs(x)=w1561:dbl)
                  n832 = property on="Status" class="Str"("Text.BGColor"=w1565) -> ()  [unwired: 2 in, 2 out]
                  n833 = shared-variable ".\\Shared Variables.lvlib\\next_WL"(w1555, error in=w1553) -> (error out=w1552:errorcluster)
                  n834 = Less?(x=w1561, y=0.06) -> (x < y?=w1559:bool)
                  n835 = Or(x=w1559, y="stop") -> (x .or. y?=w1558:bool)
                }
              }
              frame #2 {
                n836 = local write "Target Wavelength"(FALSE ("Target Wavelength")) -> ()
              }
            }
            n837 = Unbundle By Name(w1543) -> ("status"=w1542:bool)
            n838 = case shown="False" w1542 {
              tunnel: [Control_3."Idle" Control_3."Error Handler"] -> w1541
              frame False {
              }
              frame True {
              }
            }
          }
          frame "GL302 scan" {
            n839 = stacked-sequence {
              seq-local: [w1606 _ _] -> [_ w1612 _]
              tunnel: w1605 -> [w1608 _ _]
              tunnel: w1604 -> [_ w1614 _]
              tunnel: w1603 -> [_ w1613 _]
              tunnel: [_ w1611 _] -> w1601
              tunnel: [_ w1610 _] -> w1600
              tunnel: w1599 -> [_ w1609 _]
              frame #0 {
                n840 = Bundle By Name(cluster=w1608, "Spec Plot"=cluster{"Wavelength":dbl[], "Int WF":dbl[]} {"Wavelength"=[], "Int WF"=[]}) -> (w1606:T6)
              }
              frame #1 {
                n841 = case shown="\"Uninterrupted\"" "Scan Mode" {
                  tunnel: w1614 -> [w1624 w1805]
                  tunnel: w1613 -> [w1623 w1804]
                  tunnel: w1612 -> [w1622 w1803]
                  tunnel: [w1621 w1802] -> w1611
                  tunnel: [w1617 w1801] -> w1610
                  tunnel: w1609 -> [w1616 w1794]
                  frame "Interrupted " {
                    n842 = stacked-sequence {
                      seq-local: [w1626 _] -> [_ w1653]
                      seq-local: [w1632 _] -> [_ w1654]
                      tunnel: w1624 -> [w1633 _]
                      tunnel: [_ w1652] -> w1621
                      tunnel: w1623 -> [_ w1651]
                      tunnel: w1622 -> [_ w1650]
                      tunnel: [_ w1649] -> w1617
                      tunnel: w1616 -> [w1631 _]
                      frame #0 {
                        w1643 = TRUE
                        n843 = local read "Start Wavelength"() -> (w1636:dbl)
                        n844 = local read "Grating, gr/mm"() -> (w1645:u16)
                        n845 = local read "Calibration, nm"() -> (w1646:dbl)
                        n846 = local read "delay before read (ms)"() -> (w1644:u32)
                        n847 = call "wavelength_string.vi"("error in (no error)"=w1633, "Grating, gr/mm"=w1645, "Destination Wavelength"=w1636, "Calibration, nm"=w1646) -> ("error out"=w1642:errorcluster, "Wavelength_String"=w1637:string)  [unwired: 1 in]
                        n848 = call "RS232.vi"("read"=w1643, "milliseconds to wait"=w1644, "error in"=w1642, "write"=w1643, "string to write"=w1637, "VISA  name in"=w1631) -> ("error out"=w1641:errorcluster, "VISA out"=w1638:refnum<visa-resource-name>)  [unwired: 2 out]
                        n849 = call "RS232.vi"("read"=w1643, "milliseconds to wait"=w1644, "error in"=w1641, "write"=w1643, "string to write"="X-1?", "VISA  name in"=w1638) -> ("error out"=w1640:errorcluster, "bytes to read"=w1630:u32, "read string"=w1639:string, "VISA out"=w1632:refnum<visa-resource-name>)
                        n850 = call "GL302 Status.vi"("bytes to read"=w1630) -> ("Numeric"=w1628:u32, "String"=w1629:string)  [unwired: 9 in]
                        n851 = call "string_wavelength.vi"("Calibration, nm"=w1646, "Position String"=w1639, "Grating, gr/mm"=w1645, "error in (no error)"=w1640) -> ("Present Wavelength"=w1647:dbl, "error out"=w1635:errorcluster)  [unwired: 1 in]
                        n852 = local write "Status"(w1629) -> ()
                        n853 = property on="Status" class="Str"("Text.BGColor"=w1628) -> ()  [unwired: 2 in, 2 out]
                        n854 = local write "Present Wavelength"(w1647) -> ()
                        n855 = shared-variable ".\\Shared Variables.lvlib\\mono tick"(u32 1 ("mono tick"), error in=w1635) -> (error out=w1627:errorcluster)
                        n856 = shared-variable ".\\Shared Variables.lvlib\\osc tick"(u32 0 ("osc tick"), error in=w1627) -> (error out=w1626:errorcluster)
                      }
                      frame #1 {
                        n857 = while {
                          tunnel: w1654 -> [w1673]
                          tunnel: w1653 -> [w1672]
                          tunnel: [w1667] -> w1652
                          tunnel: w1651 -> [w1662]
                          shift-right: [w1660] -> w1649
                          shift-left: w1650 -> [w1661]
                          stop <- w1663 continue-if-true
                          n858 = local read "Present Wavelength"() -> (w1659:dbl)
                          n859 = local read "Start Wavelength"() -> (w1670:dbl)
                          n860 = local read "End Wavelength"() -> (w1671:dbl)
                          n861 = Build Array("FW", "BW") -> (w1675:bool[])
                          n862 = Greater Or Equal?(x=w1671, y=w1659) -> (x >= y?=w1668:bool)
                          n863 = Less Or Equal?(x=w1670, y=w1659) -> (x <= y?=w1669:bool)
                          n864 = Search 1D Array(1D array=w1675, element=TRUE) -> (index of element=w1658:i32)  [unwired: 1 in]
                          n865 = And(x=w1668, y=w1669) -> (x .and. y?=w1666:bool)
                          n866 = Increment(x=w1658) -> (x+1=w1657:i32)
                          n867 = case shown="1" w1657 {
                            tunnel: w1673 -> [_ w1690 w1750]
                            tunnel: w1672 -> [w1678 w1689 w1747]
                            tunnel: [w1678 w1688 w1746] -> w1667
                            tunnel: w1662 -> [_ w1684 _]
                            tunnel: w1661 -> [w1679 w1683 w1749]
                            tunnel: [w1679 w1682 w1748] -> w1660
                            tunnel: w1659 -> [_ w1681 w1751]
                            frame 0, Default {
                            }
                            frame 1 {
                              n868 = shared-variable ".\\Shared Variables.lvlib\\C8855_init"() -> (w1680:bool)  [unwired: 1 in, 1 out]
                              n869 = shared-variable ".\\Shared Variables.lvlib\\mono tick"() -> (w1687:u32)  [unwired: 1 in, 1 out]
                              n870 = shared-variable ".\\Shared Variables.lvlib\\osc tick"() -> (w1686:u32)  [unwired: 1 in, 1 out]
                              n871 = Less?(x=w1687, y=w1686) -> (x < y?=w1685:bool)
                              n872 = case shown="True" w1685 {
                                tunnel: w1690 -> [_ w1700]
                                tunnel: w1689 -> [w1691 w1696]
                                tunnel: [w1691 w1695] -> w1688
                                tunnel: w1684 -> [_ w1699]
                                tunnel: w1683 -> [w1692 w1698]
                                tunnel: [w1692 w1697] -> w1682
                                tunnel: w1681 -> [_ w1694]
                                tunnel: w1680 -> [_ w1693]
                                frame False {
                                }
                                frame True {
                                n873 = stacked-sequence {
                                tunnel: w1700 -> [w1734 _]
                                tunnel: w1699 -> [w1703 _]
                                tunnel: w1698 -> [w1717 _]
                                tunnel: [w1716 _] -> w1697
                                tunnel: w1696 -> [w1702 _]
                                tunnel: [w1712 _] -> w1695
                                tunnel: w1694 -> [w1711 _]
                                tunnel: w1693 -> [w1704 _]
                                frame #0 {
                                w1728 = TRUE
                                n874 = case shown="True" w1704 {
                                tunnel: w1703 -> [w1737 _]
                                tunnel: w1702 -> [w1736 w1739]
                                tunnel: [w1735 w1739] -> w1701
                                frame False {
                                n875 = Enqueue Element(queue=w1737, element=Control_4."Waveform Queries" ("Enum"), error in (no error)=w1736) -> (error out=w1735:errorcluster)  [unwired: 1 in, 2 out]
                                }
                                frame True {
                                }
                                }
                                n876 = local read "Step"() -> (w1725:dbl)
                                n877 = Unbundle By Name(w1717) -> ("Spec Plot.Wavelength"=w1719:dbl[], "Spec Plot.Int WF"=w1718:dbl[])
                                n878 = local read "Calibration, nm"() -> (w1723:dbl)
                                n879 = local read "Grating, gr/mm"() -> (w1722:u16)
                                n880 = Add(x=w1711, y=w1725) -> (x+y=w1724:dbl)
                                n881 = shared-variable ".\\Shared Variables.lvlib\\Area"(error in=w1701) -> (w1715:dbl, error out=w1714:errorcluster)
                                n882 = local read "delay before read (ms)"() -> (w1731:u32)
                                n883 = Build Array (concatenate)(w1719, w1711) -> (w1707:dbl[])
                                n884 = Build Array (concatenate)(w1718, w1715) -> (w1706:dbl[])
                                n885 = call "wavelength_string.vi"("error in (no error)"=w1714, "Grating, gr/mm"=w1722, "Destination Wavelength"=w1724, "Calibration, nm"=w1723) -> ("error out"=w1721:errorcluster, "Wavelength_String"=w1720:string)  [unwired: 1 in]
                                n886 = Bundle By Name(cluster=w1717, "Spec Plot.Wavelength"=w1707, "Spec Plot.Int WF"=w1706) -> (w1716:T6)
                                n887 = call "RS232.vi"("read"=w1728, "milliseconds to wait"=w1731, "error in"=w1721, "write"=w1728, "string to write"=w1720, "VISA  name in"=w1734) -> ("error out"=w1727:errorcluster, "VISA out"=w1733:refnum<visa-resource-name>)  [unwired: 2 out]
                                n888 = call "RS232.vi"("read"=w1728, "milliseconds to wait"=w1731, "error in"=w1727, "write"=w1728, "string to write"="X-1?", "VISA  name in"=w1733) -> ("error out"=w1726:errorcluster, "bytes to read"=w1708:u32, "read string"=w1729:string)  [unwired: 1 out]
                                n889 = call "string_wavelength.vi"("Calibration, nm"=w1723, "Position String"=w1729, "Grating, gr/mm"=w1722, "error in (no error)"=w1726) -> ("Present Wavelength"=w1730:dbl, "error out"=w1713:errorcluster)  [unwired: 1 in]
                                n890 = flat-sequence {
                                tunnel: w1713 -> [w1744]
                                tunnel: [w1741] -> w1712
                                frame #0 {
                                n891 = Tick Count (ms)() -> (millisecond timer value=w1743:u32)
                                n892 = shared-variable ".\\Shared Variables.lvlib\\mono tick"(w1743, error in=w1744) -> (error out=w1742:errorcluster)
                                n893 = shared-variable ".\\Shared Variables.lvlib\\Gate Open"(TRUE ("Gate Open"), error in=w1742) -> (error out=w1741:errorcluster)
                                }
                                }
                                n894 = call "GL302 Status.vi"("bytes to read"=w1708) -> ("Numeric"=w1709:u32, "String"=w1710:string)  [unwired: 9 in]
                                n895 = local write "Present Wavelength"(w1730) -> ()
                                n896 = local write "Status"(w1710) -> ()
                                n897 = property on="Status" class="Str"("Text.BGColor"=w1709) -> ()  [unwired: 2 in, 2 out]
                                n898 = Bundle(w1707, w1706) -> (w1705:cluster{dbl[], dbl[]})  [unwired: 1 in]
                                n899 = local write "XY Graph"(w1705) -> ()
                                }
                                frame #1 {
                                w1745 = FALSE
                                n900 = local write "BW"(w1745) -> ()
                                n901 = local write "FW"(w1745) -> ()
                                }
                                }
                                }
                              }
                            }
                            frame 2 {
                              n902 = stacked-sequence {
                                tunnel: w1751 -> [w1774 _]
                                tunnel: w1750 -> [w1780 _]
                                tunnel: w1749 -> [w1773 _]
                                tunnel: [w1772 _] -> w1748
                                tunnel: w1747 -> [w1757 _]
                                tunnel: [w1756 _] -> w1746
                                frame #0 {
                                w1778 = TRUE
                                n903 = local read "Step"() -> (w1786:dbl)
                                n904 = Subtract(x=w1774, y=w1786) -> (x-y=w1785:dbl)
                                n905 = local read "Grating, gr/mm"() -> (w1775:u16)
                                n906 = local read "Calibration, nm"() -> (w1784:dbl)
                                n907 = local read "Backlash Compensation"() -> (w1771:bool)
                                n908 = local read "delay before read (ms)"() -> (w1788:u32)
                                n909 = call "wavelength_string.vi"("error in (no error)"=w1757, "Grating, gr/mm"=w1775, "Destination Wavelength"=w1785, "Calibration, nm"=w1784) -> ("error out"=w1777:errorcluster, "Wavelength_String"=w1779:string)  [unwired: 1 in]
                                n910 = call "RS232.vi"("read"=FALSE, "milliseconds to wait"=w1788, "error in"=w1777, "write"=w1778, "string to write"=w1779, "VISA  name in"=w1780) -> ("error out"=w1770:errorcluster, "VISA out"=w1781:refnum<visa-resource-name>)  [unwired: 2 out]
                                n911 = Unbundle By Name(w1773) -> ("Spec Plot.Wavelength"=w1761:dbl[], "Spec Plot.Int WF"=w1765:dbl[])
                                n912 = case shown="True" w1771 {
                                tunnel: [w1789 w1790] -> w1769
                                tunnel: w1770 -> [w1789 w1790]
                                frame False {
                                }
                                frame True {
                                n913 = local read "Grating, gr/mm"() -> (w1792:u16)
                                n914 = local read "Backlash Compensation"() -> (w1791:dbl)
                                n915 = call "backlash_move.vi"("Grating, gr/mm"=w1792, "Wavelength, nm"=w1791) -> ()  [unwired: 3 in]
                                }
                                }
                                n916 = Array Size(array=w1761) -> (size(s)=w1760:i32)
                                n917 = Array Size(array=w1765) -> (size(s)=w1764:i32)
                                n918 = Subtract(x=w1764, y=1) -> (x-y=w1762:i32)
                                n919 = Subtract(x=w1760, y=1) -> (x-y=w1758:i32)
                                n920 = Delete From Array(array=w1765, index=w1762) -> (array with subset deleted=w1754:dbl[])  [unwired: 1 in, 1 out]
                                n921 = Delete From Array(array=w1761, index=w1758) -> (array with subset deleted=w1755:dbl[])  [unwired: 1 in, 1 out]
                                n922 = Bundle By Name(cluster=w1773, "Spec Plot.Wavelength"=w1755, "Spec Plot.Int WF"=w1754) -> (w1772:T6)
                                n923 = call "RS232.vi"("read"=w1778, "milliseconds to wait"=w1788, "error in"=w1769, "write"=w1778, "string to write"="X-1?", "VISA  name in"=w1781) -> ("error out"=w1776:errorcluster, "bytes to read"=w1768:u32, "read string"=w1783:string)  [unwired: 1 out]
                                n924 = call "string_wavelength.vi"("Calibration, nm"=w1784, "Position String"=w1783, "Grating, gr/mm"=w1775, "error in (no error)"=w1776) -> ("Present Wavelength"=w1787:dbl, "error out"=w1756:errorcluster)  [unwired: 1 in]
                                n925 = call "GL302 Status.vi"("bytes to read"=w1768) -> ("Numeric"=w1766:u32, "String"=w1767:string)  [unwired: 9 in]
                                n926 = local write "Present Wavelength"(w1787) -> ()
                                n927 = local write "Status"(w1767) -> ()
                                n928 = property on="Status" class="Str"("Text.BGColor"=w1766) -> ()  [unwired: 2 in, 2 out]
                                n929 = Bundle("Wavelength"=w1755, "Int WF"=w1754) -> (w1753:cluster{"Wavelength":dbl[], "Int WF":dbl[]})  [unwired: 1 in]
                                n930 = local write "XY Graph"(w1753) -> ()
                                }
                                frame #1 {
                                w1793 = FALSE
                                n931 = local write "BW"(w1793) -> ()
                                n932 = local write "FW"(w1793) -> ()
                                }
                              }
                            }
                          }
                          n933 = local read "Abort Scan GL302"() -> (w1665:bool)
                          n934 = Not(x=w1665) -> (.not. x?=w1664:bool)
                          n935 = Unbundle By Name(w1667) -> ("status"=w1656:bool)
                          n936 = Not(x=w1656) -> (.not. x?=w1655:bool)
                          n937 = Compound Arithmetic op=AND(w1655, w1664, w1666) -> (w1663:bool)
                        }
                      }
                    }
                    n938 = Unbundle By Name(w1617) -> ("Spec Plot.Wavelength"=w1620:dbl[], "Spec Plot.Int WF"=w1619:dbl[])
                    n939 = Bundle("Wavelength"=w1620, "Int WF"=w1619) -> (w1618:cluster{"Wavelength":dbl[], "Int WF":dbl[]})  [unwired: 1 in]
                    n940 = local write "XY Graph"(w1618) -> ()
                  }
                  frame "Uninterrupted" {
                    n941 = Less?(x="Start Wavelength", y="End Wavelength") -> (x < y?=w1798:bool)
                    n942 = case shown="True" w1798 {
                      tunnel: w1805 -> [w1811 w1946]
                      tunnel: w1804 -> [w1809 w1945]
                      tunnel: w1803 -> [w1810 w1944]
                      tunnel: [w1808 w1943] -> w1802
                      tunnel: [w1807 w1942] -> w1801
                      tunnel: w1794 -> [w1806 w1941]
                      frame False {
                        n943 = stacked-sequence {
                          seq-local: [w1828 _] -> [_ w1848]
                          seq-local: [w1816 _] -> [_ w1849]
                          tunnel: w1811 -> [w1835 _]
                          tunnel: w1810 -> [_ w1851]
                          tunnel: w1809 -> [_ w1850]
                          tunnel: [_ w1847] -> w1808
                          tunnel: [_ w1846] -> w1807
                          tunnel: w1806 -> [w1831 _]
                          frame #0 {
                            w1826 = TRUE ("write")
                            n944 = local read "Present Wavelength"() -> (w1812:dbl)
                            n945 = local read "Start Wavelength"() -> (w1813:dbl)
                            n946 = local read "Grating, gr/mm"() -> (w1819:u16)
                            n947 = local read "Calibration, nm"() -> (w1820:dbl)
                            n948 = Less?(x=w1812, y=w1813) -> (x < y?=w1814:bool)
                            n949 = call "wavelength_string.vi"("error in (no error)"=w1835, "Grating, gr/mm"=w1819, "Destination Wavelength"=w1813, "Calibration, nm"=w1820) -> ("error out"=w1834:errorcluster, "Wavelength_String"=w1837:string)  [unwired: 1 in]
                            n950 = local read "delay before read (ms)"() -> (w1818:u32)
                            n951 = call "RS232.vi"("read"=FALSE, "milliseconds to wait"=w1818, "error in"=w1834, "write"=TRUE, "string to write"=w1837, "VISA  name in"=w1831) -> ("error out"=w1832:errorcluster, "VISA out"=w1829:refnum<visa-resource-name>)  [unwired: 2 out]
                            n952 = case shown="False" w1814 {
                              tunnel: w1832 -> [w1838 w1841]
                              tunnel: [w1838 w1840] -> w1825
                              frame False {
                              }
                              frame True {
                                n953 = case shown="True" "Backlash Compensation" {
                                tunnel: [w1842 w1843] -> w1840
                                tunnel: w1841 -> [w1842 w1843]
                                frame False {
                                }
                                frame True {
                                n954 = local read "Backlash Compensation"() -> (w1845:dbl)
                                n955 = local read "Grating, gr/mm"() -> (w1844:u16)
                                n956 = call "backlash_move.vi"("Grating, gr/mm"=w1844, "Wavelength, nm"=w1845) -> ()  [unwired: 3 in]
                                }
                                }
                              }
                            }
                            n957 = call "RS232.vi"("read"=w1826, "milliseconds to wait"=w1818, "error in"=w1825, "write"=w1826, "string to write"="X-1?", "VISA  name in"=w1829) -> ("error out"=w1824:errorcluster, "read string"=w1821:string, "VISA out"=w1828:refnum<visa-resource-name>)  [unwired: 1 out]
                            n958 = call "string_wavelength.vi"("Calibration, nm"=w1820, "Position String"=w1821, "Grating, gr/mm"=w1819, "error in (no error)"=w1824) -> ("Present Wavelength"=w1822:dbl, "error out"=w1823:errorcluster)  [unwired: 1 in]
                            n959 = local write "Present Wavelength"(w1822) -> ()
                            n960 = shared-variable ".\\Shared Variables.lvlib\\mono tick"(u32 1 ("mono tick"), error in=w1823) -> (error out=w1817:errorcluster)
                            n961 = shared-variable ".\\Shared Variables.lvlib\\osc tick"(u32 0 ("osc tick"), error in=w1817) -> (error out=w1816:errorcluster)
                          }
                          frame #1 {
                            n962 = while {
                              shift-right: [w1852] -> w1846
                              shift-left: w1851 -> [w1853]
                              tunnel: w1850 -> [w1860]
                              tunnel: w1849 -> [w1859]
                              tunnel: w1848 -> [w1857]
                              tunnel: [w1855] -> w1847
                              stop <- w1861 continue-if-true
                              n963 = local read "Present Wavelength"() -> (w1858:dbl)
                              n964 = stacked-sequence {
                                seq-local: [w1866 _ _] -> [_ w1930 _]
                                seq-local: [_ w1927 _] -> [_ _ w1932]
                                tunnel: w1853 -> [w1873 _ _]
                                tunnel: w1860 -> [w1872 _ _]
                                tunnel: w1859 -> [w1871 _ _]
                                tunnel: w1858 -> [w1870 _ _]
                                tunnel: w1857 -> [w1869 _ _]
                                tunnel: [w1868 _ _] -> w1856
                                tunnel: [w1867 _ _] -> w1855
                                tunnel: [_ _ w1932] -> w1854
                                frame #0 {
                                n965 = shared-variable ".\\Shared Variables.lvlib\\mono tick"() -> (w1876:u32)  [unwired: 1 in, 1 out]
                                n966 = shared-variable ".\\Shared Variables.lvlib\\osc tick"() -> (w1875:u32)  [unwired: 1 in, 1 out]
                                n967 = Less?(x=w1876, y=w1875) -> (x < y?=w1874:bool)
                                n968 = case shown="True" w1874 {
                                tunnel: w1873 -> [w1877 w1910]
                                tunnel: w1872 -> [_ w1880]
                                tunnel: w1871 -> [w1878 w1882]
                                tunnel: [w1877 w1907] -> w1866
                                tunnel: w1870 -> [_ w1905]
                                tunnel: w1869 -> [_ w1902]
                                tunnel: [w1878 w1883] -> w1867
                                frame False {
                                }
                                frame True {
                                w1889 = TRUE ("write")
                                n969 = shared-variable ".\\Shared Variables.lvlib\\C8855_init"() -> (w1879:bool)  [unwired: 1 in, 1 out]
                                n970 = case shown="False" w1879 {
                                tunnel: w1882 -> [w1915 w1917]
                                tunnel: [w1914 w1917] -> w1881
                                tunnel: w1880 -> [w1913 _]
                                frame False {
                                n971 = Enqueue Element(queue=w1913, element=Control_4."Waveform Queries" ("Enum"), error in (no error)=w1915) -> (error out=w1914:errorcluster)  [unwired: 1 in, 2 out]
                                }
                                frame True {
                                }
                                }
                                n972 = local read "Step"() -> (w1904:dbl)
                                n973 = Unbundle By Name(w1910) -> ("Spec Plot.Wavelength"=w1912:dbl[], "Spec Plot.Int WF"=w1911:dbl[])
                                n974 = Subtract(x=w1905, y=w1904) -> (x-y=w1903:dbl)
                                n975 = local read "Grating, gr/mm"() -> (w1890:u16)
                                n976 = local read "Calibration, nm"() -> (w1891:dbl)
                                n977 = shared-variable ".\\Shared Variables.lvlib\\Area"(error in=w1881) -> (w1906:dbl, error out=w1901:errorcluster)
                                n978 = local read "Backlash Compensation"() -> (w1897:bool)
                                n979 = Build Array (concatenate)(w1912, w1905) -> (w1909:dbl[])
                                n980 = Build Array (concatenate)(w1911, w1906) -> (w1908:dbl[])
                                n981 = call "wavelength_string.vi"("error in (no error)"=w1901, "Grating, gr/mm"=w1890, "Destination Wavelength"=w1903, "Calibration, nm"=w1891) -> ("error out"=w1900:errorcluster, "Wavelength_String"=w1898:string)  [unwired: 1 in]
                                n982 = Bundle By Name(cluster=w1910, "Spec Plot.Wavelength"=w1909, "Spec Plot.Int WF"=w1908) -> (w1907:T6)
                                n983 = local read "delay before read (ms)"() -> (w1884:u32)
                                n984 = call "RS232.vi"("read"=FALSE, "milliseconds to wait"=w1884, "error in"=w1900, "write"=TRUE, "string to write"=w1898, "VISA  name in"=w1902) -> ("error out"=w1896:errorcluster, "VISA out"=w1893:refnum<visa-resource-name>)  [unwired: 2 out]
                                n985 = case shown="True" w1897 {
                                tunnel: w1896 -> [w1923 w1924]
                                tunnel: [w1923 w1924] -> w1888
                                frame False {
                                }
                                frame True {
                                n986 = local read "Backlash Compensation"() -> (w1925:dbl)
                                n987 = local read "Grating, gr/mm"() -> (w1926:u16)
                                n988 = call "backlash_move.vi"("Grating, gr/mm"=w1926, "Wavelength, nm"=w1925) -> ()  [unwired: 3 in]
                                }
                                }
                                n989 = call "RS232.vi"("read"=w1889, "milliseconds to wait"=w1884, "error in"=w1888, "write"=w1889, "string to write"="X-1?", "VISA  name in"=w1893) -> ("error out"=w1887:errorcluster, "read string"=w1892:string)  [unwired: 2 out]
                                n990 = call "string_wavelength.vi"("Calibration, nm"=w1891, "Position String"=w1892, "Grating, gr/mm"=w1890, "error in (no error)"=w1887) -> ("Present Wavelength"=w1885:dbl, "error out"=w1886:errorcluster)  [unwired: 1 in]
                                n991 = local write "Present Wavelength"(w1885) -> ()
                                n992 = flat-sequence {
                                tunnel: w1886 -> [w1922]
                                tunnel: [w1919] -> w1883
                                frame #0 {
                                n993 = Tick Count (ms)() -> (millisecond timer value=w1921:u32)
                                n994 = shared-variable ".\\Shared Variables.lvlib\\mono tick"(w1921, error in=w1922) -> (error out=w1920:errorcluster)
                                n995 = shared-variable ".\\Shared Variables.lvlib\\Gate Open"(TRUE ("Gate Open"), error in=w1920) -> (error out=w1919:errorcluster)
                                }
                                }
                                }
                                }
                                n996 = Unbundle By Name(w1867) -> ("status"=w1868:bool)
                                }
                                frame #1 {
                                n997 = Unbundle By Name(w1930) -> ("Spec Plot.Wavelength"=w1929:dbl[], "Spec Plot.Int WF"=w1928:dbl[])
                                n998 = Bundle("Wavelength"=w1929, "Int WF"=w1928) -> (w1927:cluster{"Wavelength":dbl[], "Int WF":dbl[]})  [unwired: 1 in]
                                n999 = local write "XY Graph"(w1927) -> ()
                                }
                                frame #2 {
                                n1000 = shared-variable ".\\Shared Variables.lvlib\\C8855_init"() -> (w1931:bool)  [unwired: 1 in, 1 out]
                                n1001 = case shown="True" w1931 {
                                frame False {
                                n1002 = local read "Pause"() -> (w1936:dbl)
                                n1003 = Multiply(x=w1936, y=1000.0) -> (x*y=w1934:dbl)
                                n1004 = To Unsigned Long Integer(number=w1934) -> (unsigned 32bit integer=w1933:u32)
                                n1005 = Wait (ms)(milliseconds to wait=w1933) -> ()  [unwired: 1 out]
                                }
                                frame True {
                                n1006 = local read "Pause"() -> (w1939:dbl)
                                n1007 = Multiply(x=1000.0 ("y"), y=w1939) -> (x*y=w1938:dbl)
                                n1008 = To Unsigned Long Integer(number=w1938) -> (unsigned 32bit integer=w1937:u32)
                                n1009 = Wait (ms)(milliseconds to wait=w1937) -> ()  [unwired: 1 out]
                                }
                                }
                                }
                              }
                              n1010 = local read "End Wavelength"() -> (w1863:dbl)
                              n1011 = Less Or Equal?(x=w1863, y=w1858) -> (x <= y?=w1862:bool)
                              n1012 = Bundle By Name(cluster=w1853, "Spec Plot"=w1854) -> (w1852:T6)
                              n1013 = local read "Abort Scan GL302"() -> (w1865:bool)
                              n1014 = Not(x=w1865) -> (.not. x?=w1864:bool)
                              n1015 = Compound Arithmetic op=AND(invert w1856, w1864, w1862) -> (w1861:bool)
                            }
                          }
                        }
                      }
                      frame True {
                        n1016 = stacked-sequence {
                          seq-local: [w1953 _] -> [_ w1985]
                          seq-local: [w1963 _] -> [_ w1983]
                          tunnel: w1946 -> [w1971 _]
                          tunnel: w1945 -> [_ w1986]
                          tunnel: w1944 -> [_ w1984]
                          tunnel: [_ w1982] -> w1943
                          tunnel: [_ w1981] -> w1942
                          tunnel: w1941 -> [w1968 _]
                          frame #0 {
                            w1956 = TRUE
                            n1017 = local read "Present Wavelength"() -> (w1949:dbl)
                            n1018 = local read "Start Wavelength"() -> (w1948:dbl)
                            n1019 = local read "Grating, gr/mm"() -> (w1960:u16)
                            n1020 = local read "delay before read (ms)"() -> (w1955:u32)
                            n1021 = Greater?(x=w1949, y=w1948) -> (0:w1947:bool)
                            n1022 = local read "Calibration, nm"() -> (w1961:dbl)
                            n1023 = call "wavelength_string.vi"("error in (no error)"=w1971, "Grating, gr/mm"=w1960, "Destination Wavelength"=w1948, "Calibration, nm"=w1961) -> ("error out"=w1972:errorcluster, "Wavelength_String"=w1967:string)  [unwired: 1 in]
                            n1024 = call "RS232.vi"("read"=FALSE, "milliseconds to wait"=w1955, "error in"=w1972, "write"=TRUE, "string to write"=w1967, "VISA  name in"=w1968) -> ("error out"=w1951:errorcluster, "VISA out"=w1965:refnum<visa-resource-name>)  [unwired: 2 out]
                            n1025 = case shown="False" w1947 {
                              tunnel: w1951 -> [w1973 w1975]
                              tunnel: [w1973 w1974] -> w1950
                              frame False {
                              }
                              frame True {
                                n1026 = local read "Backlash Compensation"() -> (w1976:bool)
                                n1027 = case shown="True" w1976 {
                                tunnel: w1975 -> [w1977 w1978]
                                tunnel: [w1977 w1978] -> w1974
                                frame False {
                                }
                                frame True {
                                n1028 = local read "Backlash Compensation"() -> (w1980:dbl)
                                n1029 = local read "Grating, gr/mm"() -> (w1979:u16)
                                n1030 = call "backlash_move.vi"("Grating, gr/mm"=w1979, "Wavelength, nm"=w1980) -> ()  [unwired: 3 in]
                                }
                                }
                              }
                            }
                            n1031 = call "RS232.vi"("read"=w1956, "milliseconds to wait"=w1955, "error in"=w1950, "write"=w1956, "string to write"="X-1?", "VISA  name in"=w1965) -> ("error out"=w1959:errorcluster, "read string"=w1958:string, "VISA out"=w1963:refnum<visa-resource-name>)  [unwired: 1 out]
                            n1032 = call "string_wavelength.vi"("Calibration, nm"=w1961, "Position String"=w1958, "Grating, gr/mm"=w1960, "error in (no error)"=w1959) -> ("Present Wavelength"=w1962:dbl, "error out"=w1964:errorcluster)  [unwired: 1 in]
                            n1033 = shared-variable ".\\Shared Variables.lvlib\\mono tick"(u32 1 ("mono tick"), error in=w1964) -> (error out=w1954:errorcluster)
                            n1034 = local write "Present Wavelength"(w1962) -> ()
                            n1035 = shared-variable ".\\Shared Variables.lvlib\\osc tick"(u32 0 ("osc tick"), error in=w1954) -> (error out=w1953:errorcluster)
                          }
                          frame #1 {
                            n1036 = while {
                              tunnel: w1986 -> [w2001]
                              tunnel: w1985 -> [w2000]
                              shift-right: [w1988] -> w1981
                              shift-left: w1984 -> [w1989]
                              tunnel: w1983 -> [w1999]
                              tunnel: [w1991] -> w1982
                              stop <- w1996 continue-if-true
                              n1037 = shared-variable ".\\Shared Variables.lvlib\\C8855_init"() -> (w1987:bool)  [unwired: 1 in, 1 out]
                              n1038 = local read "Present Wavelength"() -> (w1995:dbl)
                              n1039 = stacked-sequence {
                                seq-local: [_ w2065 _] -> [_ _ w2069]
                                seq-local: [w2003 _ _] -> [_ w2064 _]
                                tunnel: w2001 -> [w2010 _ _]
                                tunnel: w2000 -> [w2009 _ _]
                                tunnel: w1989 -> [w2008 _ _]
                                tunnel: w1999 -> [w2007 _ _]
                                tunnel: w1995 -> [w2006 _ _]
                                tunnel: [w2005 _ _] -> w1992
                                tunnel: [w2004 _ _] -> w1991
                                tunnel: [_ _ w2069] -> w1990
                                tunnel: w1987 -> [w2002 _ w2068]
                                frame #0 {
                                n1040 = shared-variable ".\\Shared Variables.lvlib\\mono tick"() -> (w2013:u32)  [unwired: 1 in, 1 out]
                                n1041 = shared-variable ".\\Shared Variables.lvlib\\osc tick"() -> (w2012:u32)  [unwired: 1 in, 1 out]
                                n1042 = Less?(x=w2013, y=w2012) -> (x < y?=w2011:bool)
                                n1043 = case shown="True" w2011 {
                                tunnel: w2010 -> [_ w2023]
                                tunnel: w2009 -> [w2014 w2022]
                                tunnel: w2008 -> [w2015 w2046]
                                tunnel: w2007 -> [_ w2043]
                                tunnel: [w2015 w2039] -> w2003
                                tunnel: [w2014 w2035] -> w2004
                                tunnel: w2006 -> [_ w2038]
                                tunnel: w2002 -> [_ w2020]
                                frame False {
                                }
                                frame True {
                                w2019 = TRUE
                                n1044 = case shown="True" w2020 {
                                tunnel: w2023 -> [w2056 _]
                                tunnel: w2022 -> [w2055 w2058]
                                tunnel: [w2054 w2058] -> w2021
                                frame False {
                                n1045 = Enqueue Element(queue=w2056, element=Control_4."Waveform Queries" ("Enum"), error in (no error)=w2055) -> (error out=w2054:errorcluster)  [unwired: 1 in, 2 out]
                                }
                                frame True {
                                }
                                }
                                n1046 = local read "Step"() -> (w2036:dbl)
                                n1047 = Unbundle By Name(w2046) -> ("Spec Plot.Wavelength"=w2049:dbl[], "Spec Plot.Int WF"=w2048:dbl[])
                                n1048 = local read "Grating, gr/mm"() -> (w2029:u16)
                                n1049 = local read "Calibration, nm"() -> (w2030:dbl)
                                n1050 = local read "Backlash Compensation"() -> (w2016:bool)
                                n1051 = shared-variable ".\\Shared Variables.lvlib\\Area"(error in=w2021) -> (w2047:dbl, error out=w2041:errorcluster)
                                n1052 = Add(x=w2036, y=w2038) -> (x+y=w2028:dbl)
                                n1053 = Build Array (concatenate)(w2049, w2038) -> (w2045:dbl[])
                                n1054 = Build Array (concatenate)(w2048, w2047) -> (w2044:dbl[])
                                n1055 = call "wavelength_string.vi"("error in (no error)"=w2041, "Grating, gr/mm"=w2029, "Destination Wavelength"=w2028, "Calibration, nm"=w2030) -> ("error out"=w2040:errorcluster, "Wavelength_String"=w2042:string)  [unwired: 1 in]
                                n1056 = local read "delay before read (ms)"() -> (w2024:u32)
                                n1057 = Bundle By Name(cluster=w2046, "Spec Plot.Wavelength"=w2045, "Spec Plot.Int WF"=w2044) -> (w2039:T6)
                                n1058 = call "RS232.vi"("read"=FALSE, "milliseconds to wait"=w2024, "error in"=w2040, "write"=TRUE, "string to write"=w2042, "VISA  name in"=w2043) -> ("error out"=w2018:errorcluster, "VISA out"=w2033:refnum<visa-resource-name>)  [unwired: 2 out]
                                n1059 = case shown="True" w2016 {
                                tunnel: w2018 -> [w2050 w2053]
                                tunnel: [w2050 w2053] -> w2017
                                frame False {
                                }
                                frame True {
                                n1060 = local read "Backlash Compensation"() -> (w2051:dbl)
                                n1061 = local read "Grating, gr/mm"() -> (w2052:u16)
                                n1062 = call "backlash_move.vi"("Grating, gr/mm"=w2052, "Wavelength, nm"=w2051) -> ()  [unwired: 3 in]
                                }
                                }
                                n1063 = call "RS232.vi"("read"=w2019, "milliseconds to wait"=w2024, "error in"=w2017, "write"=w2019, "string to write"="X-1?", "VISA  name in"=w2033) -> ("error out"=w2026:errorcluster, "read string"=w2027:string)  [unwired: 2 out]
                                n1064 = call "string_wavelength.vi"("Calibration, nm"=w2030, "Position String"=w2027, "Grating, gr/mm"=w2029, "error in (no error)"=w2026) -> ("Present Wavelength"=w2031:dbl, "error out"=w2032:errorcluster)  [unwired: 1 in]
                                n1065 = flat-sequence {
                                tunnel: w2032 -> [w2063]
                                tunnel: [w2060] -> w2035
                                frame #0 {
                                n1066 = Tick Count (ms)() -> (millisecond timer value=w2062:u32)
                                n1067 = shared-variable ".\\Shared Variables.lvlib\\mono tick"(w2062, error in=w2063) -> (error out=w2061:errorcluster)
                                n1068 = shared-variable ".\\Shared Variables.lvlib\\Gate Open"(TRUE ("Gate Open"), error in=w2061) -> (error out=w2060:errorcluster)
                                }
                                }
                                n1069 = local write "Present Wavelength"(w2031) -> ()
                                }
                                }
                                n1070 = Unbundle By Name(w2004) -> ("status"=w2005:bool)
                                }
                                frame #1 {
                                n1071 = Unbundle By Name(w2064) -> ("Spec Plot.Wavelength"=w2067:dbl[], "Spec Plot.Int WF"=w2066:dbl[])
                                n1072 = Bundle("Wavelength"=w2067, "Int WF"=w2066) -> (w2065:cluster{"Wavelength":dbl[], "Int WF":dbl[]})  [unwired: 1 in]
                                n1073 = local write "XY Graph"(w2065) -> ()
                                }
                                frame #2 {
                                n1074 = case shown="False" w2068 {
                                frame False {
                                n1075 = Multiply(x="Pause", y=1000.0) -> (x*y=w2070:dbl)
                                n1076 = To Unsigned Long Integer(number=w2070) -> (unsigned 32bit integer=w2072:u32)
                                n1077 = Wait (ms)(milliseconds to wait=w2072) -> ()  [unwired: 1 out]
                                }
                                frame True {
                                n1078 = local read "Pause"() -> (w2077:dbl)
                                n1079 = Multiply(x=w2077, y=1000.0) -> (x*y=w2075:dbl)
                                n1080 = To Unsigned Long Integer(number=w2075) -> (unsigned 32bit integer=w2074:u32)
                                n1081 = Wait (ms)(milliseconds to wait=w2074) -> ()  [unwired: 1 out]
                                }
                                }
                                }
                              }
                              n1082 = local read "End Wavelength"() -> (w1998:dbl)
                              n1083 = Less Or Equal?(x=w1995, y=w1998) -> (x <= y?=w1997:bool)
                              n1084 = Not(x="Abort Scan GL302") -> (.not. x?=w1993:bool)
                              n1085 = Bundle By Name(cluster=w1989, "Spec Plot"=w1990) -> (w1988:T6)
                              n1086 = Compound Arithmetic op=AND(invert w1992, w1993, w1997) -> (w1996:bool)
                            }
                          }
                        }
                      }
                    }
                    n1087 = Unbundle By Name(w1801) -> ("Spec Plot.Wavelength"=w1797:dbl[], "Spec Plot.Int WF"=w1796:dbl[])
                    n1088 = Bundle("Wavelength"=w1797, "Int WF"=w1796) -> (w1795:cluster{"Wavelength":dbl[], "Int WF":dbl[]})  [unwired: 1 in]
                    n1089 = local write "XY Graph"(w1795) -> ()
                  }
                }
              }
              frame #2 {
                n1090 = while {
                  stop <- w2078 continue-if-true
                  n1091 = shared-variable ".\\Shared Variables.lvlib\\iHR550_GL302_scan"() -> (w2078:bool)  [unwired: 1 in, 1 out]
                  n1092 = case shown="True" w2078 {
                    frame False {
                      n1093 = local write "Scan GL302"(FALSE ("Scan GL302")) -> ()
                    }
                    frame True {
                    }
                  }
                }
              }
            }
            n1094 = Unbundle By Name(w1601) -> ("status"=w1598:bool)
            n1095 = case shown="True" w1598 {
              tunnel: [w2080 Control_3."Error Handler"] -> w1602
              frame False {
                n1096 = local read "Log Data"() -> (w2081:bool)
                n1097 = case shown="True" w2081 {
                  tunnel: [Control_3."Idle" Control_3."Log Data"] -> w2080
                  frame False {
                  }
                  frame True {
                  }
                }
              }
              frame True {
              }
            }
          }
          frame "GL302 Step Movement" {
            n1098 = local read "Present Wavelength"() -> (w2089:dbl)
            n1099 = Greater Or Equal?(x=w2089, y=350.0) -> (x >= y?=w2090:bool)
            n1100 = Less Or Equal?(x=w2089, y=990.0) -> (x <= y?=w2091:bool)
            n1101 = And(x=w2091, y=w2090) -> (x .and. y?=w2086:bool)
            n1102 = case shown="False" w2086 {
              tunnel: w2096 -> [w2098 w2118]
              tunnel: [w2097 w2117] -> w2095
              tunnel: w2085 -> [_ w2116]
              frame False {
                n1103 = local read "Present Wavelength"() -> (w2106:dbl)
                n1104 = Greater?(x=w2106, y=990.0) -> (0:w2104:bool)
                n1105 = Less?(x=w2106, y=350.0) -> (x < y?=w2103:bool)
                n1106 = Build Array(w2104, w2103) -> (w2102:bool[])
                n1107 = Search 1D Array(1D array=w2102, element=TRUE, start index (0)=1) -> (index of element=w2099:i32)
                n1108 = case shown="0, Default" w2099 {
                  tunnel: w2098 -> [w2108 w2110 w2112]
                  tunnel: [w2108 w2109 w2111] -> w2097
                  frame 0, Default {
                  }
                  frame 1 {
                    n1109 = call "Display Message to User"("error in (no error)"=w2110) -> ("error out"=w2109:errorcluster)  [unwired: 9 in, 1 out]
                  }
                  frame 2 {
                    n1110 = call "Display Message to User2"("error in (no error)"=w2112) -> ("error out"=w2111:errorcluster)  [unwired: 9 in, 1 out]
                  }
                }
              }
              frame True {
                n1111 = Build Array("fs", "bs", "stop 2") -> (w2121:bool[])
                n1112 = Search 1D Array(1D array=w2121, element=TRUE) -> (index of element=w2113:i32)  [unwired: 1 in]
                n1113 = Increment(x=w2113) -> (x+1=w2114:i32)
                n1114 = case shown="2" w2114 {
                  tunnel: w2118 -> [w2123 w2146 w2163 w2179]
                  tunnel: [w2123 w2145 w2162 w2178] -> w2117
                  tunnel: w2116 -> [_ w2135 w2158 w2177]
                  frame 0, Default {
                  }
                  frame 1 {
                    w2137 = TRUE
                    n1115 = local read "Grating, gr/mm"() -> (w2125:u16)
                    n1116 = local read "delay before read (ms)"() -> (w2124:u32)
                    n1117 = call "nm_string.vi"("error in (no error)"=w2146, "Grating, gr/mm"=w2125, "Wavelength, nm"="Wavelength, nm") -> ("error out"=w2139:errorcluster, "nm_String"=w2143:string)  [unwired: 1 in]
                    n1118 = Concatenate Strings("X" ("string"), w2143, "S" ("string")) -> (w2140:string)
                    n1119 = call "RS232.vi"("read"=FALSE, "milliseconds to wait"=w2124, "error in"=w2139, "write"=w2137, "string to write"=w2140, "VISA  name in"=w2135) -> ("error out"=w2136:errorcluster, "VISA out"=w2138:refnum<visa-resource-name>)  [unwired: 2 out]
                    n1120 = local read "Calibration, nm"() -> (w2131:dbl)
                    n1121 = call "RS232.vi"("read"=w2137, "milliseconds to wait"=w2124, "error in"=w2136, "write"=w2137, "string to write"="X-1?", "VISA  name in"=w2138) -> ("error out"=w2130:errorcluster, "bytes to read"=w2129:u32, "read string"=w2132:string)  [unwired: 1 out]
                    n1122 = call "string_wavelength.vi"("Calibration, nm"=w2131, "Position String"=w2132, "Grating, gr/mm"=w2125, "error in (no error)"=w2130) -> ("Present Wavelength"=w2126:dbl, "error out"=w2145:errorcluster)  [unwired: 1 in]
                    n1123 = call "GL302 Status.vi"("bytes to read"=w2129) -> ("Numeric"=w2127:u32, "String"=w2128:string)  [unwired: 9 in]
                    n1124 = local write "Present Wavelength"(w2126) -> ()
                    n1125 = local write "Status"(w2128) -> ()
                    n1126 = property on="Status" class="Str"("Text.BGColor"=w2127) -> ()  [unwired: 2 in, 2 out]
                  }
                  frame 2 {
                    w2166 = TRUE
                    n1127 = local read "Wavelength, nm"() -> (w2171:dbl)
                    n1128 = local read "Grating, gr/mm"() -> (w2148:u16)
                    n1129 = call "nm_string.vi"("error in (no error)"=w2163, "Grating, gr/mm"=w2148, "Wavelength, nm"=w2171) -> ("error out"=w2164:errorcluster, "nm_String"=w2170:string)  [unwired: 1 in]
                    n1130 = local read "delay before read (ms)"() -> (w2147:u32)
                    n1131 = local read "Backlash Compensation"() -> (w2161:bool)
                    n1132 = Concatenate Strings("X-" ("string"), w2170, "S" ("string")) -> (w2167:string)
                    n1133 = call "RS232.vi"("read"=FALSE, "milliseconds to wait"=w2147, "error in"=w2164, "write"=w2166, "string to write"=w2167, "VISA  name in"=w2158) -> ("error out"=w2160:errorcluster, "VISA out"=w2165:refnum<visa-resource-name>)  [unwired: 2 out]
                    n1134 = case shown="True" w2161 {
                      tunnel: w2160 -> [w2172 w2173]
                      tunnel: [w2172 w2173] -> w2159
                      frame False {
                      }
                      frame True {
                        n1135 = local read "Backlash Compensation"() -> (w2174:dbl)
                        n1136 = local read "Grating, gr/mm"() -> (w2175:u16)
                        n1137 = call "backlash_move.vi"("Grating, gr/mm"=w2175, "Wavelength, nm"=w2174) -> ()  [unwired: 3 in]
                      }
                    }
                    n1138 = local read "Calibration, nm"() -> (w2154:dbl)
                    n1139 = call "RS232.vi"("read"=w2166, "milliseconds to wait"=w2147, "error in"=w2159, "write"=w2166, "string to write"="X-1?", "VISA  name in"=w2165) -> ("error out"=w2153:errorcluster, "bytes to read"=w2152:u32, "read string"=w2155:string)  [unwired: 1 out]
                    n1140 = call "GL302 Status.vi"("bytes to read"=w2152) -> ("Numeric"=w2150:u32, "String"=w2151:string)  [unwired: 9 in]
                    n1141 = call "string_wavelength.vi"("Calibration, nm"=w2154, "Position String"=w2155, "Grating, gr/mm"=w2148, "error in (no error)"=w2153) -> ("Present Wavelength"=w2149:dbl, "error out"=w2162:errorcluster)  [unwired: 1 in]
                    n1142 = local write "Status"(w2151) -> ()
                    n1143 = local write "Present Wavelength"(w2149) -> ()
                    n1144 = property on="Status" class="Str"("Text.BGColor"=w2150) -> ()  [unwired: 2 in, 2 out]
                  }
                  frame 3 {
                    w2180 = TRUE
                    n1145 = call "RS232.vi"("read"=w2180, "milliseconds to wait"=u32 50, "error in"=w2179, "write"=w2180, "string to write"="XZ", "VISA  name in"=w2177) -> ("error out"=w2178:errorcluster)  [unwired: 3 out]
                  }
                }
              }
            }
            n1146 = Unbundle By Name(w2095) -> ("status"=w2094:bool)
            n1147 = case shown="False" w2094 {
              tunnel: [Control_3."Idle" Control_3."Error Handler"] -> w2093
              frame False {
              }
              frame True {
              }
            }
          }
          frame "GL302 Settings" {
            n1148 = Build Array("Set speed", "Calibration", "Save GL302 Settings", "Initialize") -> (w2195:bool[])
            n1149 = Search 1D Array(1D array=w2195, element=TRUE) -> (index of element=w2185:i32)  [unwired: 1 in]
            n1150 = Increment(x=w2185) -> (x+1=w2184:i32)
            n1151 = case shown="3" w2184 {
              tunnel: w2193 -> [w2200 w2204 w2227 w2240 w2254]
              tunnel: [w2200 w2203 w2216 w2230 w2253] -> w2192
              tunnel: w2187 -> [_ w2202 w2215 w2242 w2255]
              frame 0, Default {
              }
              frame 1 {
                w2205 = TRUE
                n1152 = local read "Grating, gr/mm"() -> (w2209:u16)
                n1153 = call "speed_string.vi"("error in (no error)"=w2204, "Grating, gr/mm"=w2209, "Speed"="Speed") -> ("error out"=w2206:errorcluster, "nm_String"=w2207:string, "R number"=→"R number":i32)
                n1154 = call "RS232.vi"("read"=w2205, "milliseconds to wait"=u32 0, "error in"=w2206, "write"=w2205, "string to write"=w2207, "VISA  name in"=w2202) -> ("error out"=w2203:errorcluster)  [unwired: 3 out]
              }
              frame 2 {
                w2225 = TRUE
                n1155 = local read "delay before read (ms)"() -> (w2223:u32)
                n1156 = call "RS232.vi"("read"=w2225, "milliseconds to wait"=u32 0, "error in"=w2227, "write"=w2225, "string to write"="X0=15T", "VISA  name in"=w2215) -> ("error out"=w2224:errorcluster, "VISA out"=w2218:refnum<visa-resource-name>)  [unwired: 2 out]
                n1157 = local read "Calibration, nm"() -> (w2221:dbl)
                n1158 = local read "Grating, gr/mm"() -> (w2220:u16)
                n1159 = call "RS232.vi"("read"=w2225, "milliseconds to wait"=w2223, "error in"=w2224, "write"=w2225, "string to write"="X-1?", "VISA  name in"=w2218) -> ("error out"=w2219:errorcluster, "bytes to read"=w2214:u32, "read string"=w2222:string)  [unwired: 1 out]
                n1160 = call "GL302 Status.vi"("bytes to read"=w2214) -> ("Numeric"=w2212:u32, "String"=w2213:string)  [unwired: 9 in]
                n1161 = call "string_wavelength.vi"("Calibration, nm"=w2221, "Position String"=w2222, "Grating, gr/mm"=w2220, "error in (no error)"=w2219) -> ("Present Wavelength"=w2217:dbl, "error out"=w2216:errorcluster)  [unwired: 1 in]
                n1162 = local write "Status"(w2213) -> ()
                n1163 = local write "Present Wavelength"(w2217) -> ()
                n1164 = property on="Status" class="Str"("Text.BGColor"=w2212) -> ()  [unwired: 2 in, 2 out]
              }
              frame 3 {
                w2239 = TRUE
                n1165 = local read "Communication Port"() -> (w2244:refnum<visa-resource-name>)
                n1166 = local read "Calibration, nm"() -> (w2246:dbl)
                n1167 = local read "Backlash Compensation"() -> (w2248:dbl)
                n1168 = local read "Auto Calibration:"() -> (w2243:bool)
                n1169 = local read "delay before read (ms)"() -> (w2238:u32)
                n1170 = local read "Backlash Compensation"() -> (w2245:bool)
                n1171 = local read "Grating, gr/mm"() -> (w2236:u16)
                n1172 = local read "Speed"() -> (w2247:dbl)
                n1173 = call "Write config.vi"("VISA resource name"=w2244, "Grating, gr/mm"=w2236, "Speed"=w2247, "Delay Before read (ms)"=w2238, "Calibration, nm"=w2246, "Backlash compensation"=w2248, "Backlash"=w2245, "Auto Calibration:"=w2243) -> ()  [unwired: 8 in]
                n1174 = call "RS232.vi"("read"=w2239, "milliseconds to wait"=u32 0, "error in"=w2240, "write"=w2239, "string to write"="123456789e", "VISA  name in"=w2242) -> ("error out"=w2237:errorcluster)  [unwired: 3 out]
                n1175 = flat-sequence {
                  tunnel: w2237 -> [w2252]
                  tunnel: [w2252] -> w2233
                  tunnel: w2236 -> [w2250]
                  frame #0 {
                    n1176 = local read "R number"() -> (w2251:i32)
                    n1177 = call "R speed.vi"("R number"=w2251, "Grating, gr/mm\n   or Dye Laser"=w2250) -> ("Speed"=w2249:dbl)  [unwired: 9 in]
                    n1178 = local write "Speed"(w2249) -> ()
                  }
                }
                n1179 = call "Scan Limits.vi"("Grating, gr/mm\n   or Dye Laser"=w2236) -> ("Min"=w2234:dbl, "Max"=w2235:dbl)  [unwired: 9 in]
                n1180 = property on="Start Wavelength" class="DigNum (strict)"(error in=w2233, "Maximum"=w2235, "Minimum"=w2234) -> (error out=w2232:errorcluster)  [unwired: 1 in, 1 out]
                n1181 = property on="End Wavelength" class="DigNum (strict)"(error in=w2232, "Maximum"=w2235, "Minimum"=w2234) -> (error out=w2231:errorcluster)  [unwired: 1 in, 1 out]
                n1182 = property on="Destination Wavelength" class="DigNum (strict)"(error in=w2231, "Maximum"=w2235, "Minimum"=w2234) -> (error out=w2230:errorcluster)  [unwired: 1 in, 1 out]
              }
              frame 4 {
                n1183 = call <instrlib>:"initialize.vi"() -> ()  [unwired: 3 in]
                n1184 = flat-sequence {
                  tunnel: w2255 -> [w2261]
                  tunnel: w2254 -> [w2259]
                  tunnel: [w2257] -> w2253
                  frame #0 {
                    w2260 = TRUE
                    n1185 = local read "Grating, gr/mm"() -> (w2264:u16)
                    n1186 = local read "Speed"() -> (w2263:dbl)
                    n1187 = call "speed_string.vi"("error in (no error)"=w2259, "Grating, gr/mm"=w2264, "Speed"=w2263) -> ("error out"=w2258:errorcluster, "nm_String"=w2262:string)  [unwired: 1 out]
                    n1188 = call "RS232.vi"("read"=w2260, "milliseconds to wait"=u32 0, "error in"=w2258, "write"=w2260, "string to write"=w2262, "VISA  name in"=w2261) -> ("error out"=w2257:errorcluster)  [unwired: 3 out]
                  }
                }
              }
            }
            n1189 = Unbundle By Name(w2192) -> ("status"=w2191:bool)
            n1190 = case shown="False" w2191 {
              tunnel: [Control_3."Idle" Control_3."Error Handler"] -> w2190
              frame False {
              }
              frame True {
              }
            }
          }
          frame "Close Session" {
            n1191 = VISA Close(VISA resource name=w2265, error in (no error)=w2270) -> (error out=w2269:errorcluster)
            n1192 = Unbundle By Name(w2269) -> ("status"=w2268:bool)
            n1193 = case shown="False" w2268 {
              tunnel: [Control_3."Idle" Control_3."Error Handler"] -> w2267
              frame False {
              }
              frame True {
              }
            }
          }
          frame "iHR550 Front Entrance " {
            n1194 = local read "Entrance Mirror"() -> (w2276:u16)
            n1195 = local read "Current UniqueID"() -> (w2278:string)
            n1196 = call "JYSlits.vi"("JYMONOLib.IJYMonoReqd"=w2279, "Slit"=w2276, "UniqueID"=w2278, "error in (no error)"=w2284, "Slit Width"="Target\nFront Entrance") -> ("JYMONOLib.IJYMonoReqd 2"=w2277:refnum<k7>, "error out"=w2275:errorcluster)
            n1197 = call "JYGetSlits.vi"("MonoRefNum IN"=w2277, "UniqueID"=w2278, "Slit"=w2276, "error in (no error)"=w2275) -> ("Slit Width"=w2273:dbl, "error out"=w2274:errorcluster)  [unwired: 12 in, 2 out]
            n1198 = local write "Front Entrance"(w2273) -> ()
            n1199 = Unbundle By Name(w2274) -> ("status"=w2282:bool)
            n1200 = case shown="False" w2282 {
              tunnel: [Control_3."Idle" Control_3."Error Handler"] -> w2281
              frame False {
              }
              frame True {
              }
            }
          }
          frame "iHR550 Front Exit" {
            n1201 = local read "Current UniqueID"() -> (w2291:string)
            n1202 = local read "Exit Mirror"() -> (w2290:u16)
            n1203 = call "JYSlits.vi"("JYMONOLib.IJYMonoReqd"=w2293, "Slit"=w2290, "UniqueID"=w2291, "error in (no error)"=w2298, "Slit Width"="Target  Exit") -> ("JYMONOLib.IJYMonoReqd 2"=w2292:refnum<k7>, "error out"=w2289:errorcluster)
            n1204 = call "JYGetSlits.vi"("MonoRefNum IN"=w2292, "UniqueID"=w2291, "Slit"=w2290, "error in (no error)"=w2289) -> ("Slit Width"=w2287:dbl, "error out"=w2288:errorcluster)  [unwired: 12 in, 2 out]
            n1205 = local write "Exit"(w2287) -> ()
            n1206 = Unbundle By Name(w2288) -> ("status"=w2296:bool)
            n1207 = case shown="False" w2296 {
              tunnel: [Control_3."Idle" Control_3."Error Handler"] -> w2295
              frame False {
              }
              frame True {
              }
            }
          }
          frame "iHR550 Gratings" {
            n1208 = local read "Target Grating"() -> (w2302:u16)
            n1209 = Increment(x=w2302) -> (x+1=w2301:u16)
            n1210 = call "JYTurret.vi"("error in (no error)"=w2308, "Grating Index"=w2301, "JYMONOLib.IJYMonoReqd"=w2309) -> ("error out"=w2315:errorcluster, "JYMONOLib.IJYMonoReqd 2"=w2314:refnum<k7>)  [unwired: 1 out]
            n1211 = local read "Current UniqueID"() -> (w2303:string)
            n1212 = call "Show Current Grating.vi"("UniqueID"=w2303, "Refnum in"=w2314, "error in (no error)"=w2315) -> ("Grating Index"=w2313:i32, "Current Grating"=w2312:dbl, "Current Blaze"=w2311:string, "Current Description"=w2310:string, "error out"=w2306:errorcluster)  [unwired: 4 in, 4 out]
            n1213 = local write "Current Description"(w2310) -> ()
            n1214 = local write "Current Grating"(w2312) -> ()
            n1215 = local write "Current Blaze"(w2311) -> ()
            n1216 = local write "Grating Index"(w2313) -> ()
            n1217 = Unbundle By Name(w2306) -> ("status"=w2305:bool)
            n1218 = case shown="False" w2305 {
              tunnel: [Control_3."Idle" Control_3."Error Handler"] -> w2304
              frame False {
              }
              frame True {
              }
            }
          }
        }
        n1219 = shared-variable ".\\Shared Variables.lvlib\\Shutdown"() -> (w1079:bool)  [unwired: 1 in, 1 out]
        n1220 = Enqueue Element(queue=w1088, element=w1087, error in (no error)=w1084) -> (queue out=w1086:refnum<queue>, error out=w1083:errorcluster)  [unwired: 1 in, 1 out]
        n1221 = Wait (ms)(milliseconds to wait=u32 12) -> ()  [unwired: 1 out]
      }
      n1222 = call "Scan Limits.vi"("Grating, gr/mm\n   or Dye Laser"="Grating, gr/mm") -> ("Min"=w134:dbl, "Max"=w135:dbl)  [unwired: 9 in]
      n1223 = property on="Start Wavelength" class="DigNum (strict)"("Maximum"=w135, "Minimum"=w134) -> ()  [unwired: 2 in, 2 out]
      n1224 = property on="End Wavelength" class="DigNum (strict)"("Maximum"=w135, "Minimum"=w134) -> ()  [unwired: 2 in, 2 out]
      n1225 = property on="Destination Wavelength" class="DigNum (strict)"("Maximum"=w135, "Minimum"=w134) -> ()  [unwired: 2 in, 2 out]
      n1226 = Release Queue(queue=w145, error in (no error)=w140) -> (error out=w142:errorcluster)  [unwired: 1 in, 2 out]
      n1227 = call <vilib>:"Simple Error Handler.vi"("error in (no error)"=w142) -> ("error out"=→"error out":errorcluster)  [unwired: 4 in, 4 out]
    }
  }
